vi "2D scan Tclk.vi"(0 "HW Config":T12={"SEM X coil"="SEM-X", "SEM Y coil"="SEM-Y", "Detectors"="Detectors", "Det min (V)"=-10.0, "Det max (V)"=10.0, "Eanable COM"=TRUE, "COM port"="COM1", "Detector FIB-NI auto switch"="FIB/port0/line0", "Machine Type"=0, "Machine ID"=""} {"Machine Type" items=["Feiss", "NVision"]}, 1 "Options":T9={"GetInfo"=TRUE, "Set Det A para"=TRUE, "Set WD"=FALSE, "Set Mag"=TRUE, "Set stig"=FALSE, "Set aln"=FALSE, "Display"=TRUE, "Save"=TRUE, "8-bit"=TRUE, "Detector A"=TRUE, "Detector B"=TRUE, "Detector C"=FALSE, "Detector D"=FALSE, "Inverse A"=FALSE, "Inverse B"=FALSE, "Inverse C"=FALSE, "Inverse D"=FALSE, "Inverse PNG"=FALSE, "Freeze"=TRUE, "PNG only"=FALSE, "Upload"=FALSE, "Delete after upload"=FALSE}, 2 "Frame":u8=1 min=1 step=1, 5 "Det Info":T11={"Brightness A"=40.0, "Contrast A"=26.0, "Detector B name"="ESB @ 1.0 kV", "Brightness B"=40.0, "Contrast B"=40.0, "Detector C name"="PMT @ 6.0", "Detector D name"="Detector D"}, 7 "Scan Para":T10={"X resolution"=4096, "Y resolution"=2048, "X center (um)"=0.0, "Y center (um)"=0.0, "X size (V)"=20.0, "X size auto"=TRUE, "X stig"=0.0, "Y stig"=0.0, "X aln"=0.0, "Y aln"=0.0, "Scan rate (Hz)"=10000000, "Oversampling"=10, "Oversampling auto"=TRUE, "Frame line rampdown ratio"=0.1, "Pixel size (nm)"=5.0, "WD"=4.0} {"WD" format="%#_7g"; "Frame line rampdown ratio" min=-1 max=1 step=0.05 format="%.2g"; "Scan rate (Hz)" max=4000000 format="%.2e"}, 9 "Focus Index Options":T2={"Keep aspect ratio"=FALSE, "X Grids"=1, "Y Grids"=1, "Primary X index"=1, "Primary Y index"=1}, 11 "File Info":T8={"File path"=path "E:/Images", "Notes"="", "Save recipe"=FALSE, "Load recipe"=FALSE, "Sample ID"=""}, 13 "Tile index":u8[](array[numeric])=[0, 0], 14 "Milling para":T1={"X resolution"=4096, "Y resolution"=125001, "X offset (um)"=0.0, "Y offset (um)"=0.0, "X center (um)"=0.0, "Y center (um)"=0.0, "X size (um)"=250.0, "Y size (um)"=250.0, "UL-Ang"=90.0, "UR-Ang"=90.0, "Line milling time (s)"=5.0, "Z-step (nm)"=2.0, "Lines auto pause"=1, "Auto pause"=FALSE, "Mill from Bottom"=FALSE, "FIB FOV (um)"=500.0, "Auto Profile"=FALSE, "Mill start from Last"=FALSE, "FIB PID on"=FALSE, "FIB PID reset"=TRUE, "FIB PID measured"=0, "FIB PID target"=0.0, "FIB PID target slope"=0.0, "FIB PID P"=0.001, "FIB PID I"=0.01, "FIB PID D"=0.0, "Emission (uA)"=1.36, "Suppressor (V)"=50.0, "Auto reheat"=FALSE} caption="Milling Parameters" {"Suppressor (V)" step=0.1 format="%.1g"; "Emission (uA)" step=0.1 format="%.2g"; "FIB PID measured" items=["Spec.", "B.D. 1", "B.D. 2", "Mill", "Spec. +"]; "FIB PID target slope" min=-1 max=1 step=0.1; "UR-Ang" format="%.2f"; "UL-Ang" format="%.2f"; "Y offset (um)" step=0.02 format="%.3g"; "X offset (um)" step=1 format="%.3g"; "FIB FOV (um)" format="%.3g"; "Line milling time (s)" format="%.1f"; "Y center (um)" format="%#.3g"; "X center (um)" format="%#.3g"}) -> (3 "Image Focus Index Array":T3, 4 "Info & Status":T7={"AO SampClk.MaxRate"=100000000.0, "AI SampClk.MaxRate"=100000000.0, "AO rate"=10000000.0, "Scan speed"=1, "Detector number"=2, "X min (V)"=-10.0, "X max (V)"=10.0, "X min index"=0, "X max index"=4095, "AO multiline"=128, "Decimating factor"=8, "AvailSampPerChan"=6177088, "AO scan line"=2048, "Total pixels recorded"=8388608, "Total lines scanned"=2048, "Scan time (m)"=0.0, "Scan time (s)"=0.9240575999999999, "Remaining time (m)"=0, "Remaining time (s)"=0, "Specimen I (nA)"=0.0, "Frame"=1, "X tile"=0, "Y tile"=0} {"Frame" min=1 step=1; "Y tile" min=1; "X tile" min=1; "Specimen I (nA)" format="%#.2g"; "AvailSampPerChan" scale=0.0..32000000.0; "Scan time (s)" format="%.3f"; "Total pixels recorded" scale=0.0..250000.0; "Scan speed" scale=1.0..15.0; "AO rate" format="%#_3e"}, 6 "SEM parameters":T5={"Detector A"="Det A", "Detector B"="ESB @ 1.0 kV", "Brightness A"=40.0, "Contrast A"=26.0, "Brightness B"=40.0, "Contrast B"=40.0, "Magnification"=5582.6, "Pixel size"=5.0, "Working distance"=4.0, "EHT"=0.0, "Aperture"=0, "High current mode"=0, "Probe current"=0.0, "Scan rotation"=0.0, "Chamber vac"=0.0, "Gun vac"=0.0, "Beam shift X"=0.0, "Beam shift Y"=0.0, "Stig X"=0.0, "Stig Y"=0.0, "Alignment X"=0.0, "Alignment Y"=0.0, "Stage X"=0.0, "Stage Y"=0.0, "Stage Z"=0.0, "Stage T"=0.0, "Stage R"=0.0, "Stage M"=0.0}, 8 "8-bit over scale":bool[](array[boolean]), 10 "FIB parameters":T6, 15 "Image Focus Index":T4)   [LabVIEW 2018]
uses:
  <vilib>/Utility/error.llb/DialogType.ctl
  <vilib>/DAQmx/write.llb/DAQmx Write (Digital Bool 1Line 1Point).vi
  <vilib>/Analysis/2dsp.llb/Decimate (single shot, DBL).vi
  <vilib>/DAQmx/create/channels.llb/DAQmx Create Channel (DO-Digital Output).vi
  <vilib>/DAQmx/miscellaneous.llb/DAQmx Fill In Error Info.vi
  <instrlib>/niScope/Acquire/niScope Get Scaling Coefficients.vi
  <instrlib>/niFgen/niFgen.llb/niFgen Write Waveform.vi
  <instrlib>/niScope/Acquire/Fetch/niScope Multi Fetch Binary 16.vi
  <vilib>/measure/madcrms.llb/Basic Averaged DC-RMS for 1 Chan.vi
  <vilib>/regexp/Match Regular Expression.xnode
  <vilib>/Analysis/NI_AALPro.lvlib
  <vilib>/measure/NI_MAPro.lvlib
panel:
  in  "Api":refnum<k7>(container)
  in  "Force tclk init":bool
  out "DetB-Scaling":sgl
  out "DetA-Scaling":sgl
  out "DetB-Rate":sgl
  out "DetA-Rate":sgl
  out "8-bit coefficents":sgl[][](array[numeric])
  out "DetC-Io":sgl
  out "DetC-k":sgl
  out "DetD-Io":sgl
  out "DetD-k":sgl
  out "DetB-k":sgl
  out "DetB-Io":sgl
  out "DetA-k":sgl
  out "DetA-Io":sgl
  out "8-bit":bool=TRUE
  out "Screen pixel factor":dbl=0.25
  out "Mag":dbl=5582.6
  out "Runsheet header array":string[](array[string])=["Date", "Time", "Notes", "Detector A", "Detector B", "Detector C", "Detector D", "Detectors", "X resolution", "Y resolution", "Rate (Hz)", "Brightness A (%)", "Contrast A (%)", "Brightness B (%)", "Contrast B (%)", "Magnification", "Pixel size (nm)", "Working Distance (mm)", "EHT (kV)", "Aperture #", "High Current Mode", "Probe Current (A)", "Beam Shift X", "Beam Shift Y", "Stigmation X", "Stigmation Y", "Alignment X", "Alignment Y", "FIB spacing (nm)", "A Img Focus Index", "B Img Focus Index", "C Img Focus Index", "D Img Focus Index", "Temp (F)", "FIB Faraday Cup (nA)", "Specimen I (nA)", "Milling Beam Dump (nA)", "Milling Y voltage (V)", "SEM Specimen I (nA)", "Image Delta X (pix)", "Image Delta Y (pix)", "Image Delta Z"]
  out "Set aln":bool
  out "X aln":sgl
  out "Y aln":sgl
  out "FI scaling":u8=1
  in  "SEM Spec. I (nA)":sgl format="%#.2g"
  out "SW date":string
  out "Image bits":u8=16
  out "error out":errorcluster
  out "Delete after upload":bool
  in  "FI Detector":u16(ring) caption="Detector" items=["A", "B", "C", "D"]
  out "keep aspect ratio":bool=TRUE
  out "Primary Y index":u8 caption="Primary Y"
  out "Primary X index":u8 caption="Primary X"
  out "Y Grids":u8=1
  out "X Grids":u8=1
  out "Timestamp":timestamp=timestamp(3479292891.7167473 s since 1904-01-01)
  out "Upload flags path":path
  out "Upload":bool=TRUE
  out "Sample ID":string
  out "Machine ID":string
  out "Eanable COM":bool
  out "PNG only":bool=TRUE
  out "Eval D":i16[][](graph)
  out "Eval C":i16[][](graph)
  out "Eval B":i16[][](graph)
  out "Eval A":i16[][](graph)
  out "Freeze":bool=TRUE
  out "Detector FIB-NI auto switch":tag="FIB/port0/line0"
  out "GetInfo":bool=TRUE
  out "Set stig":bool
  out "Y stig":sgl
  out "X stig":sgl
  in  "Total time":dbl=0.9240575999999999
  in  "stop":bool=TRUE
  out "Det max (V)":dbl=10.0
  out "Det min (V)":dbl=-10.0
  in  "AvailSampPerChan":u32(slide)=6177088 scale=0.0..1000000.0
  in  "AO scan line":u32=2048
  in  "AO multiline":u32=128
  in  "Decimating factor":u16=8
  in  "Remaining time (m)":u16
  in  "Remaining time (s)":u8
  in  "Scan time (s)":dbl=0.9240575999999999 format="%.3f"
  in  "Scan time (m)":dbl
  in  "Total lines scanned":i32=2048
  in  "Total pixels recorded":i32(slide)=8388608 scale=-1.0..1048576.0
  in  "X max (V)":dbl=10.0
  in  "X min (V)":dbl=-10.0
  in  "X min index":i32
  in  "X max index":i32=4095
  in  "Scan speed":u8(slide)=1 scale=1.0..15.0
  in  "AO rate":dbl=10000000.0 caption="Scanning rate" format="%#_3e"
  in  "Detector number":u8=2
  in  "AI SampClk.MaxRate":dbl=100000000.0
  in  "AO SampClk.MaxRate":dbl=100000000.0
  out "Det A Img":i16[][](graph)
  out "Det B Img":i16[][](graph)
  out "Det C Img":i16[][](graph)
  out "Det D Img":i16[][](graph)
  out "Notes":string
  out "File path":path=path "E:/Images"
  out "Inverse PNG":bool
  out "Inverse D":bool
  out "Inverse C":bool
  out "Inverse B":bool
  out "Inverse A":bool
  out "Detector D":bool
  out "Detector C":bool
  out "Detector B":bool=TRUE
  out "Detector A":bool=TRUE
  out "Save":bool=TRUE
  out "Display":bool=TRUE
  out "Set Mag":bool=TRUE
  out "Set WD":bool
  out "Set Det A para":bool=TRUE
  out "WD":sgl=4.0
  out "Pixel size (nm)":sgl=5.0
  out "Frame line rampdown ratio":sgl=0.1
  out "Oversampling":u32=10
  out "Scan rate (Hz)":u32=10000000
  out "Y resolution":u32=2048
  out "X resolution":u32=4096
  out "Detector D name":string="Detector D"
  out "Detector C name":string="PMT @ 6.0"
  out "Contrast B":dbl=40.0
  out "Brightness B":dbl=40.0
  out "Detector B name":string="ESB @ 1.0 kV"
  out "Contrast A":dbl=26.0
  out "Brightness A":dbl=40.0
  out "COM port":refnum<visa-resource-name>="COM1"
  out "File name":path=path "E:/Images/Y2014/M04/D02/_14-04-02_091451_0-0.dat"
  # "Hardware Configuration"
  # "Detectors Information"
  # "Scanning Parameters"
  # "Direction"
  # "Start\nfrom"
  # "<"
  # "Hz"
  # "Scanning time"
  # "m"
  # "s"
  # "Remaining time"
  # "m"
  # "s"
  # "Det"
  # "Detector A"
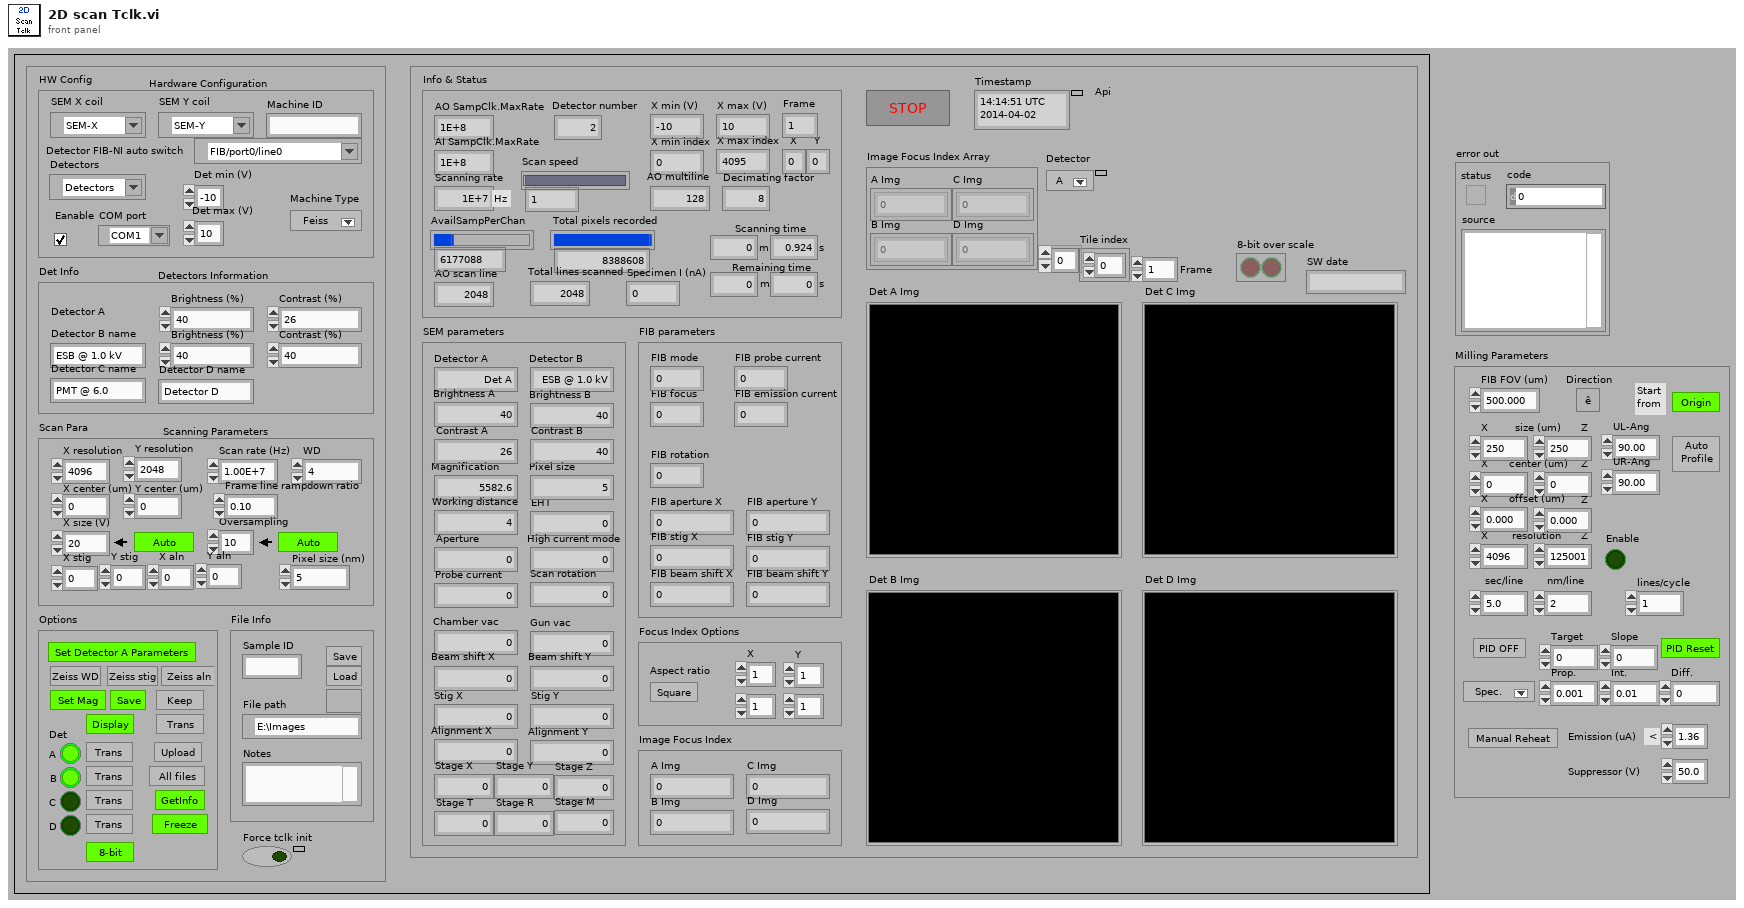
[diagram p1: front panel]
types:
  T1 = cluster{"X resolution":u32, "Y resolution":u32, "X offset (um)":sgl, "Y offset (um)":sgl, "X center (um)":sgl, "Y center (um)":sgl, "X size (um)":sgl, "Y size (um)":sgl, "UL-Ang":sgl, "UR-Ang":sgl, "Line milling time (s)":sgl, "Z-step (nm)":dbl, "Lines auto pause":u16, "Auto pause":bool, "Mill from Bottom":bool, "FIB FOV (um)":sgl, "Auto Profile":bool, "Mill start from Last":bool, "FIB PID on":bool, "FIB PID reset":bool, "FIB PID measured":u8, "FIB PID target":sgl, "FIB PID target slope":sgl, "FIB PID P":sgl, "FIB PID I":sgl, "FIB PID D":sgl, "Emission (uA)":dbl, "Suppressor (V)":sgl, "Auto reheat":bool}
  T2 = cluster{"Keep aspect ratio":bool, "X Grids":u8, "Y Grids":u8, "Primary X index":u8, "Primary Y index":u8}
  T3 = cluster{"A Img Focus Index array":sgl[][], "B Img Focus Index array":sgl[][], "C Img Focus Index array":sgl[][], "D Img Focus Index array":sgl[][]}
  T4 = cluster{"A Img Focus Index":sgl, "B Img Focus Index":sgl, "C Img Focus Index":sgl, "D Img Focus Index":sgl}
  T5 = cluster{"Detector A":string, "Detector B":string, "Brightness A":sgl, "Contrast A":sgl, "Brightness B":sgl, "Contrast B":sgl, "Magnification":sgl, "Pixel size":sgl, "Working distance":sgl, "EHT":sgl, "Aperture":u8, "High current mode":u8, "Probe current":sgl, "Scan rotation":sgl, "Chamber vac":sgl, "Gun vac":sgl, "Beam shift X":sgl, "Beam shift Y":sgl, "Stig X":sgl, "Stig Y":sgl, "Alignment X":sgl, "Alignment Y":sgl, "Stage X":sgl, "Stage Y":sgl, "Stage Z":sgl, "Stage T":sgl, "Stage R":sgl, "Stage M":sgl}
  T6 = cluster{"FIB mode":u8, "FIB focus":sgl, "FIB probe current":sgl, "FIB emission current":sgl, "FIB rotation":sgl, "FIB aperture X":sgl, "FIB aperture Y":sgl, "FIB stig X":sgl, "FIB stig Y":sgl, "FIB beam shift X":sgl, "FIB beam shift Y":sgl}
  T7 = cluster{"AO SampClk.MaxRate":dbl, "AI SampClk.MaxRate":dbl, "AO rate":dbl, "Scan speed":u8, "Detector number":u8, "X min (V)":dbl, "X max (V)":dbl, "X min index":i32, "X max index":i32, "AO multiline":u32, "Decimating factor":u16, "AvailSampPerChan":u32, "AO scan line":u32, "Total pixels recorded":i32, "Total lines scanned":i32, "Scan time (m)":dbl, "Scan time (s)":dbl, "Remaining time (m)":u16, "Remaining time (s)":u8, "Specimen I (nA)":sgl, "Frame":u8, "X tile":u8, "Y tile":u8}
  T8 = cluster{"File path":path, "Notes":string, "Save recipe":bool, "Load recipe":bool, "Sample ID":string}
  T9 = cluster{"GetInfo":bool, "Set Det A para":bool, "Set WD":bool, "Set Mag":bool, "Set stig":bool, "Set aln":bool, "Display":bool, "Save":bool, "8-bit":bool, "Detector A":bool, "Detector B":bool, "Detector C":bool, "Detector D":bool, "Inverse A":bool, "Inverse B":bool, "Inverse C":bool, "Inverse D":bool, "Inverse PNG":bool, "Freeze":bool, "PNG only":bool, "Upload":bool, "Delete after upload":bool}
  T10 = cluster{"X resolution":u32, "Y resolution":u32, "X center (um)":sgl, "Y center (um)":sgl, "X size (V)":dbl, "X size auto":bool, "X stig":sgl, "Y stig":sgl, "X aln":sgl, "Y aln":sgl, "Scan rate (Hz)":u32, "Oversampling":u32, "Oversampling auto":bool, "Frame line rampdown ratio":sgl, "Pixel size (nm)":sgl, "WD":sgl}
  T11 = cluster{"Brightness A":dbl, "Contrast A":dbl, "Detector B name":string, "Brightness B":dbl, "Contrast B":dbl, "Detector C name":string, "Detector D name":string}
  T12 = cluster{"SEM X coil":refnum<k15>, "SEM Y coil":refnum<k15>, "Detectors":refnum<k15>, "Det min (V)":dbl, "Det max (V)":dbl, "Eanable COM":bool, "COM port":refnum<visa-resource-name>, "Detector FIB-NI auto switch":tag, "Machine Type":u8, "Machine ID":string}
  T13 = cluster{"AO SampClk.MaxRate":dbl, "AI SampClk.MaxRate":dbl, "AO rate":dbl, "Scan speed":u8, "Detector number":u8, "X min (V)":dbl, "X max (V)":dbl, "X min index":i32, "X max index":i32, "AO multiline":u32, "Decimating factor":u16, "AvailSampPerChan":u32, "AO scan line":u32, "Total pixels recorded":i32, "Total lines scanned":i32, "Scan time (m)":dbl, "Scan time (s)":dbl, "Remaining time (m)":u16, "Remaining time (s)":u8, "SEM Spec. I (nA)":sgl, "Frame":u8, u8, u8}
  T14 = enum16{"SEM", "FIB", "Milling", "SEM + FIB", "Mill + SEM", "SEM Drift Correction", "FIB Drift Correction", "No Beam", "External", "External + SEM"}
  T15 = enum16{"Initialize Reference", "Get Reference", "Close Reference"}
  T16 = enum16{"open", "replace", "create", "open or create", "replace or create", "replace or create with confirmation"}
  T17 = typedef "DialogType.ctl" = u16
  T18 = cluster{"FIB mode":u8, "FIB focus":sgl, "FIB probe current":u8, "FIB emission current":sgl, "FIB rotation":sgl, "FIB aperture X":sgl, "FIB aperture Y":sgl, "FIB stig X":sgl, "FIB stig Y":sgl, "FIB beam shift X":sgl, "FIB beam shift Y":sgl}
  T19 = cluster{"Latest 8-bit coefficients[0]":sgl, "Latest 8-bit coefficients[1]":sgl, "Latest 8-bit coefficients[2]":sgl, "Latest 8-bit coefficients[3]":sgl, "Latest 8-bit coefficients[4]":sgl, "Latest 8-bit coefficients[5]":sgl, "Latest 8-bit coefficients[6]":sgl, "Latest 8-bit coefficients[7]":sgl}
  T20 = cluster{"sessions out":refnum<k20>[], "SEM-X handle out":refnum<k15>, "SEM-Y handle out":refnum<k15>, "SEM-Y waveform handle out":i32, "Detectors handle out":refnum<k15>, "channels":string, "error out":errorcluster, "Others":cluster{"AO SampClk.MaxRate":dbl, "AI SampClk.MaxRate":dbl, "AO rate":dbl, "Scan speed":u8, "Detector number":u8, "X min (V)":dbl, "X max (V)":dbl, "X min index":i32, "X max index":i32, "Y min (V)":dbl, "Y max (V)":dbl, "AO multiline":u32, "Decimating factor":u16, "Total time":dbl, "Scan time (m)":dbl, "Scan time (s)":dbl, "X resolution":u32, "Y resolution":u32, "X resolution with rampdown":i32, "Oversampling":u32, "Y scan pts per line":i32, "Y scan pts per AO multiline":i32, "Small scan":bool, "Y single line pattern":dbl[], "Detectors min record length":u32, "Waveform blocks":u32, "Repeat count":u32, "Waveform size":u32, "AI multiline":u16}}
  T21 = cluster{"offset":dbl, "gain":dbl, "reserved 1":dbl, "reserved 2":dbl}[]
  T22 = cluster{"offset":sgl, "gain":sgl, "reserved 1":sgl, "reserved 2":sgl}[]
  T23 = cluster{"Detector A":bool, "Detector B":bool, "Detector C":bool, "Detector D":bool}
  T24 = cluster{"Detector C name":string, "Detector D name":string}
  T25 = cluster{"X resolution":u32, "Y resolution":u32, "Oversampling":u32, "Scan speed":u8, "AO rate":dbl, "Frame line rampdown ratio":sgl, "X min (V)":dbl, "X max (V)":dbl, "Det min (V)":dbl, "Det max (V)":dbl}
  T26 = cluster{"A Img Focus Index array":dbl[][], "B Img Focus Index array":dbl[][], "C Img Focus Index array":dbl[][], "D Img Focus Index array":dbl[][]}
  T27 = cluster{"A Img Focus Index":dbl, "B Img Focus Index":dbl, "C Img Focus Index":dbl, "D Img Focus Index":dbl}
  T28 = cluster{"Single":sgl, "Single":sgl, "Single":sgl, "Single":sgl, "Single":sgl, "Single":sgl, "SEM Spec. I (nA)":sgl, "Single":sgl, "D Img Focus Index":dbl, "UInt32":u32}
  T29 = cluster{dbl, "8-bit":bool, "8-bit coefficents":sgl[][], cluster{"Detector A":bool, "Detector B":bool, "Detector C":bool, "Detector D":bool}, cluster{"X resolution":u32, "Y resolution":u32, "Oversampling":u32, "Scan speed":u8, "AO rate":dbl, "Frame line rampdown ratio":sgl, "X min (V)":dbl, "X max (V)":dbl, "Det min (V)":dbl, "Det max (V)":dbl}, "Decimating factor":u16, "Notes":string, cluster{"Detector C name":string, "Detector D name":string}, "SEM parameters":cluster{"Detector A":string, "Detector B":string, "Brightness A":sgl, "Contrast A":sgl, "Brightness B":sgl, "Contrast B":sgl, "Magnification":sgl, "Pixel size":sgl, "Working distance":sgl, "EHT":sgl, "Aperture":u8, "High current mode":u8, "Probe current":sgl, "Scan rotation":sgl, "Chamber vac":sgl, "Gun vac":sgl, "Beam shift X":sgl, "Beam shift Y":sgl, "Stig X":sgl, "Stig Y":sgl, "Alignment X":sgl, "Alignment Y":sgl, "Stage X":sgl, "Stage Y":sgl, "Stage Z":sgl, "Stage T":sgl, "Stage R":sgl, "Stage M":sgl}, "FIB parameters":cluster{"FIB mode":u8, "FIB focus":sgl, "FIB probe current":sgl, "FIB emission current":sgl, "FIB rotation":sgl, "FIB aperture X":sgl, "FIB aperture Y":sgl, "FIB stig X":sgl, "FIB stig Y":sgl, "FIB beam shift X":sgl, "FIB beam shift Y":sgl}, "Milling para":cluster{"X resolution":u32, "Y resolution":u32, "X offset (um)":sgl, "Y offset (um)":sgl, "X center (um)":sgl, "Y center (um)":sgl, "X size (um)":sgl, "Y size (um)":sgl, "UL-Ang":sgl, "UR-Ang":sgl, "Line milling time (s)":sgl, "Z-step (nm)":dbl, "Lines auto pause":u16, "Auto pause":bool, "Mill from Bottom":bool, "FIB FOV (um)":sgl, "Auto Profile":bool, "Mill start from Last":bool, "FIB PID on":bool, "FIB PID reset":bool, "FIB PID measured":u8, "FIB PID target":sgl, "FIB PID target slope":sgl, "FIB PID P":sgl, "FIB PID I":sgl, "FIB PID D":sgl, "Emission (uA)":dbl, "Suppressor (V)":sgl, "Auto reheat":bool}, "Machine ID":string, cluster{"Single":sgl, "Single":sgl, "Single":sgl, "Single":sgl, "Single":sgl, "Single":sgl, "SEM Spec. I (nA)":sgl, "Single":sgl, "D Img Focus Index":dbl, "UInt32":u32}}
  T30 = typedef "imagedata.ctl" = cluster{"image type":i32, "image depth":i32, "image":u8[], "mask":u8[], "colors":u32[], "Rectangle":cluster{"left":i16, "top":i16, "right":i16, "bottom":i16}}
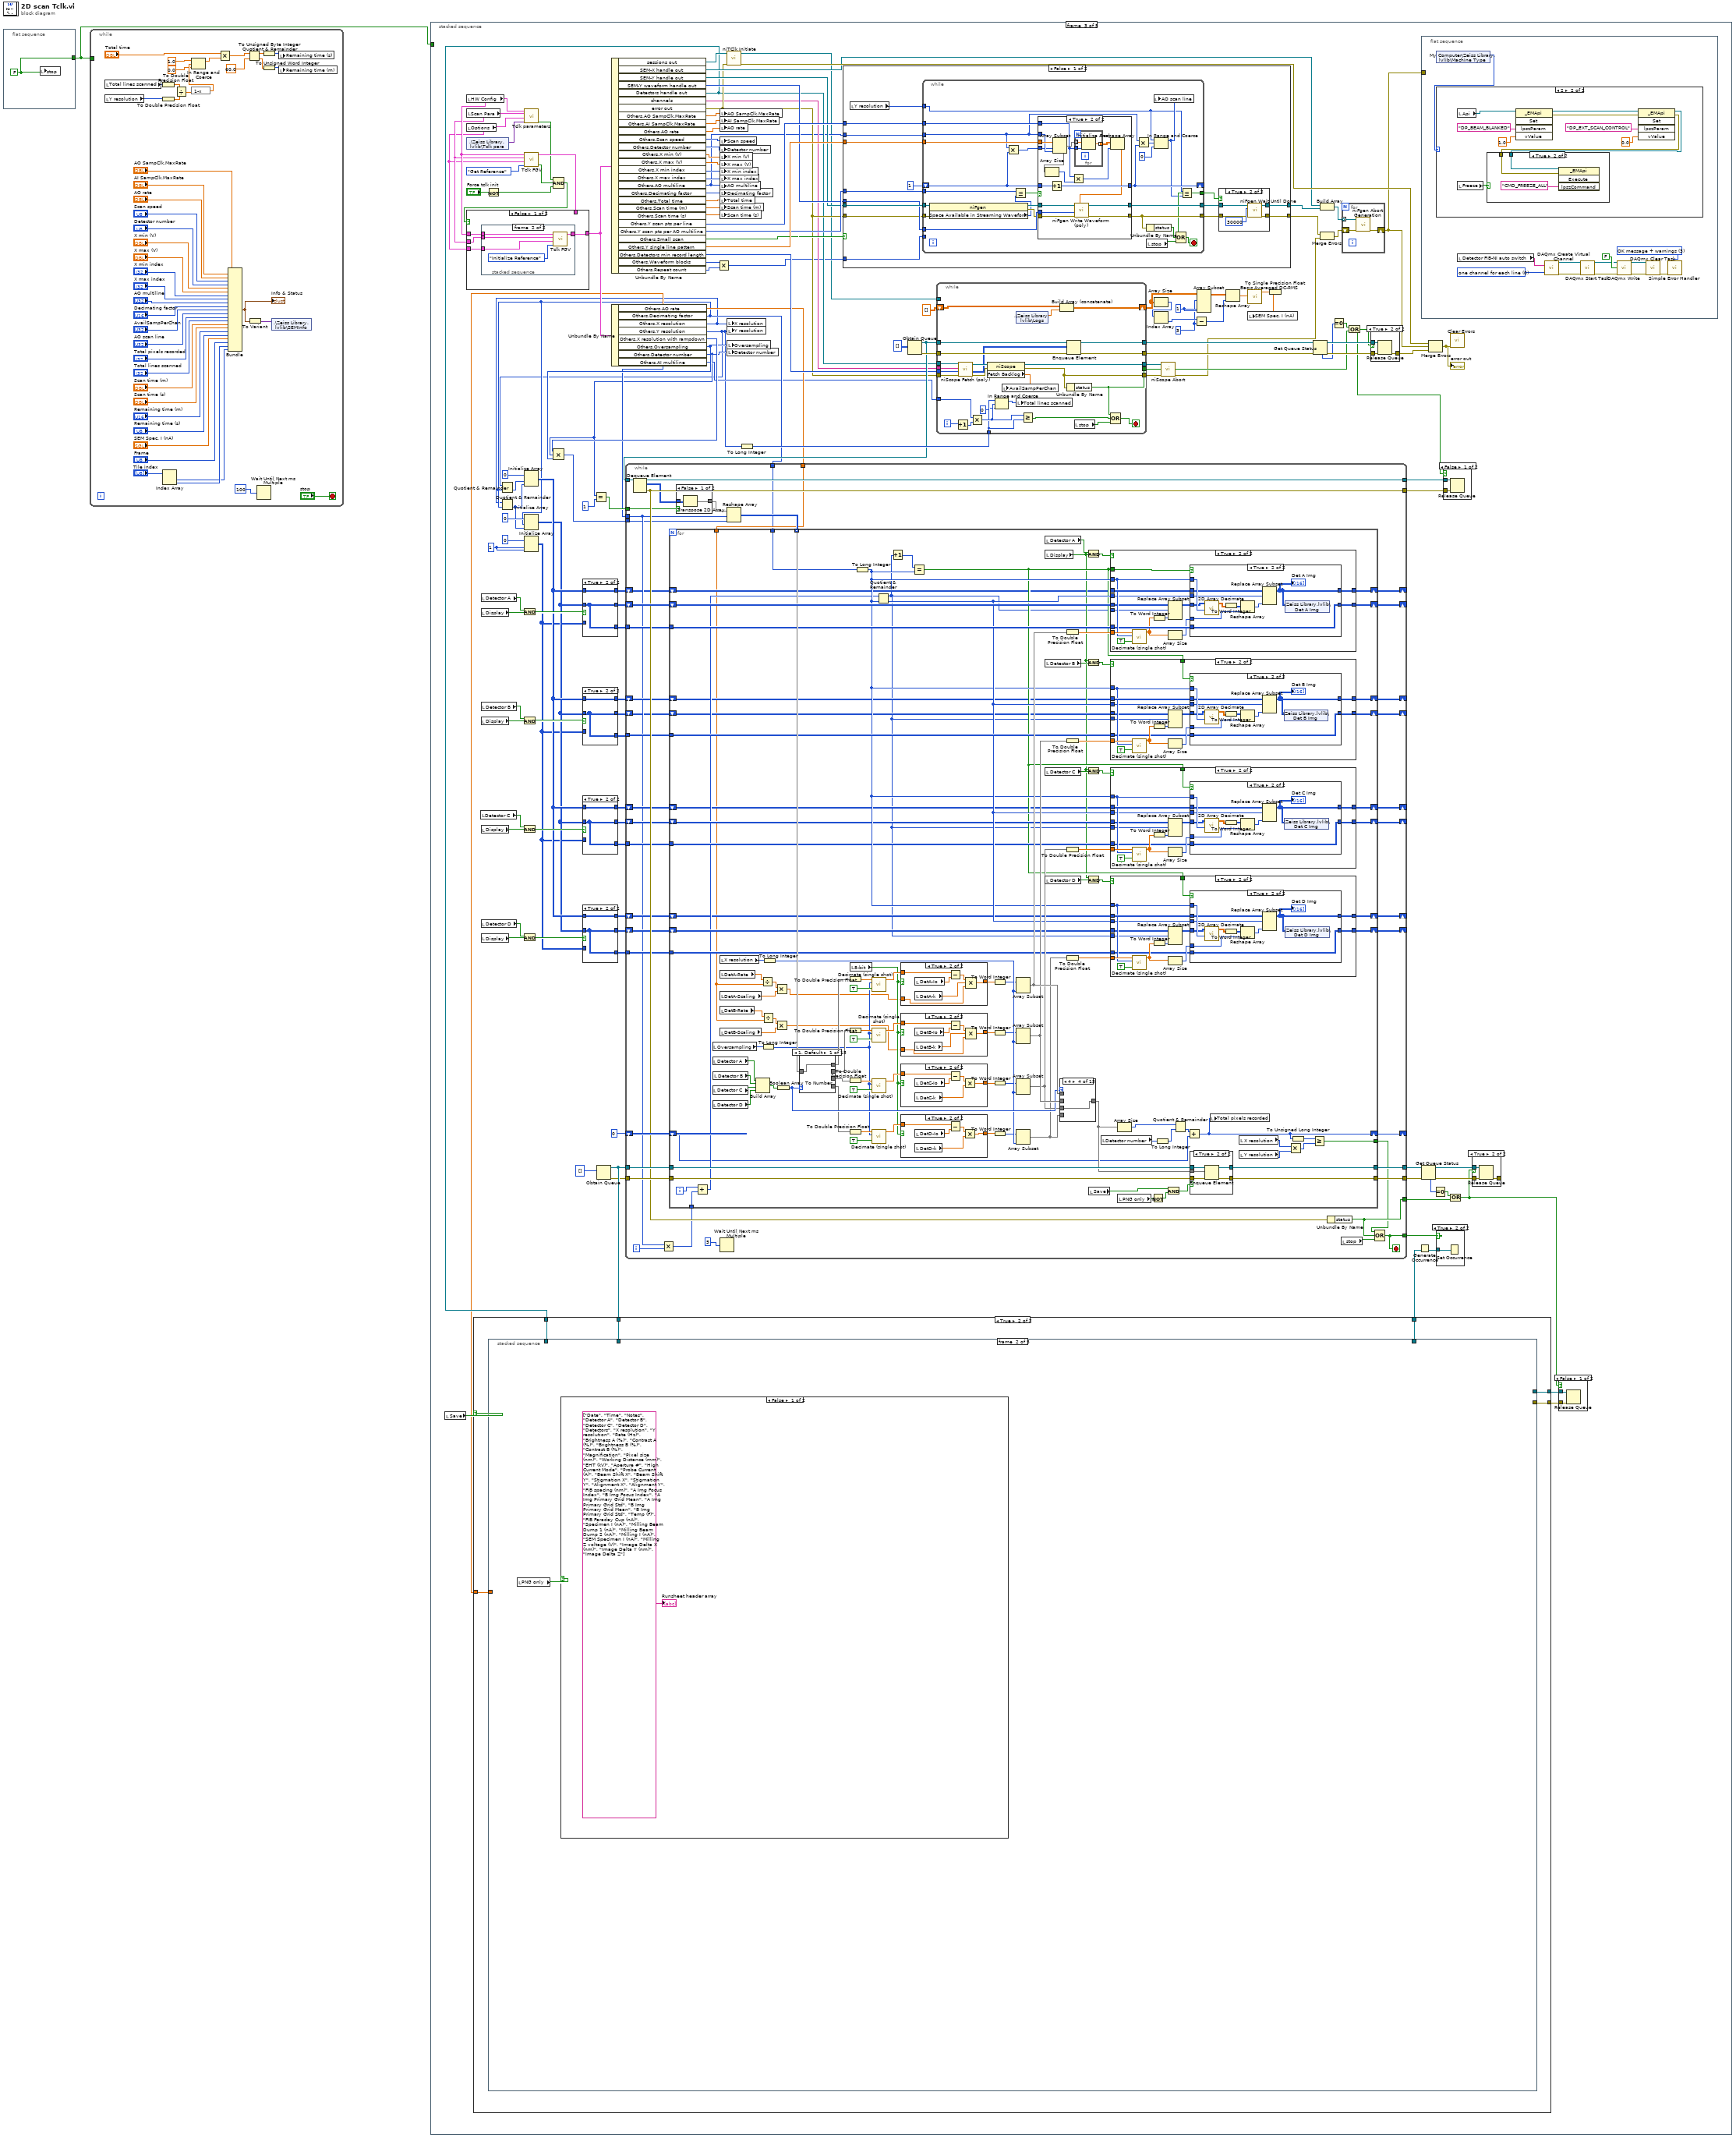
[diagram p0: block diagram]
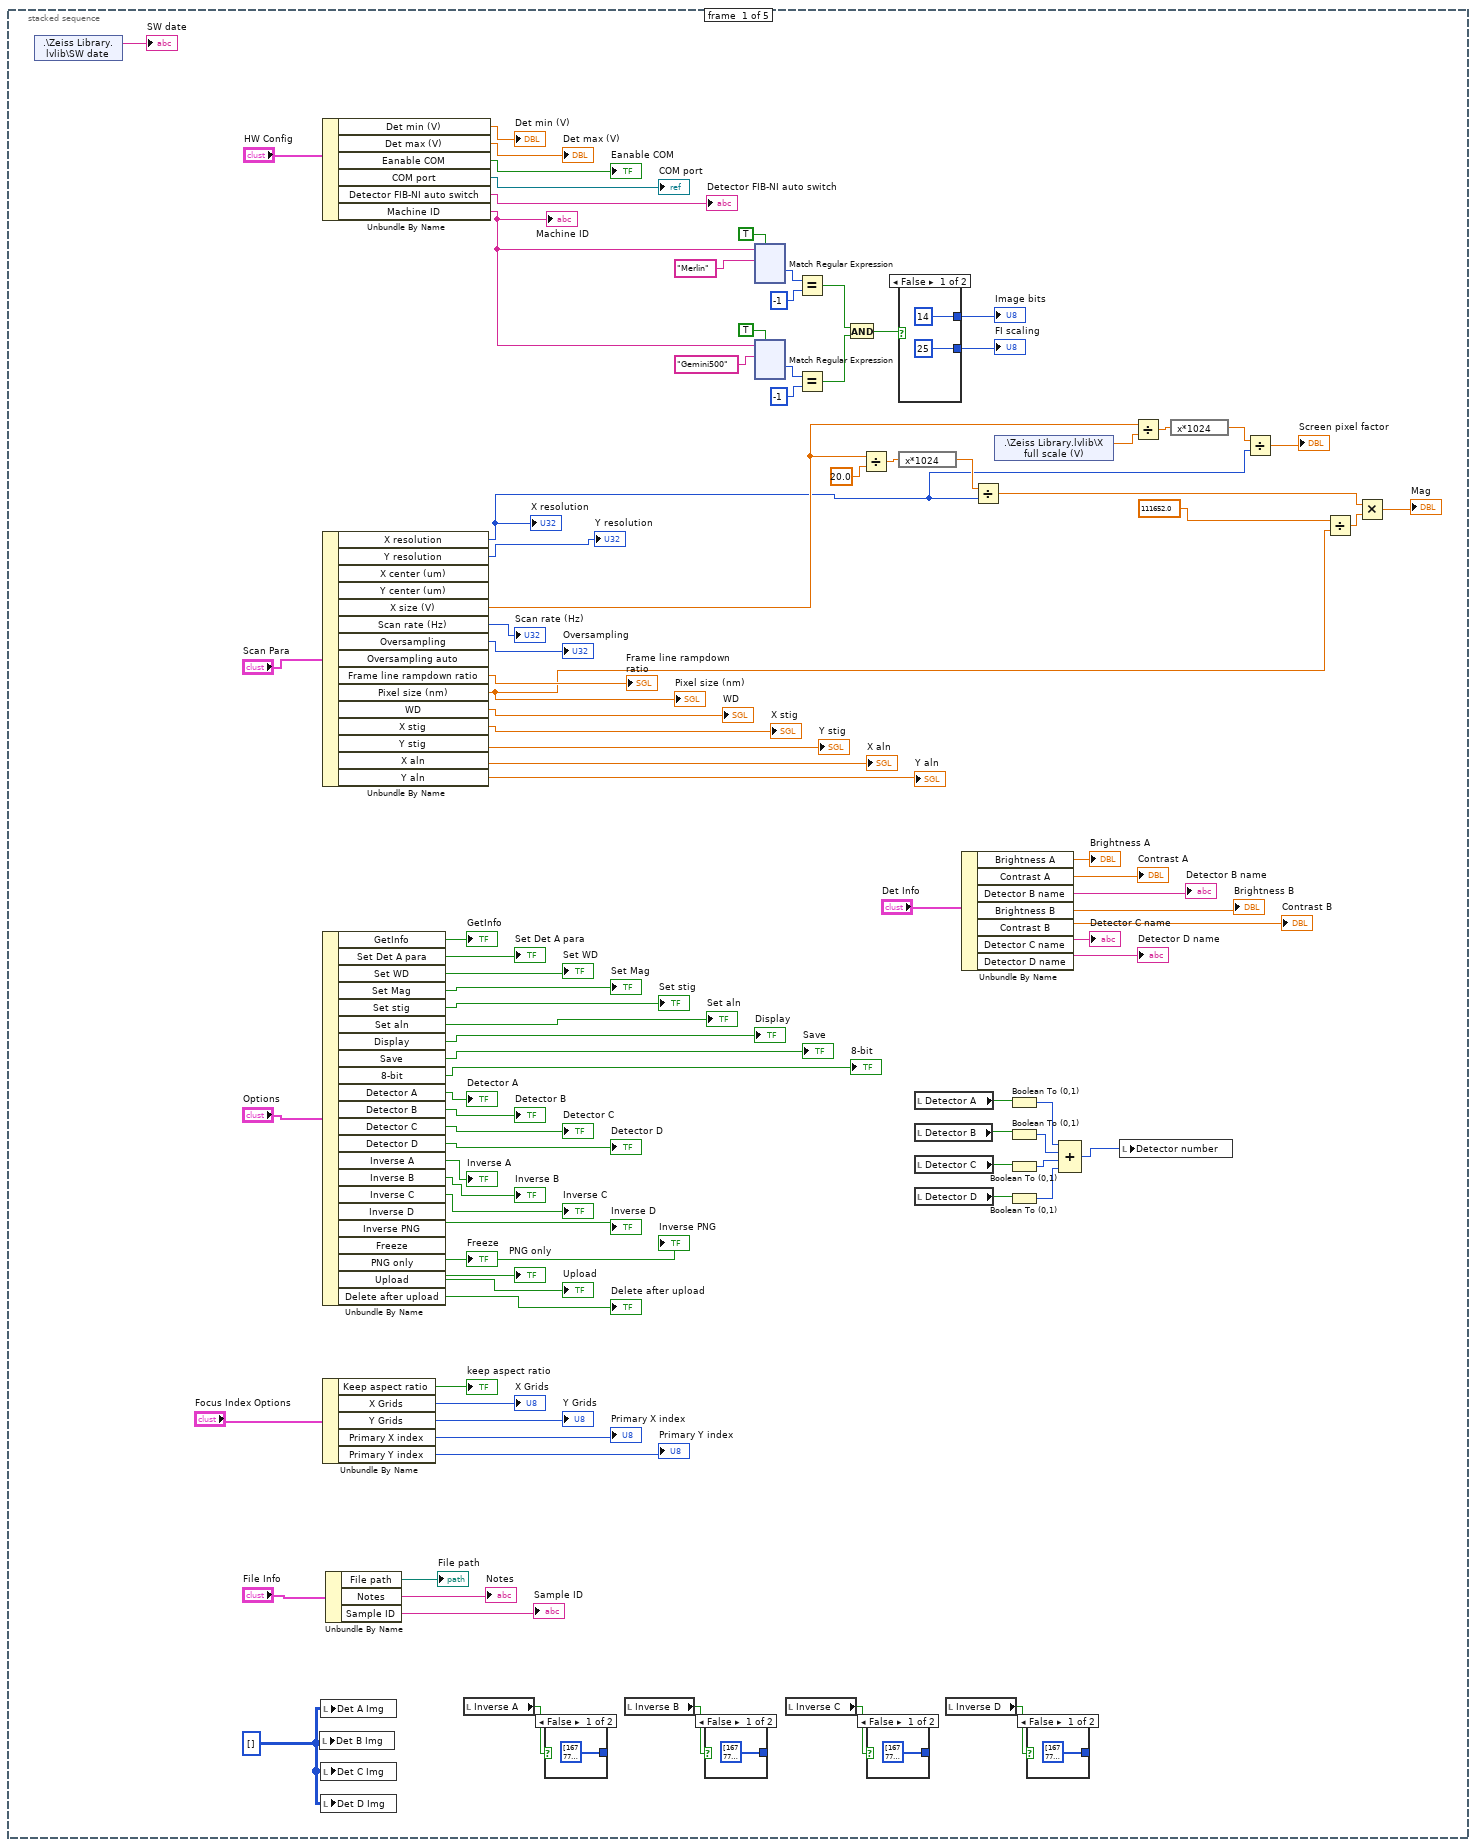
[diagram p2: hidden frame]
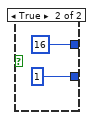
[diagram p3: hidden frame]
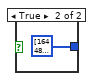
[diagram p4: hidden frame]
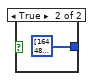
[diagram p5: hidden frame]
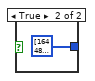
[diagram p6: hidden frame]
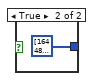
[diagram p7: hidden frame]
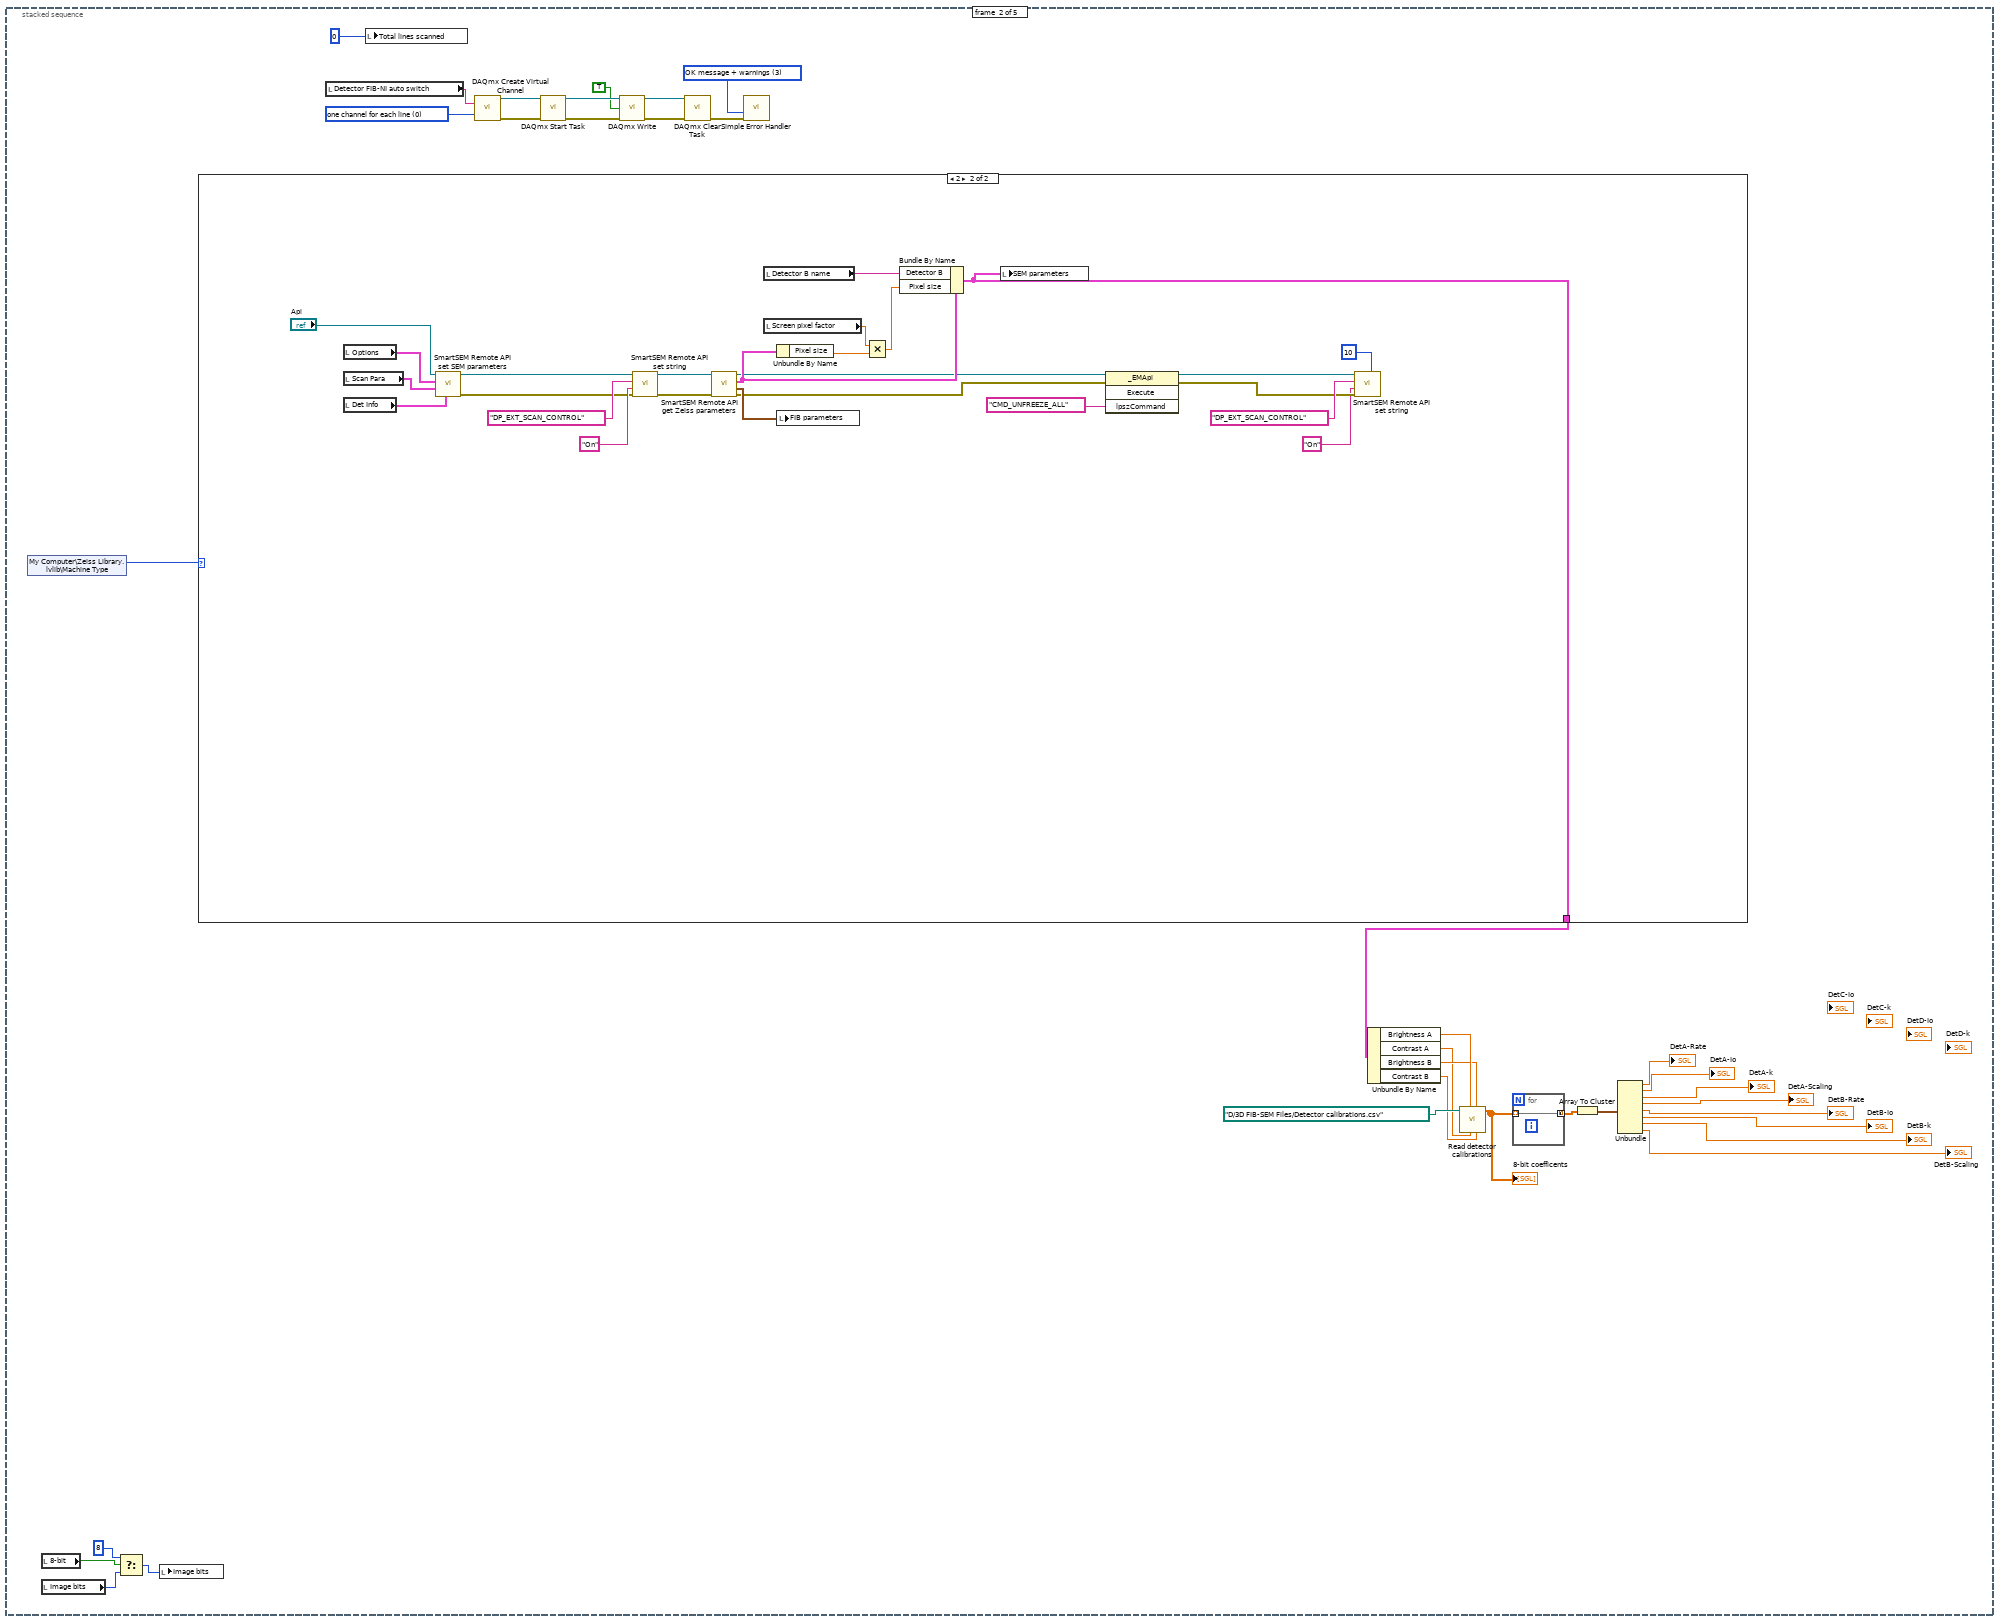
[diagram p8: hidden frame]
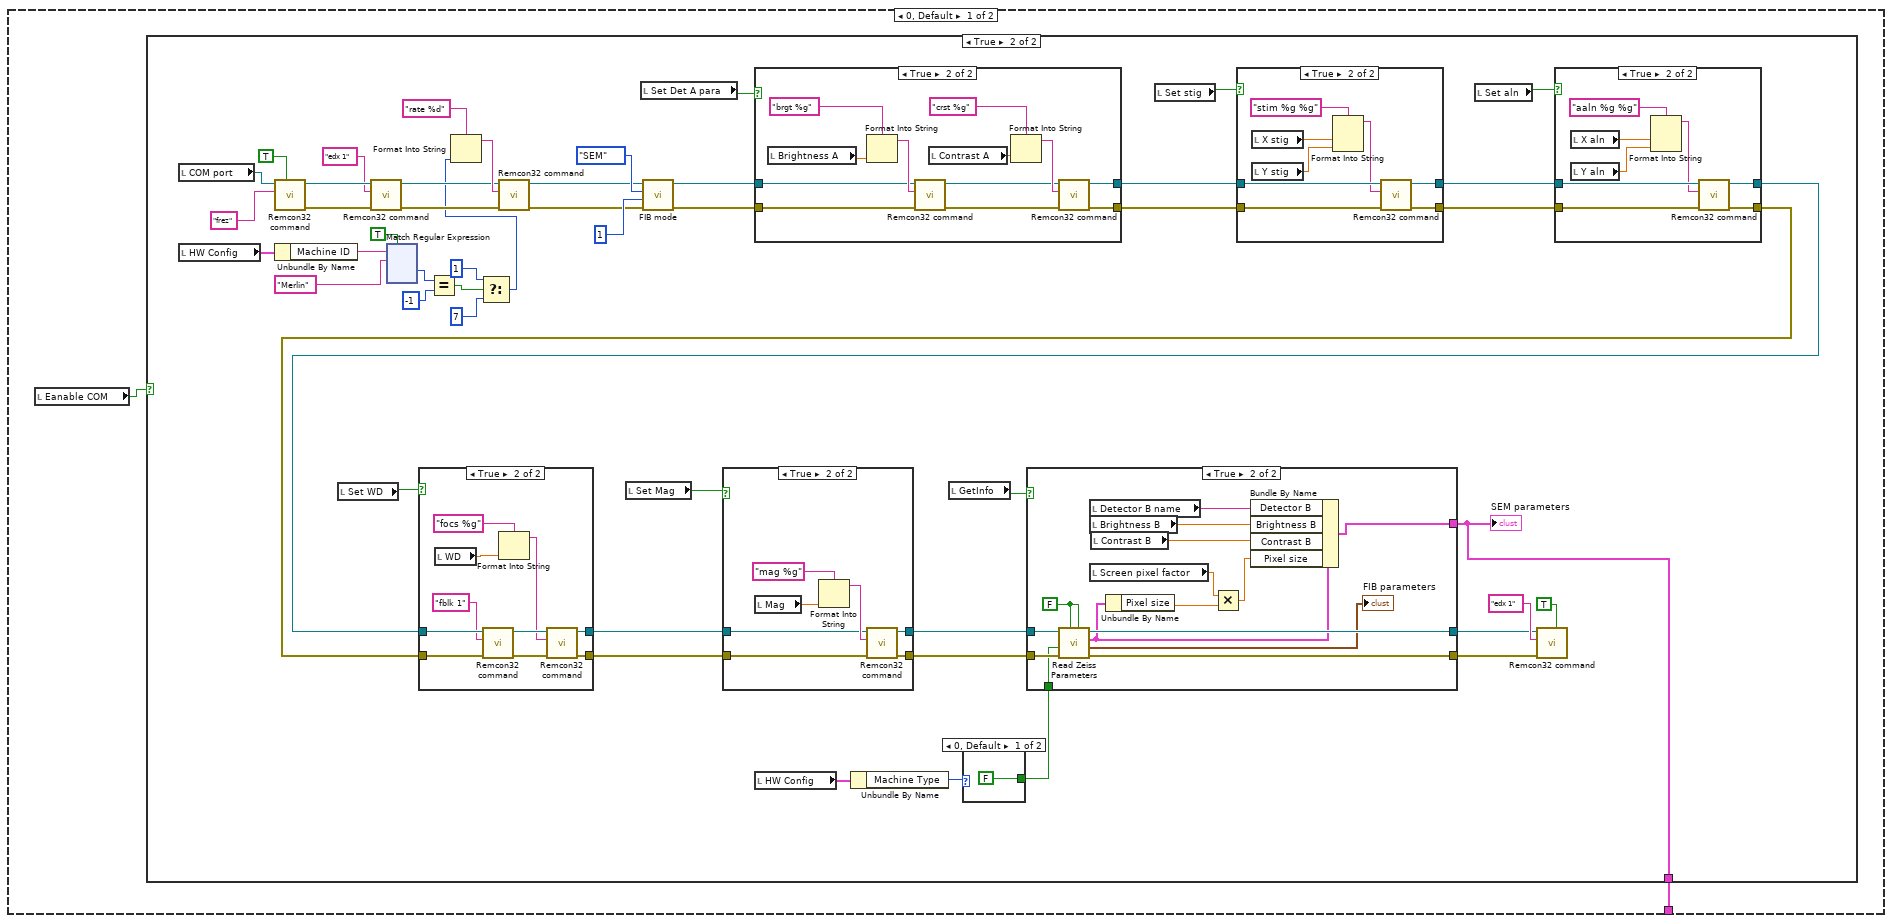
[diagram p9: hidden frame]
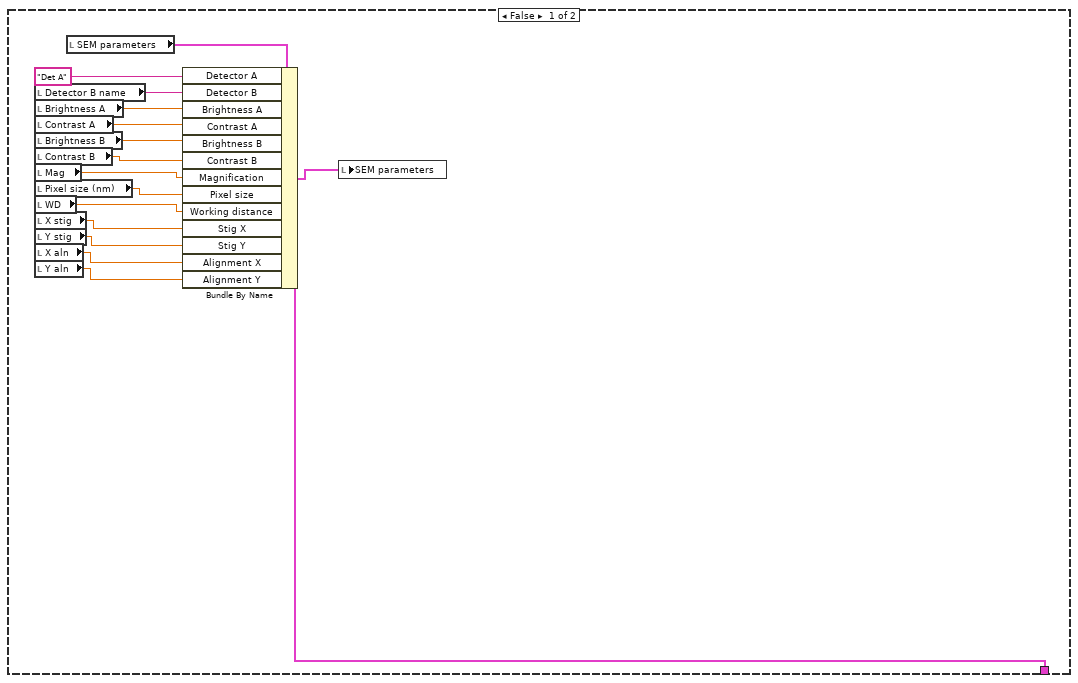
[diagram p10: hidden frame]
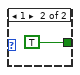
[diagram p12: hidden frame]
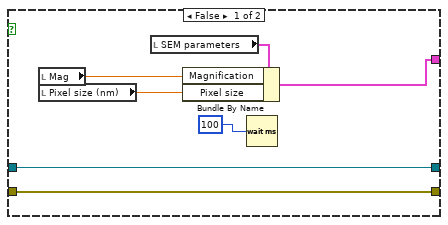
[diagram p13: hidden frame]
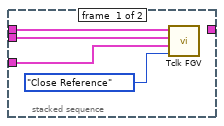
[diagram p18: hidden frame]
diagram:
  n1 = flat-sequence {
    tunnel: [w2] -> w1
    frame #0 {
      w2 = FALSE ("stop")
      n2 = local write "stop"(w2) -> ()
    }
  }
  n3 = while {
    tunnel: w1 -> [_]
    stop <- "stop" stop-if-true
    n4 = local read "Total lines scanned"() -> (w27:i32)
    n5 = local read "Y resolution"() -> (w16:u32)
    n6 = To Double Precision Float(number=w27) -> (double precision float=w20:dbl)
    n7 = To Double Precision Float(number=w16) -> (double precision float=w21:dbl)
    n8 = Index Array(array="Tile index") -> (element #1=w6:u8, element #2=w7:u8)  [unwired: 2 in]
    n9 = Divide(x=w20, y=w21) -> (x/y=w26:dbl)
    n10 = expression code="1-x"(w26) -> (w13:dbl)
    n11 = In Range and Coerce(upper limit=1.0, x=w13, lower limit=0.0) -> (coerced(x)=w10:dbl)  [unwired: 1 out]
    n12 = Multiply(x="Total time", y=w10) -> (x*y=w22:dbl)
    n13 = Bundle("AO SampClk.MaxRate"="AO SampClk.MaxRate", "AI SampClk.MaxRate"="AI SampClk.MaxRate", "AO rate"="AO rate", "Scan speed"="Scan speed", "Detector number"="Detector number", "X min (V)"="X min (V)", "X max (V)"="X max (V)", "X min index"="X min index", "X max index"="X max index", "AO multiline"="AO multiline", "Decimating factor"="Decimating factor", "AvailSampPerChan"="AvailSampPerChan", "AO scan line"="AO scan line", "Total pixels recorded"="Total pixels recorded", "Total lines scanned"="Total lines scanned", "Scan time (m)"="Scan time (m)", "Scan time (s)"="Scan time (s)", "Remaining time (m)"="Remaining time (m)", "Remaining time (s)"="Remaining time (s)", "SEM Spec. I (nA)"="SEM Spec. I (nA)", "Frame"="Frame", w7, w6) -> (w14:T13)  [unwired: 1 out]
    "Info & Status" <- w14
    n14 = Quotient & Remainder(x=w22, y=60.0) -> (x-y*floor(x/y)=w25:dbl, floor(x/y)=w24:dbl)
    n15 = To Variant(anything=w14) -> (Variant=w15:variant)
    n16 = Wait Until Next ms Multiple(millisecond multiple=u32 100) -> ()  [unwired: 1 out]
    n17 = To Unsigned Byte Integer(number=w25) -> (unsigned 8bit integer=w18:u8)
    n18 = To Unsigned Word Integer(number=w24) -> (unsigned 16bit integer=w19:u16)
    n19 = shared-variable ".\\Zeiss Library.lvlib\\SEMInfo"(w15) -> ()  [unwired: 2 out]
    n20 = local write "Remaining time (s)"(w18) -> ()
    n21 = local write "Remaining time (m)"(w19) -> ()
  }
  n22 = stacked-sequence {
    tunnel: w1 -> [_ _ _ _ _]
    frame #0 {
      w133 = i16[][] [] ("SEM")
      n23 = shared-variable ".\\Zeiss Library.lvlib\\SW date"() -> (→"SW date":string)  [unwired: 1 in, 1 out]
      n24 = local write "Det B Img"(w133) -> ()
      n25 = local write "Det A Img"(w133) -> ()
      n26 = local write "Det C Img"(w133) -> ()
      n27 = local write "Det D Img"(w133) -> ()
      n28 = Unbundle By Name("HW Config") -> ("Det min (V)"=→"Det min (V)":dbl, "Det max (V)"=→"Det max (V)":dbl, "Eanable COM"=→"Eanable COM":bool, "COM port"=→"COM port":refnum<visa-resource-name>, "Detector FIB-NI auto switch"=→"Detector FIB-NI auto switch":tag, "Machine ID"=w60:string)
      "Machine ID" <- w60
      n29 = Unbundle By Name("Scan Para") -> ("X resolution"=w48:u32, "Y resolution"=→"Y resolution":u32, "X size (V)"=w51:dbl, "Scan rate (Hz)"=→"Scan rate (Hz)":u32, "Oversampling"=→"Oversampling":u32, "Frame line rampdown ratio"=→"Frame line rampdown ratio":sgl, "Pixel size (nm)"=w71:sgl, "WD"=→"WD":sgl, "X stig"=→"X stig":sgl, "Y stig"=→"Y stig":sgl, "X aln"=→"X aln":sgl, "Y aln"=→"Y aln":sgl)  [unwired: 3 out]
      "X resolution" <- w48
      "Pixel size (nm)" <- w71
      n30 = Unbundle By Name("Options") -> ("GetInfo"=→"GetInfo":bool, "Set Det A para"=→"Set Det A para":bool, "Set WD"=→"Set WD":bool, "Set Mag"=→"Set Mag":bool, "Set stig"=→"Set stig":bool, "Set aln"=→"Set aln":bool, "Display"=→"Display":bool, "Save"=→"Save":bool, "8-bit"=→"8-bit":bool, "Detector A"=→"Detector A":bool, "Detector B"=→"Detector B":bool, "Detector C"=→"Detector C":bool, "Detector D"=→"Detector D":bool, "Inverse A"=→"Inverse A":bool, "Inverse B"=→"Inverse B":bool, "Inverse C"=→"Inverse C":bool, "Inverse D"=→"Inverse D":bool, "Inverse PNG"=→"Inverse PNG":bool, "Freeze"=→"Freeze":bool, "PNG only"=→"PNG only":bool, "Upload"=→"Upload":bool, "Delete after upload"=→"Delete after upload":bool)
      n31 = Unbundle By Name("Focus Index Options") -> ("Keep aspect ratio"=→"keep aspect ratio":bool, "X Grids"=→"X Grids":u8, "Y Grids"=→"Y Grids":u8, "Primary X index"=→"Primary X index":u8, "Primary Y index"=→"Primary Y index":u8)
      n32 = Unbundle By Name("File Info") -> ("File path"=→"File path":path, "Notes"=→"Notes":string, "Sample ID"=→"Sample ID":string)
      n33 = local read "Inverse A"() -> (w143:bool)
      n34 = case shown="False" w143 {
        tunnel: [u32[] [16777222, 65793, 131586, 197379, 263172, 328965, 394758, 460551, 526344, 592137, 657930, 723723, 789516, 855309, 921102, 986895, 1052688, 1118481, 1184274, 1250067, 1315860, 1381653, 1447446, 1513239, 1579032, 1644825, 1710618, 1776411, 1842204, 1907997, 1973790, 2039583, 2105376, 2171169, 2236962, 2302755, 2368548, 2434341, 2500134, 2565927, 2631720, 2697513, 2763306, 2829099, 2894892, 2960685, 3026478, 3092271, 3158064, 3223857, 3289650, 3355443, 3421236, 3487029, 3552822, 3618615, 3684408, 3750201, 3815994, 3881787, 3947580, 4013373, 4079166, 4144959, 4210752, 4276545, 4342338, 4408131, 4473924, 4539717, 4605510, 4671303, 4737096, 4802889, 4868682, 4934475, 5000268, 5066061, 5131854, 5197647, 5263440, 5329233, 5395026, 5460819, 5526612, 5592405, 5658198, 5723991, 5789784, 5855577, 5921370, 5987163, 6052956, 6118749, 6184542, 6250335, 6316128, 6381921, 6447714, 6513507, 6579300, 6645093, 6710886, 6776679, 6842472, 6908265, 6974058, 7039851, 7105644, 7171437, 7237230, 7303023, 7368816, 7434609, 7500402, 7566195, 7631988, 7697781, 7763574, 7829367, 7895160, 7960953, 8026746, 8092539, 8158332, 8224125, 8289918, 8355711, 8421504, 8487297, 8553090, 8618883, 8684676, 8750469, 8816262, 8882055, 8947848, 9013641, 9079434, 9145227, 9211020, 9276813, 9342606, 9408399, 9474192, 9539985, 9605778, 9671571, 9737364, 9803157, 9868950, 9934743, 10000536, 10066329, 10132122, 10197915, 10263708, 10329501, 10395294, 10461087, 10526880, 10592673, 10658466, 10724259, 10790052, 10855845, 10921638, 10987431, 11053224, 11119017, 11184810, 11250603, 11316396, 11382189, 11447982, 11513775, 11579568, 11645361, 11711154, 11776947, 11842740, 11908533, 11974326, 12040119, 12105912, 12171705, 12237498, 12303291, 12369084, 12434877, 12500670, 12566463, 12632256, 12698049, 12763842, 12829635, 12895428, 12961221, 13027014, 13092807, 13158600, 13224393, 13290186, 13355979, 13421772, 13487565, 13553358, 13619151, 13684944, 13750737, 13816530, 13882323, 13948116, 14013909, 14079702, 14145495, 14211288, 14277081, 14342874, 14408667, 14474460, 14540253, 14606046, 14671839, 14737632, 14803425, 14869218, 14935011, 15000804, 15066597, 15132390, 15198183, 15263976, 15329769, 15395562, 15461355, 15527148, 15592941, 15658734, 15724527, 15790320, 15856113, 15921906, 15987699, 16053492, 16119285, 16185078, 16250871, 16316664, 16382457, 16448250, 16514043, 16579836, 16645629, 16711422, 16448250] ("256 gray scale") u32[] [16448250, 16711422, 16645629, 16579836, 16514043, 16448250, 16382457, 16316664, 16250871, 16185078, 16119285, 16053492, 15987699, 15921906, 15856113, 15790320, 15724527, 15658734, 15592941, 15527148, 15461355, 15395562, 15329769, 15263976, 15198183, 15132390, 15066597, 15000804, 14935011, 14869218, 14803425, 14737632, 14671839, 14606046, 14540253, 14474460, 14408667, 14342874, 14277081, 14211288, 14145495, 14079702, 14013909, 13948116, 13882323, 13816530, 13750737, 13684944, 13619151, 13553358, 13487565, 13421772, 13355979, 13290186, 13224393, 13158600, 13092807, 13027014, 12961221, 12895428, 12829635, 12763842, 12698049, 12632256, 12566463, 12500670, 12434877, 12369084, 12303291, 12237498, 12171705, 12105912, 12040119, 11974326, 11908533, 11842740, 11776947, 11711154, 11645361, 11579568, 11513775, 11447982, 11382189, 11316396, 11250603, 11184810, 11119017, 11053224, 10987431, 10921638, 10855845, 10790052, 10724259, 10658466, 10592673, 10526880, 10461087, 10395294, 10329501, 10263708, 10197915, 10132122, 10066329, 10000536, 9934743, 9868950, 9803157, 9737364, 9671571, 9605778, 9539985, 9474192, 9408399, 9342606, 9276813, 9211020, 9145227, 9079434, 9013641, 8947848, 8882055, 8816262, 8750469, 8684676, 8618883, 8553090, 8487297, 8421504, 8355711, 8289918, 8224125, 8158332, 8092539, 8026746, 7960953, 7895160, 7829367, 7763574, 7697781, 7631988, 7566195, 7500402, 7434609, 7368816, 7303023, 7237230, 7171437, 7105644, 7039851, 6974058, 6908265, 6842472, 6776679, 6710886, 6645093, 6579300, 6513507, 6447714, 6381921, 6316128, 6250335, 6184542, 6118749, 6052956, 5987163, 5921370, 5855577, 5789784, 5723991, 5658198, 5592405, 5526612, 5460819, 5395026, 5329233, 5263440, 5197647, 5131854, 5066061, 5000268, 4934475, 4868682, 4802889, 4737096, 4671303, 4605510, 4539717, 4473924, 4408131, 4342338, 4276545, 4210752, 4144959, 4079166, 4013373, 3947580, 3881787, 3815994, 3750201, 3684408, 3618615, 3552822, 3487029, 3421236, 3355443, 3289650, 3223857, 3158064, 3092271, 3026478, 2960685, 2894892, 2829099, 2763306, 2697513, 2631720, 2565927, 2500134, 2434341, 2368548, 2302755, 2236962, 2171169, 2105376, 2039583, 1973790, 1907997, 1842204, 1776411, 1710618, 1644825, 1579032, 1513239, 1447446, 1381653, 1315860, 1250067, 1184274, 1118481, 1052688, 986895, 921102, 855309, 789516, 723723, 657930, 592137, 526344, 460551, 394758, 328965, 263172, 197379, 131586, 65793, 16777222] ("256 gray scale inverse")] -> _
        frame False {
        }
        frame True {
        }
      }
      n35 = local read "Inverse B"() -> (w144:bool)
      n36 = case shown="False" w144 {
        tunnel: [u32[] [16777222, 65793, 131586, 197379, 263172, 328965, 394758, 460551, 526344, 592137, 657930, 723723, 789516, 855309, 921102, 986895, 1052688, 1118481, 1184274, 1250067, 1315860, 1381653, 1447446, 1513239, 1579032, 1644825, 1710618, 1776411, 1842204, 1907997, 1973790, 2039583, 2105376, 2171169, 2236962, 2302755, 2368548, 2434341, 2500134, 2565927, 2631720, 2697513, 2763306, 2829099, 2894892, 2960685, 3026478, 3092271, 3158064, 3223857, 3289650, 3355443, 3421236, 3487029, 3552822, 3618615, 3684408, 3750201, 3815994, 3881787, 3947580, 4013373, 4079166, 4144959, 4210752, 4276545, 4342338, 4408131, 4473924, 4539717, 4605510, 4671303, 4737096, 4802889, 4868682, 4934475, 5000268, 5066061, 5131854, 5197647, 5263440, 5329233, 5395026, 5460819, 5526612, 5592405, 5658198, 5723991, 5789784, 5855577, 5921370, 5987163, 6052956, 6118749, 6184542, 6250335, 6316128, 6381921, 6447714, 6513507, 6579300, 6645093, 6710886, 6776679, 6842472, 6908265, 6974058, 7039851, 7105644, 7171437, 7237230, 7303023, 7368816, 7434609, 7500402, 7566195, 7631988, 7697781, 7763574, 7829367, 7895160, 7960953, 8026746, 8092539, 8158332, 8224125, 8289918, 8355711, 8421504, 8487297, 8553090, 8618883, 8684676, 8750469, 8816262, 8882055, 8947848, 9013641, 9079434, 9145227, 9211020, 9276813, 9342606, 9408399, 9474192, 9539985, 9605778, 9671571, 9737364, 9803157, 9868950, 9934743, 10000536, 10066329, 10132122, 10197915, 10263708, 10329501, 10395294, 10461087, 10526880, 10592673, 10658466, 10724259, 10790052, 10855845, 10921638, 10987431, 11053224, 11119017, 11184810, 11250603, 11316396, 11382189, 11447982, 11513775, 11579568, 11645361, 11711154, 11776947, 11842740, 11908533, 11974326, 12040119, 12105912, 12171705, 12237498, 12303291, 12369084, 12434877, 12500670, 12566463, 12632256, 12698049, 12763842, 12829635, 12895428, 12961221, 13027014, 13092807, 13158600, 13224393, 13290186, 13355979, 13421772, 13487565, 13553358, 13619151, 13684944, 13750737, 13816530, 13882323, 13948116, 14013909, 14079702, 14145495, 14211288, 14277081, 14342874, 14408667, 14474460, 14540253, 14606046, 14671839, 14737632, 14803425, 14869218, 14935011, 15000804, 15066597, 15132390, 15198183, 15263976, 15329769, 15395562, 15461355, 15527148, 15592941, 15658734, 15724527, 15790320, 15856113, 15921906, 15987699, 16053492, 16119285, 16185078, 16250871, 16316664, 16382457, 16448250, 16514043, 16579836, 16645629, 16711422, 16448250] ("256 gray scale") u32[] [16448250, 16711422, 16645629, 16579836, 16514043, 16448250, 16382457, 16316664, 16250871, 16185078, 16119285, 16053492, 15987699, 15921906, 15856113, 15790320, 15724527, 15658734, 15592941, 15527148, 15461355, 15395562, 15329769, 15263976, 15198183, 15132390, 15066597, 15000804, 14935011, 14869218, 14803425, 14737632, 14671839, 14606046, 14540253, 14474460, 14408667, 14342874, 14277081, 14211288, 14145495, 14079702, 14013909, 13948116, 13882323, 13816530, 13750737, 13684944, 13619151, 13553358, 13487565, 13421772, 13355979, 13290186, 13224393, 13158600, 13092807, 13027014, 12961221, 12895428, 12829635, 12763842, 12698049, 12632256, 12566463, 12500670, 12434877, 12369084, 12303291, 12237498, 12171705, 12105912, 12040119, 11974326, 11908533, 11842740, 11776947, 11711154, 11645361, 11579568, 11513775, 11447982, 11382189, 11316396, 11250603, 11184810, 11119017, 11053224, 10987431, 10921638, 10855845, 10790052, 10724259, 10658466, 10592673, 10526880, 10461087, 10395294, 10329501, 10263708, 10197915, 10132122, 10066329, 10000536, 9934743, 9868950, 9803157, 9737364, 9671571, 9605778, 9539985, 9474192, 9408399, 9342606, 9276813, 9211020, 9145227, 9079434, 9013641, 8947848, 8882055, 8816262, 8750469, 8684676, 8618883, 8553090, 8487297, 8421504, 8355711, 8289918, 8224125, 8158332, 8092539, 8026746, 7960953, 7895160, 7829367, 7763574, 7697781, 7631988, 7566195, 7500402, 7434609, 7368816, 7303023, 7237230, 7171437, 7105644, 7039851, 6974058, 6908265, 6842472, 6776679, 6710886, 6645093, 6579300, 6513507, 6447714, 6381921, 6316128, 6250335, 6184542, 6118749, 6052956, 5987163, 5921370, 5855577, 5789784, 5723991, 5658198, 5592405, 5526612, 5460819, 5395026, 5329233, 5263440, 5197647, 5131854, 5066061, 5000268, 4934475, 4868682, 4802889, 4737096, 4671303, 4605510, 4539717, 4473924, 4408131, 4342338, 4276545, 4210752, 4144959, 4079166, 4013373, 3947580, 3881787, 3815994, 3750201, 3684408, 3618615, 3552822, 3487029, 3421236, 3355443, 3289650, 3223857, 3158064, 3092271, 3026478, 2960685, 2894892, 2829099, 2763306, 2697513, 2631720, 2565927, 2500134, 2434341, 2368548, 2302755, 2236962, 2171169, 2105376, 2039583, 1973790, 1907997, 1842204, 1776411, 1710618, 1644825, 1579032, 1513239, 1447446, 1381653, 1315860, 1250067, 1184274, 1118481, 1052688, 986895, 921102, 855309, 789516, 723723, 657930, 592137, 526344, 460551, 394758, 328965, 263172, 197379, 131586, 65793, 16777222] ("256 gray scale inverse")] -> _
        frame False {
        }
        frame True {
        }
      }
      n37 = xnode "Match Regular Expression"("input string"=w60, "regular expression"="Merlin", "ignore case? (F)"=TRUE) -> ("offset past match"=w80:i32)  [unwired: 3 in, 4 out]
      n38 = xnode "Match Regular Expression"("input string"=w60, "regular expression"="Gemini500", "ignore case? (F)"=TRUE) -> ("offset past match"=w66:i32)  [unwired: 3 in, 4 out]
      n39 = local read "Inverse C"() -> (w145:bool)
      n40 = Equal?(x=w80, y=-1) -> (x = y?=w61:bool)
      n41 = Equal?(x=w66, y=-1) -> (x = y?=w63:bool)
      n42 = And(x=w61, y=w63) -> (x .and. y?=w62:bool)
      n43 = Divide(x=w51, y=20.0) -> (x/y=w74:dbl)
      n44 = case shown="False" w145 {
        tunnel: [u32[] [16777222, 65793, 131586, 197379, 263172, 328965, 394758, 460551, 526344, 592137, 657930, 723723, 789516, 855309, 921102, 986895, 1052688, 1118481, 1184274, 1250067, 1315860, 1381653, 1447446, 1513239, 1579032, 1644825, 1710618, 1776411, 1842204, 1907997, 1973790, 2039583, 2105376, 2171169, 2236962, 2302755, 2368548, 2434341, 2500134, 2565927, 2631720, 2697513, 2763306, 2829099, 2894892, 2960685, 3026478, 3092271, 3158064, 3223857, 3289650, 3355443, 3421236, 3487029, 3552822, 3618615, 3684408, 3750201, 3815994, 3881787, 3947580, 4013373, 4079166, 4144959, 4210752, 4276545, 4342338, 4408131, 4473924, 4539717, 4605510, 4671303, 4737096, 4802889, 4868682, 4934475, 5000268, 5066061, 5131854, 5197647, 5263440, 5329233, 5395026, 5460819, 5526612, 5592405, 5658198, 5723991, 5789784, 5855577, 5921370, 5987163, 6052956, 6118749, 6184542, 6250335, 6316128, 6381921, 6447714, 6513507, 6579300, 6645093, 6710886, 6776679, 6842472, 6908265, 6974058, 7039851, 7105644, 7171437, 7237230, 7303023, 7368816, 7434609, 7500402, 7566195, 7631988, 7697781, 7763574, 7829367, 7895160, 7960953, 8026746, 8092539, 8158332, 8224125, 8289918, 8355711, 8421504, 8487297, 8553090, 8618883, 8684676, 8750469, 8816262, 8882055, 8947848, 9013641, 9079434, 9145227, 9211020, 9276813, 9342606, 9408399, 9474192, 9539985, 9605778, 9671571, 9737364, 9803157, 9868950, 9934743, 10000536, 10066329, 10132122, 10197915, 10263708, 10329501, 10395294, 10461087, 10526880, 10592673, 10658466, 10724259, 10790052, 10855845, 10921638, 10987431, 11053224, 11119017, 11184810, 11250603, 11316396, 11382189, 11447982, 11513775, 11579568, 11645361, 11711154, 11776947, 11842740, 11908533, 11974326, 12040119, 12105912, 12171705, 12237498, 12303291, 12369084, 12434877, 12500670, 12566463, 12632256, 12698049, 12763842, 12829635, 12895428, 12961221, 13027014, 13092807, 13158600, 13224393, 13290186, 13355979, 13421772, 13487565, 13553358, 13619151, 13684944, 13750737, 13816530, 13882323, 13948116, 14013909, 14079702, 14145495, 14211288, 14277081, 14342874, 14408667, 14474460, 14540253, 14606046, 14671839, 14737632, 14803425, 14869218, 14935011, 15000804, 15066597, 15132390, 15198183, 15263976, 15329769, 15395562, 15461355, 15527148, 15592941, 15658734, 15724527, 15790320, 15856113, 15921906, 15987699, 16053492, 16119285, 16185078, 16250871, 16316664, 16382457, 16448250, 16514043, 16579836, 16645629, 16711422, 16448250] ("256 gray scale") u32[] [16448250, 16711422, 16645629, 16579836, 16514043, 16448250, 16382457, 16316664, 16250871, 16185078, 16119285, 16053492, 15987699, 15921906, 15856113, 15790320, 15724527, 15658734, 15592941, 15527148, 15461355, 15395562, 15329769, 15263976, 15198183, 15132390, 15066597, 15000804, 14935011, 14869218, 14803425, 14737632, 14671839, 14606046, 14540253, 14474460, 14408667, 14342874, 14277081, 14211288, 14145495, 14079702, 14013909, 13948116, 13882323, 13816530, 13750737, 13684944, 13619151, 13553358, 13487565, 13421772, 13355979, 13290186, 13224393, 13158600, 13092807, 13027014, 12961221, 12895428, 12829635, 12763842, 12698049, 12632256, 12566463, 12500670, 12434877, 12369084, 12303291, 12237498, 12171705, 12105912, 12040119, 11974326, 11908533, 11842740, 11776947, 11711154, 11645361, 11579568, 11513775, 11447982, 11382189, 11316396, 11250603, 11184810, 11119017, 11053224, 10987431, 10921638, 10855845, 10790052, 10724259, 10658466, 10592673, 10526880, 10461087, 10395294, 10329501, 10263708, 10197915, 10132122, 10066329, 10000536, 9934743, 9868950, 9803157, 9737364, 9671571, 9605778, 9539985, 9474192, 9408399, 9342606, 9276813, 9211020, 9145227, 9079434, 9013641, 8947848, 8882055, 8816262, 8750469, 8684676, 8618883, 8553090, 8487297, 8421504, 8355711, 8289918, 8224125, 8158332, 8092539, 8026746, 7960953, 7895160, 7829367, 7763574, 7697781, 7631988, 7566195, 7500402, 7434609, 7368816, 7303023, 7237230, 7171437, 7105644, 7039851, 6974058, 6908265, 6842472, 6776679, 6710886, 6645093, 6579300, 6513507, 6447714, 6381921, 6316128, 6250335, 6184542, 6118749, 6052956, 5987163, 5921370, 5855577, 5789784, 5723991, 5658198, 5592405, 5526612, 5460819, 5395026, 5329233, 5263440, 5197647, 5131854, 5066061, 5000268, 4934475, 4868682, 4802889, 4737096, 4671303, 4605510, 4539717, 4473924, 4408131, 4342338, 4276545, 4210752, 4144959, 4079166, 4013373, 3947580, 3881787, 3815994, 3750201, 3684408, 3618615, 3552822, 3487029, 3421236, 3355443, 3289650, 3223857, 3158064, 3092271, 3026478, 2960685, 2894892, 2829099, 2763306, 2697513, 2631720, 2565927, 2500134, 2434341, 2368548, 2302755, 2236962, 2171169, 2105376, 2039583, 1973790, 1907997, 1842204, 1776411, 1710618, 1644825, 1579032, 1513239, 1447446, 1381653, 1315860, 1250067, 1184274, 1118481, 1052688, 986895, 921102, 855309, 789516, 723723, 657930, 592137, 526344, 460551, 394758, 328965, 263172, 197379, 131586, 65793, 16777222] ("256 gray scale inverse")] -> _
        frame False {
        }
        frame True {
        }
      }
      n45 = case shown="False" w62 {
        tunnel: [u8 14 ("t") u8 16 ("t")] -> w78
        tunnel: [u8 25 ("t") u8 1 ("t")] -> w77
        frame False {
        }
        frame True {
        }
      }
      "Image bits" <- w78
      "FI scaling" <- w77
      n46 = expression code="x*1024"(w74) -> (w69:dbl)
      n47 = local read "Detector A"() -> (w137:bool)
      n48 = local read "Detector B"() -> (w136:bool)
      n49 = local read "Detector C"() -> (w138:bool)
      n50 = local read "Detector D"() -> (w139:bool)
      n51 = local read "Inverse D"() -> (w146:bool)
      n52 = Unbundle By Name("Det Info") -> ("Brightness A"=→"Brightness A":dbl, "Contrast A"=→"Contrast A":dbl, "Detector B name"=→"Detector B name":string, "Brightness B"=→"Brightness B":dbl, "Contrast B"=→"Contrast B":dbl, "Detector C name"=→"Detector C name":string, "Detector D name"=→"Detector D name":string)
      n53 = Divide(x=w69, y=w48) -> (x/y=w68:dbl)
      n54 = shared-variable ".\\Zeiss Library.lvlib\\X full scale (V)"() -> (w50:sgl)  [unwired: 1 in, 1 out]
      n55 = Boolean To (0,1)(Boolean=w137) -> (0, 1=w134:i16)
      n56 = Boolean To (0,1)(Boolean=w136) -> (0, 1=w135:i16)
      n57 = Boolean To (0,1)(Boolean=w138) -> (0, 1=w140:i16)
      n58 = Boolean To (0,1)(Boolean=w139) -> (0, 1=w141:i16)
      n59 = case shown="False" w146 {
        tunnel: [u32[] [16777222, 65793, 131586, 197379, 263172, 328965, 394758, 460551, 526344, 592137, 657930, 723723, 789516, 855309, 921102, 986895, 1052688, 1118481, 1184274, 1250067, 1315860, 1381653, 1447446, 1513239, 1579032, 1644825, 1710618, 1776411, 1842204, 1907997, 1973790, 2039583, 2105376, 2171169, 2236962, 2302755, 2368548, 2434341, 2500134, 2565927, 2631720, 2697513, 2763306, 2829099, 2894892, 2960685, 3026478, 3092271, 3158064, 3223857, 3289650, 3355443, 3421236, 3487029, 3552822, 3618615, 3684408, 3750201, 3815994, 3881787, 3947580, 4013373, 4079166, 4144959, 4210752, 4276545, 4342338, 4408131, 4473924, 4539717, 4605510, 4671303, 4737096, 4802889, 4868682, 4934475, 5000268, 5066061, 5131854, 5197647, 5263440, 5329233, 5395026, 5460819, 5526612, 5592405, 5658198, 5723991, 5789784, 5855577, 5921370, 5987163, 6052956, 6118749, 6184542, 6250335, 6316128, 6381921, 6447714, 6513507, 6579300, 6645093, 6710886, 6776679, 6842472, 6908265, 6974058, 7039851, 7105644, 7171437, 7237230, 7303023, 7368816, 7434609, 7500402, 7566195, 7631988, 7697781, 7763574, 7829367, 7895160, 7960953, 8026746, 8092539, 8158332, 8224125, 8289918, 8355711, 8421504, 8487297, 8553090, 8618883, 8684676, 8750469, 8816262, 8882055, 8947848, 9013641, 9079434, 9145227, 9211020, 9276813, 9342606, 9408399, 9474192, 9539985, 9605778, 9671571, 9737364, 9803157, 9868950, 9934743, 10000536, 10066329, 10132122, 10197915, 10263708, 10329501, 10395294, 10461087, 10526880, 10592673, 10658466, 10724259, 10790052, 10855845, 10921638, 10987431, 11053224, 11119017, 11184810, 11250603, 11316396, 11382189, 11447982, 11513775, 11579568, 11645361, 11711154, 11776947, 11842740, 11908533, 11974326, 12040119, 12105912, 12171705, 12237498, 12303291, 12369084, 12434877, 12500670, 12566463, 12632256, 12698049, 12763842, 12829635, 12895428, 12961221, 13027014, 13092807, 13158600, 13224393, 13290186, 13355979, 13421772, 13487565, 13553358, 13619151, 13684944, 13750737, 13816530, 13882323, 13948116, 14013909, 14079702, 14145495, 14211288, 14277081, 14342874, 14408667, 14474460, 14540253, 14606046, 14671839, 14737632, 14803425, 14869218, 14935011, 15000804, 15066597, 15132390, 15198183, 15263976, 15329769, 15395562, 15461355, 15527148, 15592941, 15658734, 15724527, 15790320, 15856113, 15921906, 15987699, 16053492, 16119285, 16185078, 16250871, 16316664, 16382457, 16448250, 16514043, 16579836, 16645629, 16711422, 16448250] ("256 gray scale") u32[] [16448250, 16711422, 16645629, 16579836, 16514043, 16448250, 16382457, 16316664, 16250871, 16185078, 16119285, 16053492, 15987699, 15921906, 15856113, 15790320, 15724527, 15658734, 15592941, 15527148, 15461355, 15395562, 15329769, 15263976, 15198183, 15132390, 15066597, 15000804, 14935011, 14869218, 14803425, 14737632, 14671839, 14606046, 14540253, 14474460, 14408667, 14342874, 14277081, 14211288, 14145495, 14079702, 14013909, 13948116, 13882323, 13816530, 13750737, 13684944, 13619151, 13553358, 13487565, 13421772, 13355979, 13290186, 13224393, 13158600, 13092807, 13027014, 12961221, 12895428, 12829635, 12763842, 12698049, 12632256, 12566463, 12500670, 12434877, 12369084, 12303291, 12237498, 12171705, 12105912, 12040119, 11974326, 11908533, 11842740, 11776947, 11711154, 11645361, 11579568, 11513775, 11447982, 11382189, 11316396, 11250603, 11184810, 11119017, 11053224, 10987431, 10921638, 10855845, 10790052, 10724259, 10658466, 10592673, 10526880, 10461087, 10395294, 10329501, 10263708, 10197915, 10132122, 10066329, 10000536, 9934743, 9868950, 9803157, 9737364, 9671571, 9605778, 9539985, 9474192, 9408399, 9342606, 9276813, 9211020, 9145227, 9079434, 9013641, 8947848, 8882055, 8816262, 8750469, 8684676, 8618883, 8553090, 8487297, 8421504, 8355711, 8289918, 8224125, 8158332, 8092539, 8026746, 7960953, 7895160, 7829367, 7763574, 7697781, 7631988, 7566195, 7500402, 7434609, 7368816, 7303023, 7237230, 7171437, 7105644, 7039851, 6974058, 6908265, 6842472, 6776679, 6710886, 6645093, 6579300, 6513507, 6447714, 6381921, 6316128, 6250335, 6184542, 6118749, 6052956, 5987163, 5921370, 5855577, 5789784, 5723991, 5658198, 5592405, 5526612, 5460819, 5395026, 5329233, 5263440, 5197647, 5131854, 5066061, 5000268, 4934475, 4868682, 4802889, 4737096, 4671303, 4605510, 4539717, 4473924, 4408131, 4342338, 4276545, 4210752, 4144959, 4079166, 4013373, 3947580, 3881787, 3815994, 3750201, 3684408, 3618615, 3552822, 3487029, 3421236, 3355443, 3289650, 3223857, 3158064, 3092271, 3026478, 2960685, 2894892, 2829099, 2763306, 2697513, 2631720, 2565927, 2500134, 2434341, 2368548, 2302755, 2236962, 2171169, 2105376, 2039583, 1973790, 1907997, 1842204, 1776411, 1710618, 1644825, 1579032, 1513239, 1447446, 1381653, 1315860, 1250067, 1184274, 1118481, 1052688, 986895, 921102, 855309, 789516, 723723, 657930, 592137, 526344, 460551, 394758, 328965, 263172, 197379, 131586, 65793, 16777222] ("256 gray scale inverse")] -> _
        frame False {
        }
        frame True {
        }
      }
      n60 = Compound Arithmetic op=ADD(w134, w135, w140, w141) -> (w142:i16)
      n61 = local write "Detector number"(w142) -> ()
      n62 = Divide(x=w51, y=w50) -> (x/y=w52:dbl)
      n63 = expression code="x*1024"(w52) -> (w49:dbl)
      n64 = Divide(x=w49, y=w48) -> (x/y=→"Screen pixel factor":dbl)
      n65 = Divide(x=111652.0, y=w71) -> (x/y=w72:dbl)
      n66 = Multiply(x=w68, y=w72) -> (x*y=→"Mag":dbl)
    }
    frame #1 {
      w407 = T17 3 items=["no dialog", "OK message", "continue or stop message", "OK message + warnings", "continue/stop + warnings"] ("type of dialog (OK msg:1)")
      w411 = 0 items=["one channel for each line", "one channel for all lines"] ("line grouping")
      n67 = shared-variable "My Computer\\Zeiss Library.lvlib\\Machine Type"() -> (w381:u8)  [unwired: 1 in, 1 out]
      n68 = local read "8-bit"() -> (w384:bool)
      n69 = local read "Image bits"() -> (w385:u8)
      n70 = Select(t=u8 8, s=w384, f=w385) -> (s? t:f=w382:u8)
      n71 = local write "Image bits"(w382) -> ()
      n72 = case shown="2" w381 {
        tunnel: [w415 w683] -> w399
        frame 0, Default {
          n73 = local read "Eanable COM"() -> (w416:bool)
          n74 = case shown="True" w416 {
            tunnel: [w417 w448] -> w415
            frame False {
              n75 = local read "Detector B name"() -> (w430:string)
              n76 = local read "Brightness A"() -> (w428:dbl)
              n77 = local read "Contrast A"() -> (w427:dbl)
              n78 = local read "Brightness B"() -> (w426:dbl)
              n79 = local read "Contrast B"() -> (w425:dbl)
              n80 = local read "Mag"() -> (w422:dbl)
              n81 = local read "Pixel size (nm)"() -> (w424:sgl)
              n82 = local read "WD"() -> (w423:sgl)
              n83 = local read "X stig"() -> (w421:sgl)
              n84 = local read "Y stig"() -> (w420:sgl)
              n85 = local read "X aln"() -> (w419:sgl)
              n86 = local read "Y aln"() -> (w418:sgl)
              n87 = local read "SEM parameters"() -> (w431:T5)
              n88 = Bundle By Name(cluster=w431, "Detector A"="Det A", "Detector B"=w430, "Brightness A"=w428, "Contrast A"=w427, "Brightness B"=w426, "Contrast B"=w425, "Magnification"=w422, "Pixel size"=w424, "Working distance"=w423, "Stig X"=w421, "Stig Y"=w420, "Alignment X"=w419, "Alignment Y"=w418) -> (w417:T5)
              n89 = local write "SEM parameters"(w417) -> ()
            }
            frame True {
              n90 = local read "COM port"() -> (w475:refnum<visa-resource-name>)
              n91 = local read "HW Config"() -> (w441:T12)
              n92 = call "Remcon32 command.vi"("Initialization"=TRUE, "SEM command"="frez" ("write buffer"), "COM port in"=w475) -> ("error out"=w455:errorcluster, "COM port out"=w456:refnum<visa-resource-name>)  [unwired: 2 in, 5 out]
              n93 = Unbundle By Name(w441) -> ("Machine ID"=w437:string)
              n94 = local read "Set WD"() -> (w465:bool)
              n95 = call "Remcon32 command.vi"("error in"=w455, "SEM command"="edx 1" ("write buffer"), "COM port in"=w456) -> ("error out"=w443:errorcluster, "COM port out"=w445:refnum<visa-resource-name>)  [unwired: 2 in, 5 out]
              n96 = xnode "Match Regular Expression"("input string"=w437, "regular expression"="Merlin", "ignore case? (F)"=TRUE) -> ("offset past match"=w439:i32)  [unwired: 3 in, 4 out]
              n97 = Equal?(x=w439, y=-1) -> (x = y?=w435:bool)
              n98 = Select(t=u8 1, s=w435, f=u8 7 ("t")) -> (s? t:f=w432:u8)
              n99 = Format Into String(format string="rate %d", w432) -> (resulting string=w447:string)  [unwired: 2 in, 1 out]
              n100 = call "Remcon32 command.vi"("error in"=w443, "SEM command"=w447, "COM port in"=w445) -> ("error out"=w442:errorcluster, "COM port out"=w444:refnum<visa-resource-name>)  [unwired: 2 in, 5 out]
              n101 = local read "Set Mag"() -> (w464:bool)
              n102 = local read "Set Det A para"() -> (w466:bool)
              n103 = call "FIB mode.vi"("error in"=w442, "Iterations"=u32 1, "FIB mode"=T14."SEM", "COM port in"=w444) -> ("error out"=w467:errorcluster, "COM port out"=w468:refnum<visa-resource-name>)  [unwired: 2 in, 4 out]
              n104 = case shown="True" w466 {
                tunnel: w468 -> [w638 w642]
                tunnel: w467 -> [w637 w641]
                tunnel: [w638 w650] -> w462
                tunnel: [w637 w649] -> w461
                frame False {
                }
                frame True {
                  n105 = local read "Brightness A"() -> (w639:dbl)
                  n106 = Format Into String(format string="brgt %g", w639) -> (resulting string=w645:string)  [unwired: 2 in, 1 out]
                  n107 = call "Remcon32 command.vi"("error in"=w641, "SEM command"=w645, "COM port in"=w642) -> ("error out"=w643:errorcluster, "COM port out"=w644:refnum<visa-resource-name>)  [unwired: 2 in, 5 out]
                  n108 = local read "Contrast A"() -> (w640:dbl)
                  n109 = Format Into String(format string="crst %g", w640) -> (resulting string=w647:string)  [unwired: 2 in, 1 out]
                  n110 = call "Remcon32 command.vi"("error in"=w643, "SEM command"=w647, "COM port in"=w644) -> ("error out"=w649:errorcluster, "COM port out"=w650:refnum<visa-resource-name>)  [unwired: 2 in, 5 out]
                }
              }
              n111 = local read "HW Config"() -> (w459:T12)
              n112 = Unbundle By Name(w459) -> ("Machine Type"=w458:u8)
              n113 = local read "GetInfo"() -> (w460:bool)
              n114 = case shown="0, Default" w458 {
                tunnel: [FALSE ("Initialization") TRUE ("Initialization")] -> w457
                frame 0, Default {
                }
                frame 1 {
                }
              }
              n115 = local read "Set stig"() -> (w463:bool)
              n116 = case shown="True" w463 {
                tunnel: [w628 w636] -> w451
                tunnel: [w627 w635] -> w452
                tunnel: w462 -> [w628 w634]
                tunnel: w461 -> [w627 w633]
                frame False {
                }
                frame True {
                  n117 = local read "X stig"() -> (w630:sgl)
                  n118 = local read "Y stig"() -> (w632:sgl)
                  n119 = Format Into String(format string="stim %g %g", w630, w632) -> (resulting string=w629:string)  [unwired: 2 in, 1 out]
                  n120 = call "Remcon32 command.vi"("error in"=w633, "SEM command"=w629, "COM port in"=w634) -> ("error out"=w635:errorcluster, "COM port out"=w636:refnum<visa-resource-name>)  [unwired: 2 in, 5 out]
                }
              }
              n121 = local read "Set aln"() -> (w453:bool)
              n122 = case shown="True" w453 {
                tunnel: [w594 w602] -> w450
                tunnel: [w593 w601] -> w449
                tunnel: w451 -> [w594 w600]
                tunnel: w452 -> [w593 w599]
                frame False {
                }
                frame True {
                  n123 = local read "X aln"() -> (w596:sgl)
                  n124 = local read "Y aln"() -> (w598:sgl)
                  n125 = Format Into String(format string="aaln %g %g", w596, w598) -> (resulting string=w595:string)  [unwired: 2 in, 1 out]
                  n126 = call "Remcon32 command.vi"("error in"=w599, "SEM command"=w595, "COM port in"=w600) -> ("error out"=w601:errorcluster, "COM port out"=w602:refnum<visa-resource-name>)  [unwired: 2 in, 5 out]
                }
              }
              n127 = case shown="True" w465 {
                tunnel: w450 -> [w661 w671]
                tunnel: w449 -> [w660 w670]
                tunnel: [w661 w668] -> w472
                tunnel: [w660 w666] -> w470
                frame False {
                }
                frame True {
                  n128 = local read "WD"() -> (w664:sgl)
                  n129 = call "Remcon32 command.vi"("error in"=w670, "SEM command"="fblk 1", "COM port in"=w671) -> ("error out"=w667:errorcluster, "COM port out"=w669:refnum<visa-resource-name>)  [unwired: 2 in, 5 out]
                  n130 = Format Into String(format string="focs %g", w664) -> (resulting string=w662:string)  [unwired: 2 in, 1 out]
                  n131 = call "Remcon32 command.vi"("error in"=w667, "SEM command"=w662, "COM port in"=w669) -> ("error out"=w666:errorcluster, "COM port out"=w668:refnum<visa-resource-name>)  [unwired: 2 in, 5 out]
                }
              }
              n132 = case shown="True" w464 {
                tunnel: w472 -> [w652 w655]
                tunnel: [w652 w657] -> w471
                tunnel: w470 -> [w651 w654]
                tunnel: [w651 w656] -> w469
                frame False {
                }
                frame True {
                  n133 = local read "Mag"() -> (w653:dbl)
                  n134 = Format Into String(format string="mag %g", w653) -> (resulting string=w658:string)  [unwired: 2 in, 1 out]
                  n135 = call "Remcon32 command.vi"("error in"=w654, "SEM command"=w658, "COM port in"=w655) -> ("error out"=w656:errorcluster, "COM port out"=w657:refnum<visa-resource-name>)  [unwired: 2 in, 5 out]
                }
              }
              n136 = case shown="True" w460 {
                tunnel: [w611 w626] -> w477
                tunnel: [w610 w625] -> w476
                tunnel: w471 -> [w611 w624]
                tunnel: w469 -> [w610 w623]
                tunnel: w457 -> [_ w615]
                tunnel: [w605 w612] -> w448
                frame False {
                  n137 = local read "Mag"() -> (w606:dbl)
                  n138 = local read "Pixel size (nm)"() -> (w607:sgl)
                  n139 = local read "SEM parameters"() -> (w609:T5)
                  n140 = Bundle By Name(cluster=w609, "Magnification"=w606, "Pixel size"=w607) -> (w605:T5)
                  n141 = Wait (ms)(milliseconds to wait=u32 100) -> ()  [unwired: 1 out]
                }
                frame True {
                  w616 = FALSE ("Initialization")
                  n142 = call "Read Zeiss Parameters.vi"("Close session"=w616, "Initialization"=w616, "error in (no error)"=w623, "FIB"=w615, "COM port in"=w624) -> ("error out"=w625:errorcluster, "FIB parameters"=→"FIB parameters":T18, "SEM parameters"=w618:T5, "COM port out"=w626:refnum<visa-resource-name>)  [unwired: 3 out]
                  n143 = local read "Detector B name"() -> (w620:string)
                  n144 = local read "Brightness B"() -> (w621:dbl)
                  n145 = local read "Screen pixel factor"() -> (w614:dbl)
                  n146 = local read "Contrast B"() -> (w622:dbl)
                  n147 = Unbundle By Name(w618) -> ("Pixel size"=w617:sgl)
                  n148 = Multiply(x=w614, y=w617) -> (x*y=w613:dbl)
                  n149 = Bundle By Name(cluster=w618, "Detector B"=w620, "Brightness B"=w621, "Contrast B"=w622, "Pixel size"=w613) -> (w612:T5)
                }
              }
              "SEM parameters" <- w448
              n150 = call "Remcon32 command.vi"("Close session"=TRUE, "error in"=w476, "SEM command"="edx 1" ("write buffer"), "COM port in"=w477) -> ()  [unwired: 1 in, 7 out]
            }
          }
        }
        frame 2 {
          n151 = local read "Options"() -> (w694:T9)
          n152 = local read "Scan Para"() -> (w695:T10)
          n153 = local read "Det Info"() -> (w693:T11)
          n154 = call "SmartSEM Remote API set SEM parameters.vi"("Det Info"=w693, "Scan Para"=w695, "SEM Options"=w694, "Api in"="Api") -> ("error out"=w674:errorcluster, "Api out"=w675:refnum<k7>)  [unwired: 6 in]
          n155 = call "SmartSEM Remote API set string.vi"("error in"=w674, "vValue"="On", "lpszParam"="DP_EXT_SCAN_CONTROL" ("lpszCommand"), "Api"=w675) -> ("error out"=w672:errorcluster, "Api out"=w673:refnum<k7>)  [unwired: 6 in]
          n156 = call "SmartSEM Remote API get Zeiss parameters.vi"("error in"=w672, "Api in"=w673) -> ("error out"=w685:errorcluster, "FIB parameters"=w692:T6, "SEM parameters"=w687:T5, "Api out"=w684:refnum<k7>)  [unwired: 6 in]
          n157 = local read "Detector B name"() -> (w691:string)
          n158 = local read "Screen pixel factor"() -> (w689:dbl)
          n159 = Unbundle By Name(w687) -> ("Pixel size"=w690:sgl)
          n160 = local write "FIB parameters"(w692) -> ()
          n161 = Multiply(x=w689, y=w690) -> (x*y=w688:dbl)
          n162 = Bundle By Name(cluster=w687, "Detector B"=w691, "Pixel size"=w688) -> (w683:T5)
          n163 = local write "SEM parameters"(w683) -> ()
          n164 = invoke class="_EMApi" method="Execute"(reference=w684, error in=w685, "lpszCommand"="CMD_UNFREEZE_ALL") -> (reference out=w682:refnum<k7>, error out=w680:errorcluster)  [unwired: 1 in, 2 out]
          n165 = call "SmartSEM Remote API set string.vi"("Wait (ms)"=u32 10 ("wait (ms)"), "error in"=w680, "vValue"="On", "lpszParam"="DP_EXT_SCAN_CONTROL" ("lpszCommand"), "Api"=w682) -> ()  [unwired: 5 in, 2 out]
        }
      }
      n166 = local read "Detector FIB-NI auto switch"() -> (w403:tag)
      n167 = local write "Total lines scanned"(0 ("Read line")) -> ()
      n168 = call-poly <vilib>:"DAQmx Create Virtual Channel.vi"("lines"=w403, "line grouping"=w411) -> ("task out"=w413:refnum<k21>, "error out"=w412:errorcluster)  [unwired: 3 in, 9 out]
      n169 = call <vilib>:"DAQmx Start Task.vi"("task/channels in"=w413, "error in"=w412) -> ("task out"=w410:refnum<k21>, "error out"=w409:errorcluster)  [unwired: 12 out]
      n170 = call-poly <vilib>:"DAQmx Write.vi"("task/channels in"=w410, "data"=TRUE, "error in"=w409) -> ("task out"=w405:refnum<k21>, "error out"=w404:errorcluster)  [unwired: 1 in, 10 out]
      n171 = call <vilib>:"DAQmx Clear Task.vi"("task in"=w405, "error in"=w404) -> ("error out"=w406:errorcluster)  [unwired: 13 out]
      n172 = call <vilib>:"Simple Error Handler.vi"("type of dialog (OK msg:1)"=w407, "error in (no error)"=w406) -> ()  [unwired: 8 out]
      n173 = Unbundle By Name(w399) -> ("Brightness A"=w398:sgl, "Contrast A"=w396:sgl, "Brightness B"=w397:sgl, "Contrast B"=w395:sgl)
      n174 = call "Read detector calibrations.vi"("Contrast B"=w395, "Brightness B"=w397, "Contrast A"=w396, "Brightness A"=w398, "Path"=path "D:/3D FIB-SEM Files/Detector calibrations.csv" ("file path (dialog if empty)")) -> ("Latest 8-bit coefficients"=w386:sgl[][])  [unwired: 6 in]
      "8-bit coefficents" <- w386
      n175 = for {
        tunnel: w386 -> [w697] mode=indexing
        tunnel: [w697] -> w402 mode=concatenating
      }
      n176 = Array To Cluster(array=w402) -> (cluster=w401:T19)
      n177 = Unbundle(w401) -> ("Latest 8-bit coefficients[0]"=→"DetA-Rate":sgl, "Latest 8-bit coefficients[1]"=→"DetA-Io":sgl, "Latest 8-bit coefficients[2]"=→"DetA-k":sgl, "Latest 8-bit coefficients[3]"=→"DetA-Scaling":sgl, "Latest 8-bit coefficients[4]"=→"DetB-Rate":sgl, "Latest 8-bit coefficients[5]"=→"DetB-Io":sgl, "Latest 8-bit coefficients[6]"=→"DetB-k":sgl, "Latest 8-bit coefficients[7]"=→"DetB-Scaling":sgl)
    }
    frame #2 {
      w698 = 3 ("index")
      w701 = 1 ("index")
      w802 = 1 ("dimension size")
      n178 = local read "Save"() -> (w806:bool)
      n179 = local read "HW Config"() -> (w718:T12)
      n180 = local read "Scan Para"() -> (w717:T10)
      n181 = local read "Options"() -> (w716:T9)
      n182 = shared-variable ".\\Zeiss Library.lvlib\\Tclk para"() -> (w720:variant)  [unwired: 1 in, 1 out]
      n183 = local read "Detector C"() -> (w787:bool)
      n184 = local read "Detector A"() -> (w804:bool)
      n185 = local read "Display"() -> (w805:bool)
      n186 = local read "Detector B"() -> (w794:bool)
      n187 = local read "Display"() -> (w793:bool)
      n188 = local read "Display"() -> (w788:bool)
      n189 = local read "Detector D"() -> (w785:bool)
      n190 = local read "Display"() -> (w784:bool)
      n191 = Not(x="Force tclk init") -> (.not. x?=w710:bool)
      n192 = And(x=w804, y=w805) -> (x .and. y?=w798:bool)
      n193 = And(x=w794, y=w793) -> (x .and. y?=w792:bool)
      n194 = And(x=w787, y=w788) -> (x .and. y?=w786:bool)
      n195 = And(x=w785, y=w784) -> (x .and. y?=w783:bool)
      n196 = call "Tclk parameters.vi"("variant"=w720, "Options"=w716, "Scan Para"=w717, "HW Config"=w718) -> ("Same tclk para?"=w711:bool)  [unwired: 6 in, 1 out]
      n197 = call "Tclk FGV.vi"("Action"=T15."Get Reference", "Options"=w716, "Scan Para"=w717, "HW Config"=w718) -> ("Tclk handle valid"=w712:bool, "Initialized handles"=w715:T20)  [unwired: 6 in]
      n198 = Initialize Array(i16 0 ("element"), w802, w802) -> (w777:i16[][])
      n199 = Compound Arithmetic op=AND(w711, w712, w710) -> (w714:bool)
      n200 = case shown="False" w714 {
        tunnel: w718 -> [w840 _]
        tunnel: w717 -> [w839 _]
        tunnel: w716 -> [w838 _]
        tunnel: [w837 w850] -> w730
        tunnel: w715 -> [_ w850]
        frame False {
          n201 = stacked-sequence {
            tunnel: w840 -> [w844 w849]
            tunnel: w839 -> [w843 w848]
            tunnel: w838 -> [w842 w847]
            tunnel: [_ w845] -> w837
            frame #0 {
              n202 = call "Tclk FGV.vi"("Action"=T15."Close Reference", "Options"=w842, "Scan Para"=w843, "HW Config"=w844) -> ()  [unwired: 6 in, 2 out]
            }
            frame #1 {
              n203 = call "Tclk FGV.vi"("Action"=T15."Initialize Reference", "Options"=w847, "Scan Para"=w848, "HW Config"=w849) -> ("Initialized handles"=w845:T20)  [unwired: 6 in, 1 out]
            }
          }
        }
        frame True {
        }
      }
      n204 = Obtain Queue(element data type=i16[] [] ("2D array")) -> (queue out=w827:refnum<queue>, error out=w826:errorcluster)  [unwired: 3 in, 2 out]
      n205 = Unbundle By Name(w730) -> ("sessions out"=w760:refnum<k20>[], "SEM-X handle out"=w759:refnum<k15>, "SEM-Y handle out"=w753:refnum<k15>, "SEM-Y waveform handle out"=w755:i32, "Detectors handle out"=w749:refnum<k15>, "channels"=w750:string, "error out"=w751:errorcluster, "Others.AO SampClk.MaxRate"=w747:dbl, "Others.AI SampClk.MaxRate"=w746:dbl, "Others.AO rate"=w745:dbl, "Others.Scan speed"=w744:u8, "Others.Detector number"=w743:u8, "Others.X min (V)"=w742:dbl, "Others.X max (V)"=w741:dbl, "Others.X min index"=w740:i32, "Others.X max index"=w739:i32, "Others.AO multiline"=w738:u32, "Others.Decimating factor"=w731:u16, "Others.Total time"=w732:dbl, "Others.Scan time (m)"=w737:dbl, "Others.Scan time (s)"=w736:dbl, "Others.Y scan pts per line"=w758:i32, "Others.Y scan pts per AO multiline"=w756:i32, "Others.Small scan"=w754:bool, "Others.Y single line pattern"=w757:dbl[], "Others.Detectors min record length"=w752:u32, "Others.Waveform blocks"=w735:u32, "Others.Repeat count"=w734:u32)
      n206 = Unbundle By Name(w730) -> ("Others.AO rate"=w729:dbl, "Others.Decimating factor"=w728:u16, "Others.X resolution"=w721:u32, "Others.Y resolution"=w722:u32, "Others.X resolution with rampdown"=w727:i32, "Others.Oversampling"=w726:u32, "Others.Detector number"=w724:u8, "Others.AI multiline"=w725:u16)
      n207 = Quotient & Remainder(x=w722, y=w728) -> (floor(x/y)=w821:u32)  [unwired: 1 out]
      n208 = Quotient & Remainder(x=w721, y=w728) -> (floor(x/y)=w820:u32)  [unwired: 1 out]
      n209 = Initialize Array(i16 0 ("element"), w821, w820) -> (w782:i16[][])
      n210 = Initialize Array(i16 0 ("element"), w728, w820) -> (w781:i16[][])
      n211 = Compound Arithmetic op=MULTIPLY(w727, w724, w726) -> (w723:u32)
      n212 = case shown="True" w798 {
        tunnel: w782 -> [_ w982]
        tunnel: [w980 w982] -> w801
        tunnel: w781 -> [_ w981]
        tunnel: [w980 w981] -> w800
        tunnel: [w980 w981] -> w799
        tunnel: w777 -> [w980 _]
        frame False {
        }
        frame True {
        }
      }
      n213 = case shown="True" w792 {
        tunnel: w782 -> [_ w979]
        tunnel: [w977 w979] -> w795
        tunnel: w781 -> [_ w978]
        tunnel: [w977 w978] -> w796
        tunnel: [w977 w978] -> w797
        tunnel: w777 -> [w977 _]
        frame False {
        }
        frame True {
        }
      }
      n214 = case shown="True" w786 {
        tunnel: w782 -> [_ w976]
        tunnel: [w974 w976] -> w791
        tunnel: w781 -> [_ w975]
        tunnel: [w974 w975] -> w790
        tunnel: [w974 w975] -> w789
        tunnel: w777 -> [w974 _]
        frame False {
        }
        frame True {
        }
      }
      n215 = case shown="True" w783 {
        tunnel: w782 -> [_ w973]
        tunnel: [w971 w973] -> w779
        tunnel: w781 -> [_ w972]
        tunnel: [w971 w972] -> w780
        tunnel: [w971 w972] -> w778
        tunnel: w777 -> [w971 _]
        frame False {
        }
        frame True {
        }
      }
      n216 = Equal?(x=w724, y=u8 1 ("x")) -> (x = y?=w764:bool)
      n217 = Multiply(x=w735, y=w734) -> (x*y=w733:u32)
      n218 = local write "AO SampClk.MaxRate"(w747) -> ()
      n219 = local write "AI SampClk.MaxRate"(w746) -> ()
      n220 = local write "AO rate"(w745) -> ()
      n221 = local write "Scan speed"(w744) -> ()
      n222 = local write "Detector number"(w743) -> ()
      n223 = local write "X min (V)"(w742) -> ()
      n224 = local write "X max (V)"(w741) -> ()
      n225 = local write "X min index"(w740) -> ()
      n226 = local write "X max index"(w739) -> ()
      n227 = local write "AO multiline"(w738) -> ()
      n228 = local write "Decimating factor"(w731) -> ()
      n229 = local write "Total time"(w732) -> ()
      n230 = local write "Scan time (m)"(w737) -> ()
      n231 = local write "Scan time (s)"(w736) -> ()
      n232 = call <instrlib>:"niTClk Initiate.vi"("error in (no error)"=w751, "sessions"=w760) -> ("error out"=w765:errorcluster, "sessions out"=w709:refnum<k20>[])  [unwired: 8 in]
      n233 = local write "X resolution"(w721) -> ()
      n234 = local write "Y resolution"(w722) -> ()
      n235 = local write "Oversampling"(w726) -> ()
      n236 = local write "Detector number"(w724) -> ()
      n237 = To Long Integer(number=w722) -> (32bit integer=w828:i32)
      n238 = case shown="False" w754 {
        tunnel: w753 -> [w865 w921]
        tunnel: w755 -> [w863 _]
        tunnel: w758 -> [w853 _]
        tunnel: w751 -> [w862 w920]
        tunnel: w738 -> [w852 _]
        tunnel: [w860 w921] -> w769
        tunnel: [w858 w920] -> w767
        tunnel: w757 -> [w857 _]
        tunnel: w756 -> [w856 _]
        tunnel: w733 -> [w851 _]
        frame False {
          n239 = local read "Y resolution"() -> (w855:u32)
          n240 = while {
            tunnel: w852 -> [w874]
            tunnel: w865 -> [w895]
            tunnel: w857 -> [w876]
            tunnel: w853 -> [w877]
            shift-right: [w885] -> _
            shift-left: 1 -> [w873]
            tunnel: w863 -> [w893]
            tunnel: [w892] -> w861
            tunnel: w862 -> [w890]
            tunnel: [w889] -> w859
            tunnel: [w884] -> w854
            tunnel: w851 -> [_]
            tunnel: w856 -> [w882]
            tunnel: w855 -> [w879]
            stop <- w896 stop-if-true
            n241 = property class="niFgen"(reference=w895, error in=w890) -> (reference out=w894:refnum<k15>, error out=w891:errorcluster, "Arbitrary Waveform:Data Transfer:Streaming:Space Available in Streaming Waveform"=w886:i32)
            n242 = Multiply(x=w874, y=w873) -> (x*y=w875:u32)
            n243 = Less Or Equal?(x=w882, y=w886) -> (x <= y?=w878:bool)
            n244 = case shown="True" w878 {
              tunnel: [w899 w915] -> w892
              tunnel: w894 -> [w899 w914]
              tunnel: [w898 w913] -> w885
              tunnel: w873 -> [w898 w908]
              tunnel: w893 -> [_ w912]
              tunnel: w891 -> [w897 w911]
              tunnel: [w897 w910] -> w889
              tunnel: w874 -> [_ w907]
              tunnel: w877 -> [_ w901]
              tunnel: w876 -> [_ w909]
              tunnel: w875 -> [_ w906]
              frame False {
              }
              frame True {
                n245 = Increment(x=w908) -> (x+1=w913:i32)
                n246 = Array Subset(array=w909, index=w906, length=w907) -> (w903:dbl[])
                n247 = Array Size(array=w903) -> (size(s)=w902:i32)
                n248 = Multiply(x=w901, y=w902) -> (x*y=w900:i32)
                n249 = for {
                  tunnel: w903 -> [w916] mode=indexing
                  tunnel: [w918] -> w904 mode=indexing
                  tunnel: w901 -> [w917]
                  n250 = Initialize Array(w916, w917) -> (w918:dbl[])
                }
                n251 = Reshape Array(w904, w900) -> (w905:dbl[])
                n252 = call-poly <instrlib>:"niFgen Write Waveform (poly).vi"("Waveform Data"=w905, "error in (no error)"=w911, "Waveform Handle"=w912, "Instrument Handle"=w914) -> ("error out"=w910:errorcluster, "Instrument Handle Out"=w915:refnum<k15>)  [unwired: 5 in, 1 out]
              }
            }
            n253 = Multiply(x=w874, y=w885) -> (x*y=w881:u32)
            n254 = Unbundle By Name(w889) -> ("status"=w887:bool)
            n255 = local read "stop"() -> (w888:bool)
            n256 = In Range and Coerce(upper limit=w879, x=w881, lower limit=u32 0) -> (coerced(x)=w880:u32)  [unwired: 1 out]
            n257 = local write "AO scan line"(w880) -> ()
            n258 = Less Or Equal?(x=w879, y=w880) -> (x <= y?=w884:bool)
            n259 = Compound Arithmetic op=OR(w884, w887, w888) -> (w896:bool)
          }
          n260 = case shown="True" w854 {
            tunnel: w861 -> [w867 w872]
            tunnel: [w867 w871] -> w860
            tunnel: [w866 w869] -> w858
            tunnel: w859 -> [w866 w868]
            frame False {
            }
            frame True {
              n261 = call <instrlib>:"niFgen Wait Until Done.vi"("error in (no error)"=w868, "MaxTime (msec)"=30000, "Instrument Handle"=w872) -> ("error out"=w869:errorcluster, "Instrument Handle Out"=w871:refnum<k15>)  [unwired: 7 in]
            }
          }
        }
        frame True {
          n262 = local read "Y resolution"() -> (w919:u32)
          n263 = local write "AO scan line"(w919) -> ()
        }
      }
      n264 = Obtain Queue(element data type=i16[][] [] ("wfm")) -> (queue out=w819:refnum<queue>, error out=w836:errorcluster)  [unwired: 3 in, 2 out]
      n265 = while {
        tunnel: w827 -> [w1032]
        tunnel: w826 -> [w1031]
        tunnel: [w1030] -> w811
        tunnel: [w1029] -> w810
        shift-right: [w1005] -> _
        shift-left: w800 -> [w1028]
        shift-right: [w1027] -> _
        shift-left: w801 -> [w1006]
        shift-right: [w1021] -> _
        shift-left: w796 -> [w1003]
        shift-right: [w1004] -> _
        shift-left: w795 -> [w1015]
        shift-right: [w1025] -> _
        shift-left: 0 -> [w1007]
        tunnel: [w1026] -> w817
        tunnel: [w1024] -> w812
        tunnel: w799 -> [w1022]
        tunnel: w797 -> [w1020]
        shift-right: [w1002] -> _
        shift-left: w791 -> [w1014]
        shift-right: [w1001] -> _
        shift-left: w790 -> [w1019]
        tunnel: w789 -> [w1018]
        shift-right: [w1000] -> _
        shift-left: w779 -> [w1013]
        shift-right: [w999] -> _
        shift-left: w780 -> [w1017]
        tunnel: w778 -> [w1016]
        tunnel: w819 -> [w1012]
        tunnel: [w1011] -> w818
        tunnel: w725 -> [w1008]
        tunnel: [w994] -> w776
        tunnel: w723 -> [w995]
        tunnel: w764 -> [w992]
        tunnel: w729 -> [w990]
        tunnel: w728 -> [w989]
        i -> [w1023]
        stop <- w994 stop-if-true
        n266 = Dequeue Element(queue=w1012) -> (queue out=w1011:refnum<queue>, element=w997:i16[][], error out=w1026:errorcluster)  [unwired: 1 in, 2 out]
        n267 = Multiply(x=w1008, y=w1023) -> (x*y=w1009:i32)
        n268 = case shown="False" w992 {
          tunnel: w997 -> [w1034 w1035]
          tunnel: [w1033 w1035] -> w996
          frame False {
            n269 = Transpose 2D Array(2D array=w1034) -> (transposed array=w1033:i16[][])
          }
          frame True {
          }
        }
        n270 = Wait Until Next ms Multiple(millisecond multiple=u32 5) -> ()  [unwired: 1 out]
        n271 = Reshape Array(w996, w1008, w995) -> (w1010:i16[][])
        n272 = for {
          tunnel: w1032 -> [w1146]
          tunnel: w1031 -> [w1145]
          tunnel: [w1144] -> w1030
          tunnel: [w1143] -> w1029
          tunnel: [w1132] -> w993
          tunnel: w1010 -> [w1130] mode=indexing
          tunnel: w1009 -> [w1112]
          tunnel: w1022 -> [w1111]
          tunnel: w1020 -> [w1109]
          tunnel: w1018 -> [w1091]
          tunnel: w1016 -> [w1088]
          shift-right: [w1064] -> w1025
          shift-left: w1007 -> [w1085]
          shift-right: [w1137] -> w1027
          shift-left: w1006 -> [w1065]
          shift-right: [w1084] -> w1005
          shift-left: w1028 -> [w1138]
          shift-right: [w1083] -> w1004
          shift-left: w1015 -> [w1066]
          shift-right: [w1110] -> w1021
          shift-left: w1003 -> [w1082]
          shift-right: [w1081] -> w1002
          shift-left: w1014 -> [w1067]
          shift-right: [w1080] -> w1001
          shift-left: w1019 -> [w1092]
          shift-right: [w1079] -> w1000
          shift-left: w1013 -> [w1068]
          shift-right: [w1078] -> w999
          shift-left: w1017 -> [w1089]
          tunnel: w990 -> [w1039]
          tunnel: w989 -> [w1036]
          i -> [w1086]
          n273 = Add(x=w1086, y=w1112) -> (x+y=w1087:i32)
          n274 = local read "Oversampling"() -> (w1140:u32)
          n275 = local read "Detector A"() -> (w1123:bool)
          n276 = local read "Detector C"() -> (w1108:bool)
          n277 = local read "Detector D"() -> (w1107:bool)
          n278 = local read "Detector B"() -> (w1124:bool)
          n279 = local read "X resolution"() -> (w1139:u32)
          n280 = local read "DetA-Rate"() -> (w1040:sgl)
          n281 = local read "DetA-Scaling"() -> (w1043:sgl)
          n282 = local read "DetB-Rate"() -> (w1041:sgl)
          n283 = local read "DetB-Scaling"() -> (w1044:sgl)
          n284 = Build Array(w1123, w1124, w1108, w1107) -> (w1125:bool[])
          n285 = Divide(x=w1040, y=w1039) -> (x/y=w1042:dbl)
          n286 = Divide(x=w1041, y=w1039) -> (x/y=w1045:dbl)
          n287 = To Long Integer(number=w1140) -> (32bit integer=w1102:i32)
          n288 = To Long Integer(number=w1139) -> (32bit integer=w1099:i32)
          n289 = Multiply(x=w1042, y=w1043) -> (x*y=w1038:dbl)
          n290 = Multiply(x=w1045, y=w1044) -> (x*y=w1037:dbl)
          n291 = Boolean Array To Number(Boolean array=w1125) -> (number=w1122:u32)
          n292 = case shown="1, Default" w1122 {
            tunnel: [w1274 _ w1278 _ w1282 _ w1289 _ w1293 _ w1300 _ w1307 _ w1316] -> w1131
            tunnel: w1130 -> [w1274 w1275 w1276 w1279 w1280 w1283 w1286 w1290 w1291 w1294 w1297 w1301 w1304 w1308 w1312]
            tunnel: [_ w1275 w1277 _ _ w1285 w1288 _ _ w1296 w1299 _ _ w1311 w1315] -> w1126
            tunnel: [_ _ _ w1279 w1281 w1284 w1287 _ _ _ _ w1303 w1306 w1309 w1314] -> w1101
            tunnel: [_ _ _ _ _ _ _ w1290 w1292 w1295 w1298 w1302 w1305 w1310 w1313] -> w1100
            frame 1, Default {
            }
            frame 2 {
            }
            frame 3 {
              n293 = Decimate 1D Array(w1276) -> (w1278:i16[], w1277:i16[])
            }
            frame 4 {
            }
            frame 5 {
              n294 = Decimate 1D Array(w1280) -> (w1282:i16[], w1281:i16[])
            }
            frame 6 {
              n295 = Decimate 1D Array(w1283) -> (w1285:i16[], w1284:i16[])
            }
            frame 7 {
              n296 = Decimate 1D Array(w1286) -> (w1289:i16[], w1288:i16[], w1287:i16[])
            }
            frame 8 {
            }
            frame 9 {
              n297 = Decimate 1D Array(w1291) -> (w1293:i16[], w1292:i16[])
            }
            frame 10 {
              n298 = Decimate 1D Array(w1294) -> (w1296:i16[], w1295:i16[])
            }
            frame 11 {
              n299 = Decimate 1D Array(w1297) -> (w1300:i16[], w1299:i16[], w1298:i16[])
            }
            frame 12 {
              n300 = Decimate 1D Array(w1301) -> (w1303:i16[], w1302:i16[])
            }
            frame 13 {
              n301 = Decimate 1D Array(w1304) -> (w1307:i16[], w1306:i16[], w1305:i16[])
            }
            frame 14 {
              n302 = Decimate 1D Array(w1308) -> (w1311:i16[], w1309:i16[], w1310:i16[])
            }
            frame 15 {
              n303 = Decimate 1D Array(w1312) -> (w1316:i16[], w1315:i16[], w1314:i16[], w1313:i16[])
            }
          }
          n304 = To Double Precision Float(number=w1131) -> (double precision float=w1121:dbl[])
          n305 = To Double Precision Float(number=w1126) -> (double precision float=w1120:dbl[])
          n306 = To Double Precision Float(number=w1101) -> (double precision float=w1105:dbl[])
          n307 = To Double Precision Float(number=w1100) -> (double precision float=w1106:dbl[])
          n308 = local read "8-bit"() -> (w1054:bool)
          n309 = To Long Integer(number=w1036) -> (32bit integer=w1093:i32)
          n310 = call-poly <vilib>:"Decimate (single shot).vi"("averaging"=TRUE, "decimating factor"=w1102, "X"=w1121) -> ("Decimated Array"=w1136:dbl[])  [unwired: 8 out]
          n311 = call-poly <vilib>:"Decimate (single shot).vi"("averaging"=TRUE, "decimating factor"=w1102, "X"=w1120) -> ("Decimated Array"=w1057:dbl[])  [unwired: 8 out]
          n312 = call-poly <vilib>:"Decimate (single shot).vi"("averaging"=TRUE, "decimating factor"=w1102, "X"=w1105) -> ("Decimated Array"=w1056:dbl[])  [unwired: 8 out]
          n313 = call-poly <vilib>:"Decimate (single shot).vi"("averaging"=TRUE, "decimating factor"=w1102, "X"=w1106) -> ("Decimated Array"=w1055:dbl[])  [unwired: 8 out]
          n314 = Quotient & Remainder(x=w1087, y=w1093) -> (x-y*floor(x/y)=w1062:i32, floor(x/y)=w1094:i32)
          n315 = Increment(x=w1062) -> (x+1=w1063:i32)
          n316 = case shown="True" w1054 {
            tunnel: [w1166 w1169] -> w1053
            tunnel: w1136 -> [w1166 w1171]
            tunnel: w1038 -> [_ w1168]
            frame False {
            }
            frame True {
              n317 = local read "DetA-Io"() -> (w1172:sgl)
              n318 = local read "DetA-k"() -> (w1167:sgl)
              n319 = Subtract(x=w1171, y=w1172) -> (x-y=w1170:dbl[])
              n320 = Compound Arithmetic op=MULTIPLY(w1170, w1167, w1168) -> (w1169:dbl[])
            }
          }
          n321 = case shown="True" w1054 {
            tunnel: [w1159 w1162] -> w1051
            tunnel: w1057 -> [w1159 w1164]
            tunnel: w1037 -> [_ w1161]
            frame False {
            }
            frame True {
              n322 = local read "DetB-Io"() -> (w1165:sgl)
              n323 = local read "DetB-k"() -> (w1160:sgl)
              n324 = Subtract(x=w1164, y=w1165) -> (x-y=w1163:dbl[])
              n325 = Compound Arithmetic op=MULTIPLY(w1163, w1160, w1161) -> (w1162:dbl[])
            }
          }
          n326 = case shown="True" w1054 {
            tunnel: [w1153 w1154] -> w1049
            tunnel: w1056 -> [w1153 w1157]
            frame False {
            }
            frame True {
              n327 = local read "DetC-Io"() -> (w1158:sgl)
              n328 = local read "DetC-k"() -> (w1155:sgl)
              n329 = Subtract(x=w1157, y=w1158) -> (x-y=w1156:dbl[])
              n330 = Multiply(x=w1156, y=w1155) -> (x*y=w1154:dbl[])
            }
          }
          n331 = case shown="True" w1054 {
            tunnel: [w1147 w1148] -> w1047
            tunnel: w1055 -> [w1147 w1151]
            frame False {
            }
            frame True {
              n332 = local read "DetD-Io"() -> (w1152:sgl)
              n333 = local read "DetD-k"() -> (w1149:sgl)
              n334 = Subtract(x=w1151, y=w1152) -> (x-y=w1150:dbl[])
              n335 = Multiply(x=w1150, y=w1149) -> (x*y=w1148:dbl[])
            }
          }
          n336 = Equal?(x=w1063, y=w1093) -> (x = y?=w1090:bool)
          n337 = To Word Integer(number=w1053) -> (16bit integer=w1052:i16[])
          n338 = To Word Integer(number=w1051) -> (16bit integer=w1050:i16[])
          n339 = To Word Integer(number=w1049) -> (16bit integer=w1048:i16[])
          n340 = To Word Integer(number=w1047) -> (16bit integer=w1046:i16[])
          n341 = Array Subset(array=w1052, length=w1099) -> (w1129:i16[])  [unwired: 1 in]
          n342 = Array Subset(array=w1050, length=w1099) -> (w1128:i16[])  [unwired: 1 in]
          n343 = Array Subset(array=w1048, length=w1099) -> (w1097:i16[])  [unwired: 1 in]
          n344 = Array Subset(array=w1046, length=w1099) -> (w1096:i16[])  [unwired: 1 in]
          n345 = local read "Detector A"() -> (w1077:bool)
          n346 = local read "Display"() -> (w1069:bool)
          n347 = local read "Detector B"() -> (w1075:bool)
          n348 = local read "Detector C"() -> (w1072:bool)
          n349 = local read "Detector D"() -> (w1070:bool)
          n350 = case shown="4" w1122 {
            tunnel: w1129 -> [w1231 _ w1235 _ w1238 _ w1246 _ w1250 _ w1257 _ w1264 _ w1273]
            tunnel: w1128 -> [_ w1232 w1234 _ _ w1242 w1245 _ _ w1253 w1256 _ _ w1268 w1272]
            tunnel: [w1231 w1232 w1233 w1236 w1239 w1240 w1243 w1247 w1248 w1251 w1254 w1258 w1261 w1265 w1269] -> w1127
            tunnel: w1097 -> [_ _ _ w1236 w1237 w1241 w1244 _ _ _ _ w1259 w1263 w1267 w1271]
            tunnel: w1096 -> [_ _ _ _ _ _ _ w1247 w1249 w1252 w1255 w1260 w1262 w1266 w1270]
            frame 1, Default {
            }
            frame 2 {
            }
            frame 3 {
              n351 = Interleave 1D Arrays(w1235, w1234) -> (w1233:i16[])
            }
            frame 4 {
            }
            frame 5 {
              n352 = Interleave 1D Arrays(w1238, w1237) -> (w1239:i16[])
            }
            frame 6 {
              n353 = Interleave 1D Arrays(w1242, w1241) -> (w1240:i16[])
            }
            frame 7 {
              n354 = Interleave 1D Arrays(w1246, w1245, w1244) -> (w1243:i16[])
            }
            frame 8 {
            }
            frame 9 {
              n355 = Interleave 1D Arrays(w1250, w1249) -> (w1248:i16[])
            }
            frame 10 {
              n356 = Interleave 1D Arrays(w1253, w1252) -> (w1251:i16[])
            }
            frame 11 {
              n357 = Interleave 1D Arrays(w1257, w1256, w1255) -> (w1254:i16[])
            }
            frame 12 {
              n358 = Interleave 1D Arrays(w1259, w1260) -> (w1258:i16[])
            }
            frame 13 {
              n359 = Interleave 1D Arrays(w1264, w1263, w1262) -> (w1261:i16[])
            }
            frame 14 {
              n360 = Interleave 1D Arrays(w1268, w1267, w1266) -> (w1265:i16[])
            }
            frame 15 {
              n361 = Interleave 1D Arrays(w1273, w1272, w1271, w1270) -> (w1269:i16[])
            }
          }
          n362 = To Double Precision Float(number=w1129) -> (double precision float=w1113:dbl[])
          n363 = To Double Precision Float(number=w1128) -> (double precision float=w1114:dbl[])
          n364 = To Double Precision Float(number=w1097) -> (double precision float=w1098:dbl[])
          n365 = To Double Precision Float(number=w1096) -> (double precision float=w1095:dbl[])
          n366 = And(x=w1077, y=w1069) -> (x .and. y?=w1076:bool)
          n367 = And(x=w1069, y=w1075) -> (x .and. y?=w1074:bool)
          n368 = And(x=w1069, y=w1072) -> (x .and. y?=w1073:bool)
          n369 = And(x=w1069, y=w1070) -> (x .and. y?=w1071:bool)
          n370 = local read "Save"() -> (w1059:bool)
          n371 = local read "Detector number"() -> (w1117:u8)
          n372 = case shown="True" w1076 {
            tunnel: w1113 -> [_ w1359]
            tunnel: w1138 -> [w1346 w1354]
            tunnel: [w1347 w1362] -> w1137
            tunnel: w1065 -> [w1347 w1361]
            tunnel: w1093 -> [_ w1357]
            tunnel: [w1346 w1360] -> w1084
            tunnel: w1062 -> [_ w1353]
            tunnel: w1111 -> [_ w1352]
            tunnel: w1090 -> [_ w1348]
            tunnel: w1094 -> [_ w1349]
            frame False {
            }
            frame True {
              n373 = call-poly <vilib>:"Decimate (single shot).vi"("averaging"=TRUE, "decimating factor"=w1357, "X"=w1359) -> ("Decimated Array"=w1351:dbl[])  [unwired: 8 out]
              n374 = To Word Integer(number=w1351) -> (16bit integer=w1355:i16[])
              n375 = Replace Array Subset(array=w1354, new element=w1355, index (row)=w1353) -> (w1356:i16[][])  [unwired: 1 in]
              n376 = Array Size(array=w1351) -> (size(s)=w1350:i32)
              n377 = case shown="True" w1348 {
                tunnel: [w1364 w1365] -> w1362
                tunnel: w1361 -> [w1364 w1367]
                tunnel: w1357 -> [_ w1374]
                tunnel: [w1363 w1372] -> w1360
                tunnel: w1356 -> [w1363 w1373]
                tunnel: w1352 -> [_ w1372]
                tunnel: w1350 -> [_ w1368]
                tunnel: w1349 -> [_ w1366]
                frame False {
                }
                frame True {
                  n378 = call "2D Array Decimate.vi"("y decimating factor"=w1374, "Input 2D Array"=w1373) -> ("output array"=w1369:dbl[][])  [unwired: 2 in, 7 out]
                  n379 = To Word Integer(number=w1369) -> (16bit integer=w1370:i16[][])
                  n380 = Reshape Array(w1370, w1368) -> (w1371:i16[])
                  n381 = Replace Array Subset(array=w1367, new element=w1371, index (row)=w1366) -> (w1365:i16[][])  [unwired: 1 in]
                  "Det A Img" <- w1365
                  n382 = shared-variable ".\\Zeiss Library.lvlib\\Det A Img"(w1365) -> ()  [unwired: 2 out]
                }
              }
            }
          }
          n383 = case shown="True" w1074 {
            tunnel: w1093 -> [_ w1329]
            tunnel: w1114 -> [_ w1330]
            tunnel: w1082 -> [w1317 w1321]
            tunnel: [w1318 w1333] -> w1083
            tunnel: w1066 -> [w1318 w1332]
            tunnel: w1090 -> [_ w1328]
            tunnel: w1094 -> [_ w1327]
            tunnel: w1062 -> [_ w1325]
            tunnel: [w1317 w1320] -> w1110
            tunnel: w1109 -> [_ w1319]
            frame False {
            }
            frame True {
              n384 = call-poly <vilib>:"Decimate (single shot).vi"("averaging"=TRUE, "decimating factor"=w1329, "X"=w1330) -> ("Decimated Array"=w1324:dbl[])  [unwired: 8 out]
              n385 = To Word Integer(number=w1324) -> (16bit integer=w1326:i16[])
              n386 = Replace Array Subset(array=w1321, new element=w1326, index (row)=w1325) -> (w1323:i16[][])  [unwired: 1 in]
              n387 = Array Size(array=w1324) -> (size(s)=w1322:i32)
              n388 = case shown="True" w1328 {
                tunnel: w1329 -> [_ w1345]
                tunnel: [w1335 w1336] -> w1333
                tunnel: w1332 -> [w1335 w1343]
                tunnel: w1327 -> [_ w1342]
                tunnel: w1323 -> [w1334 w1338]
                tunnel: w1322 -> [_ w1339]
                tunnel: [w1334 w1337] -> w1320
                tunnel: w1319 -> [_ w1337]
                frame False {
                }
                frame True {
                  n389 = call "2D Array Decimate.vi"("y decimating factor"=w1345, "Input 2D Array"=w1338) -> ("output array"=w1344:dbl[][])  [unwired: 2 in, 7 out]
                  n390 = To Word Integer(number=w1344) -> (16bit integer=w1340:i16[][])
                  n391 = Reshape Array(w1340, w1339) -> (w1341:i16[])
                  n392 = Replace Array Subset(array=w1343, new element=w1341, index (row)=w1342) -> (w1336:i16[][])  [unwired: 1 in]
                  "Det B Img" <- w1336
                  n393 = shared-variable ".\\Zeiss Library.lvlib\\Det B Img"(w1336) -> ()  [unwired: 2 out]
                }
              }
            }
          }
          n394 = case shown="True" w1073 {
            tunnel: w1093 -> [_ w1214]
            tunnel: w1098 -> [_ w1215]
            tunnel: w1092 -> [w1202 w1206]
            tunnel: [w1203 w1218] -> w1081
            tunnel: w1067 -> [w1203 w1217]
            tunnel: w1090 -> [_ w1213]
            tunnel: w1094 -> [_ w1212]
            tunnel: w1062 -> [_ w1210]
            tunnel: [w1202 w1205] -> w1080
            tunnel: w1091 -> [_ w1204]
            frame False {
            }
            frame True {
              n395 = call-poly <vilib>:"Decimate (single shot).vi"("averaging"=TRUE, "decimating factor"=w1214, "X"=w1215) -> ("Decimated Array"=w1209:dbl[])  [unwired: 8 out]
              n396 = To Word Integer(number=w1209) -> (16bit integer=w1211:i16[])
              n397 = Replace Array Subset(array=w1206, new element=w1211, index (row)=w1210) -> (w1208:i16[][])  [unwired: 1 in]
              n398 = Array Size(array=w1209) -> (size(s)=w1207:i32)
              n399 = case shown="True" w1213 {
                tunnel: w1214 -> [_ w1230]
                tunnel: [w1220 w1221] -> w1218
                tunnel: w1217 -> [w1220 w1228]
                tunnel: w1212 -> [_ w1227]
                tunnel: w1208 -> [w1219 w1223]
                tunnel: w1207 -> [_ w1224]
                tunnel: [w1219 w1222] -> w1205
                tunnel: w1204 -> [_ w1222]
                frame False {
                }
                frame True {
                  n400 = call "2D Array Decimate.vi"("y decimating factor"=w1230, "Input 2D Array"=w1223) -> ("output array"=w1229:dbl[][])  [unwired: 2 in, 7 out]
                  n401 = To Word Integer(number=w1229) -> (16bit integer=w1225:i16[][])
                  n402 = Reshape Array(w1225, w1224) -> (w1226:i16[])
                  n403 = Replace Array Subset(array=w1228, new element=w1226, index (row)=w1227) -> (w1221:i16[][])  [unwired: 1 in]
                  "Det C Img" <- w1221
                  n404 = shared-variable ".\\Zeiss Library.lvlib\\Det C Img"(w1221) -> ()  [unwired: 2 out]
                }
              }
            }
          }
          n405 = case shown="True" w1071 {
            tunnel: w1093 -> [_ w1185]
            tunnel: w1095 -> [_ w1186]
            tunnel: w1089 -> [w1173 w1177]
            tunnel: [w1174 w1189] -> w1079
            tunnel: w1068 -> [w1174 w1188]
            tunnel: w1090 -> [_ w1184]
            tunnel: w1094 -> [_ w1183]
            tunnel: w1062 -> [_ w1181]
            tunnel: [w1173 w1176] -> w1078
            tunnel: w1088 -> [_ w1175]
            frame False {
            }
            frame True {
              n406 = call-poly <vilib>:"Decimate (single shot).vi"("averaging"=TRUE, "decimating factor"=w1185, "X"=w1186) -> ("Decimated Array"=w1180:dbl[])  [unwired: 8 out]
              n407 = To Word Integer(number=w1180) -> (16bit integer=w1182:i16[])
              n408 = Replace Array Subset(array=w1177, new element=w1182, index (row)=w1181) -> (w1179:i16[][])  [unwired: 1 in]
              n409 = Array Size(array=w1180) -> (size(s)=w1178:i32)
              n410 = case shown="True" w1184 {
                tunnel: w1185 -> [_ w1201]
                tunnel: [w1191 w1192] -> w1189
                tunnel: w1188 -> [w1191 w1199]
                tunnel: w1183 -> [_ w1198]
                tunnel: w1179 -> [w1190 w1194]
                tunnel: w1178 -> [_ w1195]
                tunnel: [w1190 w1193] -> w1176
                tunnel: w1175 -> [_ w1193]
                frame False {
                }
                frame True {
                  n411 = call "2D Array Decimate.vi"("y decimating factor"=w1201, "Input 2D Array"=w1194) -> ("output array"=w1200:dbl[][])  [unwired: 2 in, 7 out]
                  n412 = To Word Integer(number=w1200) -> (16bit integer=w1196:i16[][])
                  n413 = Reshape Array(w1196, w1195) -> (w1197:i16[])
                  n414 = Replace Array Subset(array=w1199, new element=w1197, index (row)=w1198) -> (w1192:i16[][])  [unwired: 1 in]
                  "Det D Img" <- w1192
                  n415 = shared-variable ".\\Zeiss Library.lvlib\\Det D Img"(w1192) -> ()  [unwired: 2 out]
                }
              }
            }
          }
          n416 = Array Size(array=w1127) -> (size(s)=w1118:i32)
          n417 = local read "PNG only"() -> (w1061:bool)
          n418 = Not(x=w1061) -> (.not. x?=w1060:bool)
          n419 = To Long Integer(number=w1117) -> (32bit integer=w1116:i32)
          n420 = And(x=w1059, y=w1060) -> (x .and. y?=w1058:bool)
          n421 = Quotient & Remainder(x=w1118, y=w1116) -> (floor(x/y)=w1119:i32)  [unwired: 1 out]
          n422 = Add(x=w1119, y=w1085) -> (x+y=w1064:i32)
          n423 = case shown="True" w1058 {
            tunnel: w1146 -> [w1376 w1381]
            tunnel: w1145 -> [w1375 w1380]
            tunnel: [w1376 w1379] -> w1144
            tunnel: [w1375 w1378] -> w1143
            tunnel: w1127 -> [_ w1377]
            frame False {
            }
            frame True {
              n424 = Enqueue Element(queue=w1381, element=w1377, error in (no error)=w1380) -> (queue out=w1379:refnum<queue>, error out=w1378:errorcluster)  [unwired: 2 out]
            }
          }
          n425 = local write "Total pixels recorded"(w1064) -> ()
          n426 = local read "X resolution"() -> (w1135:u32)
          n427 = local read "Y resolution"() -> (w1134:u32)
          n428 = Multiply(x=w1135, y=w1134) -> (x*y=w1133:u32)
          n429 = To Unsigned Long Integer(number=w1064) -> (unsigned 32bit integer=w1115:u32)
          n430 = Greater Or Equal?(x=w1115, y=w1133) -> (x >= y?=w1132:bool)
        }
        n431 = Unbundle By Name(w1026) -> ("status"=w1024:bool)
        n432 = local read "stop"() -> (w998:bool)
        n433 = Compound Arithmetic op=OR(w993, w1024, w998) -> (w994:bool)
      }
      n434 = while {
        tunnel: w819 -> [w2262]
        tunnel: w836 -> [w2261]
        tunnel: [w2260] -> w835
        tunnel: [w2259] -> w833
        tunnel: w828 -> [w2239]
        tunnel: w725 -> [w2244]
        tunnel: w749 -> [w2257]
        tunnel: w751 -> [w2256]
        tunnel: w752 -> [w2255]
        tunnel: [w2250] -> w772
        tunnel: [w2253] -> w768
        tunnel: w750 -> [w2254]
        tunnel: [w2247] -> w773
        tunnel: w709 -> [_]
        shift-right: [w2236] -> w706
        shift-left: sgl[][] [] -> [w2235]
        i -> [w2245]
        stop <- w2258 stop-if-true
        n435 = Increment(x=w2245) -> (x+1=w2246:i32)
        n436 = call-poly <instrlib>:"niScope Fetch (poly).vi"("error in"=w2256, "numSamples"=w2255, "channels"=w2254, "instrument handle"=w2257) -> ("error out"=w2252:errorcluster, "wfm"=w2248:i16[][], "instrument handle out"=w2251:refnum<k15>)  [unwired: 4 in, 1 out]
        n437 = Multiply(x=w2244, y=w2246) -> (x*y=w2240:i32)
        n438 = property class="niScope"(reference=w2251, error in=w2252) -> (reference out=w2250:refnum<k15>, error out=w2253:errorcluster, "Fetch Backlog"=w2249:dbl)
        n439 = In Range and Coerce(upper limit=w2239, x=w2240, lower limit=0) -> (coerced(x)=w2243:i32)  [unwired: 1 out]
        n440 = local write "AvailSampPerChan"(w2249) -> ()
        n441 = shared-variable ".\\Zeiss Library.lvlib\\Logs"() -> (w2237:sgl[])  [unwired: 1 in, 1 out]
        n442 = local write "Total lines scanned"(w2243) -> ()
        n443 = Greater Or Equal?(x=w2240, y=w2239) -> (x >= y?=w2241:bool)
        n444 = Build Array (concatenate)(w2235, w2237) -> (w2236:sgl[][])
        n445 = Enqueue Element(queue=w2262, element=w2248, error in (no error)=w2261) -> (queue out=w2260:refnum<queue>, error out=w2259:errorcluster)  [unwired: 2 out]
        n446 = Unbundle By Name(w2253) -> ("status"=w2247:bool)
        n447 = local read "stop"() -> (w2242:bool)
        n448 = Compound Arithmetic op=OR(w2247, w2241, w2242) -> (w2258:bool)
      }
      n449 = Array Size(array=w706) -> (size(s)=w707:i32[])
      n450 = Index Array(array=w707) -> (element=w700:i32)  [unwired: 1 in]
      n451 = call <instrlib>:"niScope Abort.vi"("instrument handle"=w772, "error in"=w768) -> ("error out"=w748:errorcluster)  [unwired: 12 in, 1 out]
      n452 = Subtract(x=w700, y=w698) -> (x-y=w699:i32)
      n453 = Array Subset(array=w706, index (row)=w698, index (col)=w701, length (col)=w701) -> (w705:sgl[][])  [unwired: 1 in]
      n454 = Reshape Array(w705, w699) -> (w704:sgl[])
      n455 = call-poly <vilib>:"Basic Averaged DC-RMS.vi"("signal in"=w704) -> ("DC value"=w702:dbl)  [unwired: 7 in, 3 out]
      n456 = To Single Precision Float(number=w702) -> (single precision float=w703:sgl)
      n457 = local write "SEM Spec. I (nA)"(w703) -> ()
      n458 = Get Queue Status(queue=w835, error in (no error)=w833) -> (queue out=w834:refnum<queue>, error out=w832:errorcluster, # elements in queue=w831:i32)  [unwired: 6 out]
      n459 = Build Array(w759, w769) -> (w771:refnum<k15>[])
      n460 = Merge Errors(w767, w748) -> (w766:errorcluster)
      n461 = Equal To 0?(x=w831) -> (x = 0?=w830:bool)
      n462 = for {
        tunnel: w771 -> [w924] mode=indexing
        shift-right: [w922] -> w762
        shift-left: w766 -> [w923]
        n463 = call <instrlib>:"niFgen Abort Generation.vi"("error in (no error)"=w923, "Instrument Handle"=w924) -> ("error out"=w922:errorcluster)  [unwired: 8 in, 1 out]
      }
      n464 = Compound Arithmetic op=OR(w830, w773) -> (w829:bool)
      n465 = case shown="True" w829 {
        tunnel: w834 -> [_ w2234]
        tunnel: w832 -> [w2231 w2233]
        tunnel: [w2231 w2232] -> w770
        frame False {
        }
        frame True {
          n466 = Release Queue(queue=w2234, error in (no error)=w2233) -> (error out=w2232:errorcluster)  [unwired: 3 out]
        }
      }
      n467 = Generate Occurrence() -> (w775:refnum<k4>)
      n468 = case shown="True" w806 {
        tunnel: w827 -> [_ w1387]
        tunnel: [_ w1386] -> w809
        tunnel: [_ w1385] -> w808
        tunnel: w775 -> [_ w1384]
        tunnel: w749 -> [_ w1383]
        tunnel: w729 -> [_ w1382]
        frame False {
        }
        frame True {
          n469 = stacked-sequence {
            tunnel: w1387 -> [_ _ w1537 _ _]
            tunnel: [_ _ w1536 _ _] -> w1386
            tunnel: [_ _ w1535 _ _] -> w1385
            tunnel: w1384 -> [_ _ w1533 _ _]
            tunnel: w1383 -> [_ _ w1532 _ _]
            tunnel: w1382 -> [_ _ w1531 w1943 _]
            frame #0 {
              w1389 = "-" ("string")
              w1398 = "_" ("string")
              n470 = local read "Machine ID"() -> (w1403:string)
              n471 = local read "Tile index"() -> (w1391:u8[])
              n472 = local read "Frame"() -> (w1388:u8)
              n473 = Format Into String(w1388) -> (resulting string=w1390:string)  [unwired: 3 in, 1 out]
              n474 = Index Array(array=w1391) -> (element #1=w1393:u8, element #2=w1392:u8)  [unwired: 2 in]
              n475 = Compound Arithmetic op=ADD(w1392, w1393, w1388) -> (w1394:u8)
              n476 = Equal To 0?(x=w1394) -> (x = 0?=w1395:bool)
              n477 = case shown="False" w1395 {
                tunnel: [w1415 w1416] -> w1401
                frame False {
                  n478 = local read "Timestamp"() -> (w1415:timestamp)
                }
                frame True {
                  n479 = Get Date/Time In Seconds() -> (seconds since 1Jan1904=w1416:timestamp)
                }
              }
              "Timestamp" <- w1401
              n480 = local read "File path"() -> (w1406:path)
              n481 = xnode "Match Regular Expression"("input string"=w1403, "regular expression"="/") -> ("after match"=w1404:string)  [unwired: 4 in, 4 out]
              n482 = Format Date/Time String(time format string (%c)="%y-%m-%d_%H%M%S", seconds (now)=w1401) -> (date/time string=w1409:string)  [unwired: 1 out]
              n483 = Format Into String(w1393) -> (resulting string=w1397:string)  [unwired: 3 in, 1 out]
              n484 = Format Into String(w1392) -> (resulting string=w1396:string)  [unwired: 3 in, 1 out]
              n485 = Format Date/Time String(time format string (%c)="Y%Y\\M%m\\D%d", seconds (now)=w1401) -> (date/time string=w1402:string)  [unwired: 1 out]
              n486 = Build Path(base path=w1406, name or relative path=w1402) -> (appended path=w1407:path)
              n487 = Concatenate Strings(w1404, w1398, w1409, w1398, w1390, w1389, w1397, w1389, w1396, ".dat" ("string")) -> (w1400:string)
              n488 = File/Directory Info(path=w1407) -> (path out=w1414:path, error out=w1412:errorcluster)  [unwired: 1 in, 5 out]
              n489 = Build Path(base path=w1407, name or relative path=w1400) -> (appended path=→"File name":path)
              n490 = Unbundle By Name(w1412) -> ("status"=w1413:bool)
              n491 = case shown="True" w1413 {
                tunnel: w1414 -> [_ w1528]
                frame False {
                }
                frame True {
                  n492 = Create Folder(path (use dialog)=w1528) -> ()  [unwired: 1 in, 4 out]
                }
              }
            }
            frame #1 {
              n493 = local read "PNG only"() -> (w1529:bool)
              n494 = case shown="False" w1529 {
                frame False {
                  "Runsheet header array" <- string[] ["Date", "Time", "Notes", "Detector A", "Detector B", "Detector C", "Detector D", "Detectors", "X resolution", "Y resolution", "Rate (Hz)", "Brightness A (%)", "Contrast A (%)", "Brightness B (%)", "Contrast B (%)", "Magnification", "Pixel size (nm)", "Working Distance (mm)", "EHT (kV)", "Aperture #", "High Current Mode", "Probe Current (A)", "Beam Shift X", "Beam Shift Y", "Stigmation X", "Stigmation Y", "Alignment X", "Alignment Y", "FIB spacing (nm)", "A Img Focus Index", "B Img Focus Index", "A Img Primary Grid Mean", "A Img Primary Grid Std", "B Img Primary Grid Mean", "B Img Primary Grid Std", "Temp (F)", "FIB Faraday Cup (nA)", "Specimen I (nA)", "Milling Beam Dump 1 (nA)", "Milling Beam Dump 2 (nA)", "Milling I (nA)", "SEM Specimen I (nA)", "Milling Z voltage (V)", "Image Delta X (nm)", "Image Delta Y (nm)", "Image Delta Z"]
                }
                frame True {
                }
              }
            }
            frame #2 {
              n495 = local read "PNG only"() -> (w1534:bool)
              n496 = case shown="False" w1534 {
                tunnel: w1537 -> [w1704 _]
                tunnel: [w1703 _] -> w1536
                tunnel: [w1702 _] -> w1535
                tunnel: w1533 -> [_ w1942]
                tunnel: w1532 -> [w1603 _]
                tunnel: w1531 -> [w1555 _]
                frame False {
                  w1653 = u8 1 ("lower limit")
                  w1716 = "\"" ("string")
                  w1737 = T17 3 items=["no dialog", "OK message", "continue or stop message", "OK message + warnings", "continue/stop + warnings"] ("type of dialog (OK msg:1)")
                  n497 = property class="niScope"(reference=w1603) -> ("Actual Sample Rate"=w1607:dbl)  [unwired: 1 in, 2 out]
                  n498 = local read "8-bit"() -> (w1572:bool)
                  n499 = local read "8-bit coefficents"() -> (w1561:sgl[][])
                  n500 = local read "Detector A"() -> (w1728:bool)
                  n501 = local read "Detector C"() -> (w1709:bool)
                  n502 = local read "Detector D"() -> (w1708:bool)
                  n503 = local read "X resolution"() -> (w1723:u32)
                  n504 = local read "Y resolution"() -> (w1734:u32)
                  n505 = local read "Oversampling"() -> (w1735:u32)
                  n506 = local read "Scan speed"() -> (w1729:u8)
                  n507 = local read "Frame line rampdown ratio"() -> (w1736:sgl)
                  n508 = local read "X min (V)"() -> (w1664:dbl)
                  n509 = local read "X max (V)"() -> (w1710:dbl)
                  n510 = local read "Det min (V)"() -> (w1666:dbl)
                  n511 = local read "Det max (V)"() -> (w1665:dbl)
                  n512 = local read "Decimating factor"() -> (w1582:u16)
                  n513 = local read "Notes"() -> (w1612:string)
                  n514 = local read "Detector C name"() -> (w1705:string)
                  n515 = local read "Detector D name"() -> (w1706:string)
                  n516 = local read "SEM parameters"() -> (w1608:T5)
                  n517 = local read "FIB parameters"() -> (w1610:T6)
                  n518 = local read "Machine ID"() -> (w1609:string)
                  n519 = local read "Detector B"() -> (w1727:bool)
                  n520 = call-poly <instrlib>:"niScope Get Wfm Coefficients (poly).vi"("instrument handle"=w1603, "channels"="0,1") -> ("coefficient info"=w1605:T21)  [unwired: 11 in, 2 out]
                  n521 = To Single Precision Float(number=w1605) -> (single precision float=w1604:T22)
                  n522 = Bundle("Detector A"=w1728, "Detector B"=w1727, "Detector C"=w1709, "Detector D"=w1708) -> (w1614:T23)  [unwired: 1 out]
                  n523 = Reciprocal(x=w1607) -> (1/x=w1602:dbl)
                  n524 = Bundle("Detector C name"=w1705, "Detector D name"=w1706) -> (w1611:T24)  [unwired: 1 out]
                  n525 = for {
                    tunnel: w1604 -> [w1759] mode=indexing
                    tunnel: [w1758] -> w1574 mode=indexing
                    n526 = Unbundle By Name(w1759) -> ("offset"=w1763:sgl, "gain"=w1762:sgl, "reserved 1"=w1761:sgl, "reserved 2"=w1760:sgl)
                    n527 = Build Array(w1763, w1762, w1761, w1760) -> (w1758:sgl[])
                  }
                  n528 = Bundle("X resolution"=w1723, "Y resolution"=w1734, "Oversampling"=w1735, "Scan speed"=w1729, "AO rate"=w1555, "Frame line rampdown ratio"=w1736, "X min (V)"=w1664, "X max (V)"=w1710, "Det min (V)"=w1666, "Det max (V)"=w1665) -> (w1613:T25)  [unwired: 1 out]
                  n529 = local read "Detector number"() -> (w1719:u8)
                  n530 = Unbundle By Name(w1613) -> ("X resolution"=w1720:u32, "Y resolution"=w1721:u32, "AO rate"=w1722:dbl)
                  n531 = Unbundle By Name(w1608) -> ("Detector A"=w1714:string, "Detector B"=w1713:string, "Brightness A"=w1701:sgl, "Contrast A"=w1700:sgl, "Brightness B"=w1711:sgl, "Contrast B"=w1712:sgl, "Magnification"=w1699:sgl, "Pixel size"=w1698:sgl, "Working distance"=w1697:sgl, "EHT"=w1696:sgl, "Aperture"=w1695:u8, "High current mode"=w1694:u8, "Probe current"=w1693:sgl, "Beam shift X"=w1688:sgl, "Beam shift Y"=w1687:sgl, "Stig X"=w1692:sgl, "Stig Y"=w1691:sgl, "Alignment X"=w1690:sgl, "Alignment Y"=w1689:sgl)
                  n532 = Unbundle By Name("Milling para") -> ("Z-step (nm)"=w1538:dbl)
                  n533 = Select(t=w1561, s=TRUE, f=w1574) -> (s? t:f=w1573:sgl[][])
                  n534 = shared-variable ".\\Zeiss Library.lvlib\\Temp (F)"() -> (w1591:sgl)  [unwired: 1 in, 1 out]
                  n535 = shared-variable ".\\Zeiss Library.lvlib\\Faraday Cup (nA)"() -> (w1590:sgl)  [unwired: 1 in, 1 out]
                  n536 = shared-variable ".\\Zeiss Library.lvlib\\Specimen (nA)"() -> (w1589:sgl)  [unwired: 1 in, 1 out]
                  n537 = shared-variable ".\\Zeiss Library.lvlib\\Beam Dump 1 (nA)"() -> (w1588:sgl)  [unwired: 1 in, 1 out]
                  n538 = shared-variable ".\\Zeiss Library.lvlib\\Beam Dump 2 (nA)"() -> (w1552:sgl)  [unwired: 1 in, 1 out]
                  n539 = shared-variable ".\\Zeiss Library.lvlib\\Milling I (nA)"() -> (w1551:sgl)  [unwired: 1 in, 1 out]
                  n540 = local read "SEM Spec. I (nA)"() -> (w1587:sgl)
                  n541 = shared-variable "My Computer\\Zeiss Library.lvlib\\FIB Slice #"() -> (w1584:u32)  [unwired: 1 in, 1 out]
                  n542 = shared-variable ".\\Zeiss Library.lvlib\\Milling Z Voltage RT"() -> (w1586:sgl)  [unwired: 1 in, 1 out]
                  n543 = local read "X Grids"() -> (w1544:u8)
                  n544 = local read "Y Grids"() -> (w1543:u8)
                  n545 = local read "File name"() -> (w1667:path)
                  n546 = local read "keep aspect ratio"() -> (w1542:bool)
                  n547 = local read "X resolution"() -> (w1663:u32)
                  n548 = local read "Y resolution"() -> (w1662:u32)
                  n549 = Multiply(x=w1544, y=w1543) -> (x*y=w1637:u8)
                  n550 = Less Or Equal?(x=w1637, y=u8 10) -> (x <= y?=w1636:bool)
                  n551 = local read "Notes"() -> (w1718:string)
                  n552 = Open/Create/Replace File(file path (use dialog)=w1667, operation (0:open)=T16."replace or create") -> (refnum out=w1743:refnum<file>, error out=w1742:errorcluster)  [unwired: 1 in, 4 out]
                  n553 = Select(t=u32 1048576 ("Cropped to area pixels"), s=w1636, f=u32 262144 ("Cropped to area pixels")) -> (s? t:f=w1633:u32)
                  n554 = Initialize Array(0.0 ("element"), 128 ("dimension size")) -> (w1739:dbl[])
                  n555 = call "Proportional area crop.vi"("Cropped to area pixels"=w1633, "keep aspect ratio"=w1542, "Y grids"=w1543, "Y resolution"=w1662, "X grids"=w1544, "X resolution"=w1663) -> ("Y length"=w1659:u32, "Y index"=w1661:u32[], "X length"=w1658:u32, "X index"=w1660:u32[])  [unwired: 2 in]
                  n556 = Concatenate Strings(w1716, w1718, w1716) -> (w1717:string)
                  n557 = Write to Binary File(file (use dialog)=w1743, data=w1739, error in=w1742, 5:FALSE ("prepend array or string size? (T)")) -> (refnum out=w1600:refnum<file>, error out=w1599:errorcluster)  [unwired: 3 out]
                  n558 = local read "DetA-Rate"() -> (w1557:sgl)
                  n559 = local read "DetA-Scaling"() -> (w1559:sgl)
                  n560 = local read "DetA-k"() -> (w1556:sgl)
                  n561 = local read "Runsheet header array"() -> (w1578:string[])
                  n562 = local read "File path"() -> (w1581:path)
                  n563 = local read "Timestamp"() -> (w1580:timestamp)
                  n564 = Compound Arithmetic op=MULTIPLY(w1658, w1659, w1544, w1543) -> (w1680:u32)
                  n565 = Initialize Array(i16 0 ("element"), w1680) -> (w1670:i16[])
                  n566 = Initialize Array(i16 0 ("element"), 1 ("dimension size")) -> (w1668:i16[])
                  n567 = Divide(x=w1557, y=w1555) -> (x/y=w1558:dbl)
                  n568 = local read "Detector A"() -> (w1684:bool)
                  n569 = local read "Detector C"() -> (w1683:bool)
                  n570 = local read "Detector D"() -> (w1682:bool)
                  n571 = case shown="0, Default" "FI Detector" {
                    tunnel: [w1776 FALSE ("Detector A") FALSE ("Detector A") FALSE ("Detector A")] -> w1631
                    frame 0, Default {
                      n572 = local read "Detector A"() -> (w1776:bool)
                    }
                    frame 1 {
                    }
                    frame 2 {
                    }
                    frame 3 {
                    }
                  }
                  n573 = case shown="1" "FI Detector" {
                    tunnel: [FALSE ("Detector A") w1773 FALSE ("Detector A") FALSE ("Detector A")] -> w1630
                    frame 0, Default {
                    }
                    frame 1 {
                      n574 = local read "Detector B"() -> (w1773:bool)
                    }
                    frame 2 {
                    }
                    frame 3 {
                    }
                  }
                  n575 = case shown="2" "FI Detector" {
                    tunnel: [FALSE ("Detector A") FALSE ("Detector A") w1770 FALSE ("Detector A")] -> w1628
                    frame 0, Default {
                    }
                    frame 1 {
                    }
                    frame 2 {
                      n576 = local read "Detector C"() -> (w1770:bool)
                    }
                    frame 3 {
                    }
                  }
                  n577 = case shown="3" "FI Detector" {
                    tunnel: [FALSE ("Detector A") FALSE ("Detector A") FALSE ("Detector A") w1767] -> w1629
                    frame 0, Default {
                    }
                    frame 1 {
                    }
                    frame 2 {
                    }
                    frame 3 {
                      n578 = local read "Detector D"() -> (w1767:bool)
                    }
                  }
                  n579 = local read "Detector B"() -> (w1685:bool)
                  n580 = Compound Arithmetic op=MULTIPLY(w1558, w1559, w1556) -> (w1554:dbl)
                  n581 = Set File Position(offset (in bytes) (0)=i64 1024, refnum=w1600, from (0:start)=enum16{"start", "end", "current"}."start", error in=w1599) -> (refnum out=w1746:refnum<file>, error out=w1745:errorcluster)
                  n582 = expression code="1/x**2"(w1554) -> (w1553:dbl)
                  n583 = Build Array(w1684, w1685, w1683, w1682) -> (w1686:bool[])
                  n584 = local read "8-bit"() -> (w1575:bool)
                  n585 = Boolean Array To Number(Boolean array=w1686) -> (number=w1681:u32)
                  n586 = Select(t=w1670, s=w1631, f=w1668) -> (s? t:f=w1674:i16[])
                  n587 = Select(t=w1670, s=w1630, f=w1668) -> (s? t:f=w1673:i16[])
                  n588 = Select(t=w1670, s=w1628, f=w1668) -> (s? t:f=w1672:i16[])
                  n589 = Select(t=w1670, s=w1629, f=w1668) -> (s? t:f=w1671:i16[])
                  n590 = while {
                    tunnel: w1746 -> [w1886]
                    tunnel: [w1884] -> w1598
                    tunnel: w1745 -> [w1883]
                    tunnel: [w1879] -> w1597
                    tunnel: w1704 -> [w1876]
                    tunnel: [w1875] -> w1616
                    tunnel: [w1871] -> w1703
                    tunnel: [w1870] -> w1702
                    tunnel: w1681 -> [w1868]
                    shift-right: [w1864] -> w1678
                    shift-left: w1674 -> [w1866]
                    shift-right: [w1853] -> w1652
                    shift-left: w1673 -> [w1861]
                    shift-right: [w1854] -> w1651
                    shift-left: w1672 -> [w1862]
                    shift-right: [w1855] -> w1648
                    shift-left: w1671 -> [w1863]
                    tunnel: w1661 -> [w1860]
                    tunnel: w1660 -> [w1856]
                    tunnel: w1658 -> [w1851]
                    tunnel: w1659 -> [w1850]
                    tunnel: w1629 -> [w1846]
                    tunnel: w1628 -> [w1847]
                    tunnel: w1630 -> [w1848]
                    tunnel: w1631 -> [w1849]
                    tunnel: [w1851] -> w1645
                    tunnel: [w1850] -> w1644
                    tunnel: [w1849] -> w1627
                    tunnel: [w1848] -> w1626
                    tunnel: [w1847] -> w1625
                    tunnel: [w1846] -> w1624
                    tunnel: w1575 -> [w1844]
                    i -> [w1852]
                    stop <- w1880 stop-if-true
                    n591 = Dequeue Element(queue=w1876) -> (queue out=w1871:refnum<queue>, element=w1843:i16[], error out=w1870:errorcluster)  [unwired: 1 in, 2 out]
                    n592 = local read "Y resolution"() -> (w1867:u32)
                    n593 = Increment(x=w1852) -> (x+1=w1872:i32)
                    n594 = case shown="5" w1868 {
                      tunnel: w1843 -> [w1899 w1900 w1903 w1904 w1907 w1910 w1914 w1915 w1918 w1921 w1925 w1928 w1932 w1933 w1937]
                      tunnel: [w1899 _ w1902 _ w1906 _ w1913 _ w1917 _ w1924 _ w1929 _ w1941] -> w1865
                      tunnel: [_ w1900 w1901 _ _ w1909 w1912 _ _ w1920 w1922 _ _ w1935 w1938] -> w1859
                      tunnel: [_ _ _ w1904 w1905 w1908 w1911 _ _ _ _ w1926 w1930 w1934 w1939] -> w1858
                      tunnel: [_ _ _ _ _ _ _ w1915 w1916 w1919 w1923 w1927 w1931 w1936 w1940] -> w1857
                      frame 1, Default {
                      }
                      frame 2 {
                      }
                      frame 3 {
                        n595 = Decimate 1D Array(w1903) -> (w1902:i16[], w1901:i16[])
                      }
                      frame 4 {
                      }
                      frame 5 {
                        n596 = Decimate 1D Array(w1907) -> (w1906:i16[], w1905:i16[])
                      }
                      frame 6 {
                        n597 = Decimate 1D Array(w1910) -> (w1909:i16[], w1908:i16[])
                      }
                      frame 7 {
                        n598 = Decimate 1D Array(w1914) -> (w1913:i16[], w1912:i16[], w1911:i16[])
                      }
                      frame 8 {
                      }
                      frame 9 {
                        n599 = Decimate 1D Array(w1918) -> (w1917:i16[], w1916:i16[])
                      }
                      frame 10 {
                        n600 = Decimate 1D Array(w1921) -> (w1920:i16[], w1919:i16[])
                      }
                      frame 11 {
                        n601 = Decimate 1D Array(w1925) -> (w1924:i16[], w1922:i16[], w1923:i16[])
                      }
                      frame 12 {
                        n602 = Decimate 1D Array(w1928) -> (w1926:i16[], w1927:i16[])
                      }
                      frame 13 {
                        n603 = Decimate 1D Array(w1932) -> (w1929:i16[], w1930:i16[], w1931:i16[])
                      }
                      frame 14 {
                        n604 = Decimate 1D Array(w1933) -> (w1935:i16[], w1934:i16[], w1936:i16[])
                      }
                      frame 15 {
                        n605 = Decimate 1D Array(w1937) -> (w1941:i16[], w1938:i16[], w1939:i16[], w1940:i16[])
                      }
                    }
                    n606 = In Range and Coerce(upper limit=u8 255 ("offset (in bytes) (0)"), x=w1843, lower limit=u8 0 ("offset (in bytes) (0)")) -> (coerced(x)=w1842:i16[])  [unwired: 1 out]
                    n607 = Less Or Equal?(x=w1867, y=w1872) -> (x <= y?=w1873:bool)
                    n608 = To Unsigned Byte Integer(number=w1842) -> (unsigned 8bit integer=w1845:u8[])
                    n609 = local read "Save"() -> (w1878:bool)
                    n610 = case shown="True" w1844 {
                      tunnel: w1886 -> [w1891 w1897]
                      tunnel: [w1890 w1896] -> w1885
                      tunnel: w1883 -> [w1889 w1895]
                      tunnel: [w1888 w1894] -> w1882
                      tunnel: w1845 -> [_ w1893]
                      tunnel: w1843 -> [w1887 _]
                      frame False {
                        n611 = Write to Binary File(file (use dialog)=w1891, data=w1887, error in=w1889, 5:FALSE ("prepend array or string size? (T)")) -> (refnum out=w1890:refnum<file>, error out=w1888:errorcluster)  [unwired: 3 out]
                      }
                      frame True {
                        n612 = Write to Binary File(file (use dialog)=w1897, data=w1893, error in=w1895, 5:FALSE ("prepend array or string size? (T)")) -> (refnum out=w1896:refnum<file>, error out=w1894:errorcluster)  [unwired: 3 out]
                      }
                    }
                    n613 = call "Scan line to grid area.vi"("Y index"=w1860, "X index"=w1856, "Y length"=w1850, "X length"=w1851, "Y scan line"=w1852, "Enable"=w1849, "Single line scan"=w1865, "Input array"=w1866) -> ("Ouput array"=w1864:i16[])  [unwired: 3 in]
                    n614 = call "Scan line to grid area.vi"("Y index"=w1860, "X index"=w1856, "Y length"=w1850, "X length"=w1851, "Y scan line"=w1852, "Enable"=w1848, "Single line scan"=w1859, "Input array"=w1861) -> ("Ouput array"=w1853:i16[])  [unwired: 3 in]
                    n615 = call "Scan line to grid area.vi"("Y index"=w1860, "X index"=w1856, "Y length"=w1850, "X length"=w1851, "Y scan line"=w1852, "Enable"=w1847, "Single line scan"=w1858, "Input array"=w1862) -> ("Ouput array"=w1854:i16[])  [unwired: 3 in]
                    n616 = call "Scan line to grid area.vi"("Y index"=w1860, "X index"=w1856, "Y length"=w1850, "X length"=w1851, "Y scan line"=w1852, "Enable"=w1846, "Single line scan"=w1857, "Input array"=w1863) -> ("Ouput array"=w1855:i16[])  [unwired: 3 in]
                    n617 = local read "stop"() -> (w1869:bool)
                    n618 = Unbundle By Name(w1870) -> ("status"=w1874:bool)
                    n619 = Not(x=w1878) -> (.not. x?=w1877:bool)
                    n620 = Get File Position(4:w1882, 7:w1885) -> (0:w1879:errorcluster, 2:w1875:i64, 3:w1884:refnum<file>)
                    n621 = Unbundle By Name(w1879) -> ("status"=w1881:bool)
                    n622 = Compound Arithmetic op=OR(w1881, w1874, w1877, w1873, w1869) -> (w1880:bool)
                  }
                  n623 = local read "X Grids"() -> (w1647:u8)
                  n624 = local read "Y Grids"() -> (w1646:u8)
                  n625 = local read "Pixel size (nm)"() -> (w1550:sgl)
                  n626 = local read "Primary X index"() -> (w1541:u8)
                  n627 = local read "Primary Y index"() -> (w1540:u8)
                  n628 = shared-variable ".\\Zeiss Library.lvlib\\Recipe input"() -> (w1615:variant)  [unwired: 1 in, 1 out]
                  n629 = Less?(x=w1550, y=sgl 4.0) -> (x < y?=w1548:bool)
                  n630 = In Range and Coerce(upper limit=w1647, x=w1541, lower limit=w1653) -> (coerced(x)=w1650:u8)  [unwired: 1 out]
                  n631 = In Range and Coerce(upper limit=w1646, x=w1540, lower limit=w1653) -> (coerced(x)=w1649:u8)  [unwired: 1 out]
                  n632 = Select(t=TRUE ("prepend array or string size? (T)"), s=w1548, f=FALSE ("prepend array or string size? (T)")) -> (s? t:f=w1545:bool)
                  n633 = case shown="True" w1627 {
                    tunnel: w1678 -> [_ w1839]
                    tunnel: w1645 -> [_ w1838]
                    tunnel: w1644 -> [_ w1837]
                    tunnel: w1647 -> [_ w1836]
                    tunnel: w1646 -> [_ w1835]
                    tunnel: [w1824 w1832] -> w1656
                    tunnel: w1650 -> [_ w1831]
                    tunnel: w1649 -> [_ w1830]
                    tunnel: [sgl[][] [] ("Focus index array") w1829] -> w1654
                    tunnel: [w1824 w1828] -> w1566
                    tunnel: [w1824 w1827] -> w1565
                    tunnel: w1545 -> [_ w1826]
                    frame False {
                      w1824 = sgl 0.0 ("Focus index")
                    }
                    frame True {
                      n634 = call "Focus Index by Grid.vi"("Input array"=w1839, "Primary X index"=w1831, "X grids"=w1836, "Pre-bin 2"=w1826, "Y grids"=w1835, "X length"=w1838, "Y length"=w1837, "Primary Y index"=w1830) -> ("Focus index array"=w1829:sgl[][], "Primary FI"=w1832:sgl, "Primary eval area mean"=w1828:sgl, "Primary eval area std"=w1827:sgl, "Primary eval area"=w1834:dbl[][])  [unwired: 3 in]
                      n635 = To Word Integer(number=w1834) -> (16bit integer=→"Eval A":i16[][])
                    }
                  }
                  n636 = case shown="True" w1626 {
                    tunnel: w1652 -> [_ w1823]
                    tunnel: w1645 -> [_ w1822]
                    tunnel: w1644 -> [_ w1821]
                    tunnel: w1647 -> [_ w1820]
                    tunnel: w1646 -> [_ w1819]
                    tunnel: [w1808 w1817] -> w1643
                    tunnel: w1650 -> [_ w1816]
                    tunnel: w1649 -> [_ w1815]
                    tunnel: [sgl[][] [] ("Focus index array") w1814] -> w1640
                    tunnel: [w1808 w1812] -> w1564
                    tunnel: [w1808 w1811] -> w1563
                    tunnel: w1545 -> [_ w1810]
                    frame False {
                      w1808 = sgl 0.0 ("Focus index")
                    }
                    frame True {
                      n637 = call "Focus Index by Grid.vi"("Input array"=w1823, "Primary X index"=w1816, "X grids"=w1820, "Pre-bin 2"=w1810, "Y grids"=w1819, "X length"=w1822, "Y length"=w1821, "Primary Y index"=w1815) -> ("Focus index array"=w1814:sgl[][], "Primary FI"=w1817:sgl, "Primary eval area mean"=w1812:sgl, "Primary eval area std"=w1811:sgl, "Primary eval area"=w1818:dbl[][])  [unwired: 3 in]
                      n638 = To Word Integer(number=w1818) -> (16bit integer=→"Eval B":i16[][])
                    }
                  }
                  n639 = case shown="True" w1625 {
                    tunnel: w1651 -> [_ w1807]
                    tunnel: w1645 -> [_ w1806]
                    tunnel: w1644 -> [_ w1805]
                    tunnel: w1647 -> [_ w1804]
                    tunnel: w1646 -> [_ w1803]
                    tunnel: [sgl 0.0 ("Focus index") w1801] -> w1642
                    tunnel: w1650 -> [_ w1800]
                    tunnel: w1649 -> [_ w1799]
                    tunnel: [sgl[][] [] ("Focus index array") w1798] -> w1639
                    tunnel: w1545 -> [_ w1796]
                    frame False {
                    }
                    frame True {
                      n640 = call "Focus Index by Grid.vi"("Input array"=w1807, "Primary X index"=w1800, "X grids"=w1804, "Pre-bin 2"=w1796, "Y grids"=w1803, "X length"=w1806, "Y length"=w1805, "Primary Y index"=w1799) -> ("Focus index array"=w1798:sgl[][], "Primary FI"=w1801:sgl, "Primary eval area"=w1802:dbl[][])  [unwired: 3 in, 2 out]
                      n641 = To Word Integer(number=w1802) -> (16bit integer=→"Eval C":i16[][])
                    }
                  }
                  n642 = case shown="True" w1624 {
                    tunnel: w1648 -> [_ w1793]
                    tunnel: w1645 -> [_ w1792]
                    tunnel: w1644 -> [_ w1791]
                    tunnel: w1647 -> [_ w1790]
                    tunnel: w1646 -> [_ w1789]
                    tunnel: [sgl 0.0 ("Focus index") w1787] -> w1641
                    tunnel: w1650 -> [_ w1786]
                    tunnel: w1649 -> [_ w1785]
                    tunnel: [sgl[][] [] ("Focus index array") w1784] -> w1638
                    tunnel: w1545 -> [_ w1782]
                    frame False {
                    }
                    frame True {
                      n643 = call "Focus Index by Grid.vi"("Input array"=w1793, "Primary X index"=w1786, "X grids"=w1790, "Pre-bin 2"=w1782, "Y grids"=w1789, "X length"=w1792, "Y length"=w1791, "Primary Y index"=w1785) -> ("Focus index array"=w1784:sgl[][], "Primary FI"=w1787:sgl, "Primary eval area"=w1788:dbl[][])  [unwired: 3 in, 2 out]
                      n644 = To Word Integer(number=w1788) -> (16bit integer=→"Eval D":i16[][])
                    }
                  }
                  n645 = local read "8-bit"() -> (w1571:bool)
                  n646 = local read "FI scaling"() -> (w1569:u8)
                  n647 = local read "Image Focus Index Array"() -> (w1655:T3)
                  n648 = Select(t=w1553, s=w1571, f=1.0) -> (s? t:f=w1570:dbl)
                  n649 = Multiply(x=w1569, y=w1570) -> (x*y=w1568:dbl)
                  n650 = Bundle(cluster=w1655, "A Img Focus Index array"=w1654, "B Img Focus Index array"=w1640, "C Img Focus Index array"=w1639, "D Img Focus Index array"=w1638) -> (w1623:T3)
                  n651 = local read "Image Focus Index"() -> (w1677:T4)
                  n652 = Multiply(x=w1623, y=w1568) -> (x*y=w1577:T26)
                  "Image Focus Index Array" <- w1577
                  n653 = Bundle(cluster=w1677, "A Img Focus Index"=w1656, "B Img Focus Index"=w1643, "C Img Focus Index"=w1642, "D Img Focus Index"=w1641) -> (w1622:T4)
                  n654 = To Variant(anything=w1577) -> (Variant=w1576:variant)
                  n655 = Multiply(x=w1568, y=w1622) -> (x*y=w1592:T27)
                  "Image Focus Index" <- w1592
                  n656 = Unbundle By Name(w1592) -> ("A Img Focus Index"=w1676:dbl, "B Img Focus Index"=w1675:dbl)
                  n657 = case shown="0, Default" "FI Detector" {
                    tunnel: w1592 -> [w1751 w1753 w1755 w1757]
                    tunnel: [w1750 w1752 w1754 w1756] -> w1585
                    frame 0, Default {
                      n658 = Unbundle By Name(w1751) -> ("A Img Focus Index"=w1750:dbl)
                    }
                    frame 1 {
                      n659 = Unbundle By Name(w1753) -> ("B Img Focus Index"=w1752:dbl)
                    }
                    frame 2 {
                      n660 = Unbundle By Name(w1755) -> ("C Img Focus Index"=w1754:dbl)
                    }
                    frame 3 {
                      n661 = Unbundle By Name(w1757) -> ("D Img Focus Index"=w1756:dbl)
                    }
                  }
                  n662 = Build Array(w1719, w1720, w1721, w1722, w1701, w1700, w1711, w1712, w1699, w1698, w1697, w1696, w1695, w1694, w1693, w1688, w1687, w1692, w1691, w1690, w1689, w1538, w1676, w1675, w1566, w1565, w1564, w1563) -> (w1724:dbl[])
                  n663 = Bundle("Single"=w1591, "Single"=w1590, "Single"=w1589, "Single"=w1588, "Single"=w1552, "Single"=w1551, "SEM Spec. I (nA)"=w1587, "Single"=w1586, "D Img Focus Index"=w1585, "UInt32"=w1584) -> (w1583:T28)  [unwired: 1 out]
                  n664 = Bundle(w1602, "8-bit"=w1572, "8-bit coefficents"=w1573, w1614, w1613, "Decimating factor"=w1582, "Notes"=w1612, w1611, "SEM parameters"=w1608, "FIB parameters"=w1610, "Milling para"="Milling para", "Machine ID"=w1609, w1583) -> (w1601:T29)  [unwired: 1 in]
                  n665 = Array To Spreadsheet String(delimiter (Tab)=",", array=w1724, 3:"%#g" ("format string")) -> (spreadsheet string=w1715:string)
                  n666 = Scan String For Tokens(9:w1715) -> (1:w1707:string)  [unwired: 1 in, 7 out]
                  n667 = Build Array(w1717, w1714, w1713, w1705, w1706, w1707) -> (w1579:string[])
                  n668 = call "YMD log files.vi"("Input text array"=w1579, "Input header array"=w1578, "current time"=w1580, "Log file path"=w1581) -> ()  [unwired: 8 in]
                  n669 = call "Zeiss File Header Tclk.vi"("error in"=w1597, "Inputs"=w1601, "refnum"=w1598) -> ("error out"=w1593:errorcluster, "dup refnum"=w1594:refnum<file>)  [unwired: 6 in, 1 out]
                  n670 = Set File Position(offset (in bytes) (0)=i64 1000, refnum=w1594, error in=w1593) -> (refnum out=w1733:refnum<file>, error out=w1732:errorcluster)  [unwired: 1 in]
                  n671 = Write to Binary File(file (use dialog)=w1733, data=w1616, error in=w1732, 5:FALSE ("prepend array or string size? (T)")) -> (refnum out=w1618:refnum<file>, error out=w1617:errorcluster)  [unwired: 3 out]
                  n672 = Set File Position(offset (in bytes) (0)=w1616, refnum=w1618, error in=w1617) -> (refnum out=w1619:refnum<file>, error out=w1620:errorcluster)  [unwired: 1 in]
                  n673 = Write to Binary File(file (use dialog)=w1619, data=w1615, error in=w1620, 5:FALSE ("prepend array or string size? (T)")) -> (refnum out=w1596:refnum<file>, error out=w1595:errorcluster)  [unwired: 3 out]
                  n674 = Close File(refnum=w1596, error in=w1595) -> (error out=w1738:errorcluster)  [unwired: 1 out]
                  n675 = shared-variable ".\\Zeiss Library.lvlib\\Focus Index Array"(w1576) -> ()  [unwired: 1 in, 1 out]
                  n676 = call <vilib>:"General Error Handler.vi"("type of dialog (OK msg:1)"=w1737, "error in (no error)"=w1738) -> ()  [unwired: 1 in, 13 out]
                }
                frame True {
                  n677 = Wait on Occurrence(2:w1942) -> ()  [unwired: 2 in, 1 out]
                }
              }
            }
            frame #3 {
              n678 = local read "Display"() -> (w1944:bool)
              n679 = case shown="True" w1944 {
                tunnel: w1943 -> [_ w1954]
                frame False {
                }
                frame True {
                  w2010 = "%s, Max/Mean/Min = %#g / %#g / %#g, Focus INdex = %^_3e" ("format string")
                  w2041 = "%s, B&C = %#u\\% & %#u\\%, Max/Mean/Min = %#g / %#g / %#g, Focus Index = %^_3e" ("format string")
                  n680 = local read "Detector A"() -> (w2035:bool)
                  n681 = local read "Detector C"() -> (w2033:bool)
                  n682 = local read "Detector D"() -> (w2032:bool)
                  n683 = local read "Detector B"() -> (w2034:bool)
                  n684 = local read "Det B Img"() -> (w1982:i16[][])
                  n685 = local read "Detector A"() -> (w1979:bool)
                  n686 = local read "Detector C"() -> (w1978:bool)
                  n687 = local read "Detector D"() -> (w1975:bool)
                  n688 = local read "Det A Img"() -> (w1981:i16[][])
                  n689 = local read "Det C Img"() -> (w1983:i16[][])
                  n690 = local read "Det D Img"() -> (w1984:i16[][])
                  n691 = local read "Detector B"() -> (w1976:bool)
                  n692 = case shown="True" w2035 {
                    tunnel: [u8[][] [] w2188] -> w1985
                    tunnel: [_ w2191] -> w1950
                    tunnel: [_ w2190] -> w1949
                    tunnel: [_ w2189] -> w1948
                    tunnel: [_ w2193] -> w1998
                    frame False {
                    }
                    frame True {
                      n693 = local read "Det A Img"() -> (w2192:i16[][])
                      n694 = local read "Image Focus Index"() -> (w2194:T4)
                      n695 = call "16bit Image Normalization.vi"("Input image"=w2192) -> ("min"=w2189:i16, "mean"=w2190:i16, "max"=w2191:i16, "Normalized image"=w2188:u8[][])  [unwired: 6 in, 1 out]
                      n696 = Unbundle By Name(w2194) -> ("A Img Focus Index"=w2193:sgl)
                    }
                  }
                  n697 = case shown="True" w2034 {
                    tunnel: [u8[][] [] w2184] -> w2019
                    tunnel: [_ w2183] -> w1947
                    tunnel: [_ w2182] -> w1946
                    tunnel: [_ w2181] -> w1945
                    tunnel: [_ w2185] -> w1999
                    frame False {
                    }
                    frame True {
                      n698 = local read "Det B Img"() -> (w2180:i16[][])
                      n699 = local read "Image Focus Index"() -> (w2186:T4)
                      n700 = call "16bit Image Normalization.vi"("Input image"=w2180) -> ("min"=w2181:i16, "mean"=w2182:i16, "max"=w2183:i16, "Normalized image"=w2184:u8[][])  [unwired: 6 in, 1 out]
                      n701 = Unbundle By Name(w2186) -> ("B Img Focus Index"=w2185:sgl)
                    }
                  }
                  n702 = case shown="True" w2033 {
                    tunnel: [u8[][] [] w2171] -> w2018
                    tunnel: [_ w2173] -> w2014
                    tunnel: [_ w2174] -> w2015
                    tunnel: [_ w2172] -> w2013
                    tunnel: [_ w2175] -> w1997
                    frame False {
                    }
                    frame True {
                      n703 = local read "Det C Img"() -> (w2170:i16[][])
                      n704 = local read "Image Focus Index"() -> (w2176:T4)
                      n705 = call "16bit Image Normalization.vi"("Input image"=w2170) -> ("min"=w2172:i16, "mean"=w2173:i16, "max"=w2174:i16, "Normalized image"=w2171:u8[][])  [unwired: 6 in, 1 out]
                      n706 = Unbundle By Name(w2176) -> ("C Img Focus Index"=w2175:sgl)
                    }
                  }
                  n707 = case shown="True" w2032 {
                    tunnel: [u8[][] [] w2163] -> w2017
                    tunnel: [_ w2166] -> w2009
                    tunnel: [_ w2165] -> w2008
                    tunnel: [_ w2164] -> w2007
                    tunnel: [_ w2167] -> w1996
                    frame False {
                    }
                    frame True {
                      n708 = local read "Det D Img"() -> (w2162:i16[][])
                      n709 = local read "Image Focus Index"() -> (w2168:T4)
                      n710 = call "16bit Image Normalization.vi"("Input image"=w2162) -> ("min"=w2164:i16, "mean"=w2165:i16, "max"=w2166:i16, "Normalized image"=w2163:u8[][])  [unwired: 6 in, 1 out]
                      n711 = Unbundle By Name(w2168) -> ("D Img Focus Index"=w2167:sgl)
                    }
                  }
                  n712 = Build Array(w2035, w2034, w2033, w2032) -> (w2031:bool[])
                  n713 = Build Array(w1979, w1976, w1978, w1975) -> (w1977:bool[])
                  n714 = Boolean Array To Number(Boolean array=w2031) -> (number=w2044:u32)
                  n715 = Boolean Array To Number(Boolean array=w1977) -> (number=w1980:u32)
                  n716 = case shown="2" w1980 {
                    tunnel: w1981 -> [w2091 _ w2093 _ w2095 _ w2097 _ w2099 _ w2101 _ w2103 _ w2105]
                    tunnel: w1982 -> [_ w2092 _ _ _ w2096 _ _ _ w2100 _ _ _ w2104 _]
                    tunnel: [w2091 w2092 w2093 w2094 w2095 w2096 w2097 w2098 w2099 w2100 w2101 w2102 w2103 w2104 w2105] -> w1974
                    tunnel: w1983 -> [_ _ _ w2094 _ _ _ _ _ _ _ w2102 _ _ _]
                    tunnel: w1984 -> [_ _ _ _ _ _ _ w2098 _ _ _ _ _ _ _]
                    frame 1, Default {
                    }
                    frame 2 {
                    }
                    frame 3 {
                    }
                    frame 4 {
                    }
                    frame 5 {
                    }
                    frame 6 {
                    }
                    frame 7 {
                    }
                    frame 8 {
                    }
                    frame 9 {
                    }
                    frame 10 {
                    }
                    frame 11 {
                    }
                    frame 12 {
                    }
                    frame 13 {
                    }
                    frame 14 {
                    }
                    frame 15 {
                    }
                  }
                  n717 = local read "Image bits"() -> (w1972:u8)
                  n718 = local read "Inverse PNG"() -> (w1971:bool)
                  n719 = case shown="True" w1971 {
                    tunnel: [u32[] [16777222, 65793, 131586, 197379, 263172, 328965, 394758, 460551, 526344, 592137, 657930, 723723, 789516, 855309, 921102, 986895, 1052688, 1118481, 1184274, 1250067, 1315860, 1381653, 1447446, 1513239, 1579032, 1644825, 1710618, 1776411, 1842204, 1907997, 1973790, 2039583, 2105376, 2171169, 2236962, 2302755, 2368548, 2434341, 2500134, 2565927, 2631720, 2697513, 2763306, 2829099, 2894892, 2960685, 3026478, 3092271, 3158064, 3223857, 3289650, 3355443, 3421236, 3487029, 3552822, 3618615, 3684408, 3750201, 3815994, 3881787, 3947580, 4013373, 4079166, 4144959, 4210752, 4276545, 4342338, 4408131, 4473924, 4539717, 4605510, 4671303, 4737096, 4802889, 4868682, 4934475, 5000268, 5066061, 5131854, 5197647, 5263440, 5329233, 5395026, 5460819, 5526612, 5592405, 5658198, 5723991, 5789784, 5855577, 5921370, 5987163, 6052956, 6118749, 6184542, 6250335, 6316128, 6381921, 6447714, 6513507, 6579300, 6645093, 6710886, 6776679, 6842472, 6908265, 6974058, 7039851, 7105644, 7171437, 7237230, 7303023, 7368816, 7434609, 7500402, 7566195, 7631988, 7697781, 7763574, 7829367, 7895160, 7960953, 8026746, 8092539, 8158332, 8224125, 8289918, 8355711, 8421504, 8487297, 8553090, 8618883, 8684676, 8750469, 8816262, 8882055, 8947848, 9013641, 9079434, 9145227, 9211020, 9276813, 9342606, 9408399, 9474192, 9539985, 9605778, 9671571, 9737364, 9803157, 9868950, 9934743, 10000536, 10066329, 10132122, 10197915, 10263708, 10329501, 10395294, 10461087, 10526880, 10592673, 10658466, 10724259, 10790052, 10855845, 10921638, 10987431, 11053224, 11119017, 11184810, 11250603, 11316396, 11382189, 11447982, 11513775, 11579568, 11645361, 11711154, 11776947, 11842740, 11908533, 11974326, 12040119, 12105912, 12171705, 12237498, 12303291, 12369084, 12434877, 12500670, 12566463, 12632256, 12698049, 12763842, 12829635, 12895428, 12961221, 13027014, 13092807, 13158600, 13224393, 13290186, 13355979, 13421772, 13487565, 13553358, 13619151, 13684944, 13750737, 13816530, 13882323, 13948116, 14013909, 14079702, 14145495, 14211288, 14277081, 14342874, 14408667, 14474460, 14540253, 14606046, 14671839, 14737632, 14803425, 14869218, 14935011, 15000804, 15066597, 15132390, 15198183, 15263976, 15329769, 15395562, 15461355, 15527148, 15592941, 15658734, 15724527, 15790320, 15856113, 15921906, 15987699, 16053492, 16119285, 16185078, 16250871, 16316664, 16382457, 16448250, 16514043, 16579836, 16645629, 16711422, 16448250] ("256 gray scale") u32[] [16448250, 16711422, 16645629, 16579836, 16514043, 16448250, 16382457, 16316664, 16250871, 16185078, 16119285, 16053492, 15987699, 15921906, 15856113, 15790320, 15724527, 15658734, 15592941, 15527148, 15461355, 15395562, 15329769, 15263976, 15198183, 15132390, 15066597, 15000804, 14935011, 14869218, 14803425, 14737632, 14671839, 14606046, 14540253, 14474460, 14408667, 14342874, 14277081, 14211288, 14145495, 14079702, 14013909, 13948116, 13882323, 13816530, 13750737, 13684944, 13619151, 13553358, 13487565, 13421772, 13355979, 13290186, 13224393, 13158600, 13092807, 13027014, 12961221, 12895428, 12829635, 12763842, 12698049, 12632256, 12566463, 12500670, 12434877, 12369084, 12303291, 12237498, 12171705, 12105912, 12040119, 11974326, 11908533, 11842740, 11776947, 11711154, 11645361, 11579568, 11513775, 11447982, 11382189, 11316396, 11250603, 11184810, 11119017, 11053224, 10987431, 10921638, 10855845, 10790052, 10724259, 10658466, 10592673, 10526880, 10461087, 10395294, 10329501, 10263708, 10197915, 10132122, 10066329, 10000536, 9934743, 9868950, 9803157, 9737364, 9671571, 9605778, 9539985, 9474192, 9408399, 9342606, 9276813, 9211020, 9145227, 9079434, 9013641, 8947848, 8882055, 8816262, 8750469, 8684676, 8618883, 8553090, 8487297, 8421504, 8355711, 8289918, 8224125, 8158332, 8092539, 8026746, 7960953, 7895160, 7829367, 7763574, 7697781, 7631988, 7566195, 7500402, 7434609, 7368816, 7303023, 7237230, 7171437, 7105644, 7039851, 6974058, 6908265, 6842472, 6776679, 6710886, 6645093, 6579300, 6513507, 6447714, 6381921, 6316128, 6250335, 6184542, 6118749, 6052956, 5987163, 5921370, 5855577, 5789784, 5723991, 5658198, 5592405, 5526612, 5460819, 5395026, 5329233, 5263440, 5197647, 5131854, 5066061, 5000268, 4934475, 4868682, 4802889, 4737096, 4671303, 4605510, 4539717, 4473924, 4408131, 4342338, 4276545, 4210752, 4144959, 4079166, 4013373, 3947580, 3881787, 3815994, 3750201, 3684408, 3618615, 3552822, 3487029, 3421236, 3355443, 3289650, 3223857, 3158064, 3092271, 3026478, 2960685, 2894892, 2829099, 2763306, 2697513, 2631720, 2565927, 2500134, 2434341, 2368548, 2302755, 2236962, 2171169, 2105376, 2039583, 1973790, 1907997, 1842204, 1776411, 1710618, 1644825, 1579032, 1513239, 1447446, 1381653, 1315860, 1250067, 1184274, 1118481, 1052688, 986895, 921102, 855309, 789516, 723723, 657930, 592137, 526344, 460551, 394758, 328965, 263172, 197379, 131586, 65793, 16777222] ("256 gray scale inverse")] -> w1970
                    frame False {
                    }
                    frame True {
                    }
                  }
                  n720 = call "16bit Image Normalization.vi"("Transpose"=FALSE, "Imput image bits"=w1972, "Input image"=w1974) -> ("Direct scaled image"=w1960:u8[][])  [unwired: 4 in, 4 out]
                  n721 = local read "PNG only"() -> (w1968:bool)
                  n722 = local read "Inverse PNG"() -> (w2052:bool)
                  n723 = call <vilib>:"Flatten Pixmap.vi"("colors"=w1970, "8-bit pixmap"=w1960) -> ("image data"=w1969:T30)  [unwired: 4 in, 5 out]
                  n724 = Build Array (concatenate)(w1985, w2019, w2018, w2017) -> (w1995:u8[][])
                  n725 = shared-variable "My Computer\\Zeiss Library.lvlib\\DetB Max"(w1947) -> ()  [unwired: 1 in, 1 out]
                  n726 = shared-variable "My Computer\\Zeiss Library.lvlib\\DetB Mean"(w1946) -> ()  [unwired: 1 in, 1 out]
                  n727 = shared-variable "My Computer\\Zeiss Library.lvlib\\DetB Min"(w1945) -> ()  [unwired: 1 in, 1 out]
                  n728 = case shown="False" w1968 {
                    tunnel: w1969 -> [w2088 _]
                    frame False {
                      n729 = local read "Tile index"() -> (w2085:u8[])
                      n730 = Index Array(array=w2085) -> (element #1=w2086:u8, element #2=w2087:u8)  [unwired: 2 in]
                      n731 = Format Into String(w2086) -> (resulting string=w2084:string)  [unwired: 3 in, 1 out]
                      n732 = Format Into String(w2087) -> (resulting string=w2082:string)  [unwired: 3 in, 1 out]
                      n733 = Concatenate Strings("Low res_" ("string"), w2084, "-" ("string"), w2082, ".png" ("string")) -> (w2078:string)
                      n734 = Build Path(base path=path "D:/3D FIB-SEM Files" ("path to PNG file"), name or relative path=w2078) -> (appended path=w2077:path)
                      n735 = call <vilib>:"Write PNG File.vi"("image data"=w2088, "path to PNG file"=w2077) -> ()  [unwired: 1 in, 9 out]
                    }
                    frame True {
                    }
                  }
                  n736 = local read "Detector C name"() -> (w2006:string)
                  n737 = local read "Detector D name"() -> (w2011:string)
                  n738 = Transpose 2D Array(2D array=w1995) -> (transposed array=w2065:u8[][])
                  n739 = local read "FI Detector"() -> (w1953:u16)
                  n740 = local read "Eval A"() -> (w1991:i16[][])
                  n741 = local read "Eval B"() -> (w1992:i16[][])
                  n742 = local read "Eval C"() -> (w1993:i16[][])
                  n743 = local read "Eval D"() -> (w1994:i16[][])
                  n744 = shared-variable "My Computer\\Zeiss Library.lvlib\\DetA Max"(w1950) -> ()  [unwired: 1 in, 1 out]
                  n745 = case shown="False" w2052 {
                    tunnel: [u8 0 ("element") u8 255 ("element")] -> w2069
                    frame False {
                    }
                    frame True {
                    }
                  }
                  n746 = shared-variable "My Computer\\Zeiss Library.lvlib\\DetA Mean"(w1949) -> ()  [unwired: 1 in, 1 out]
                  n747 = shared-variable "My Computer\\Zeiss Library.lvlib\\DetA Min"(w1948) -> ()  [unwired: 1 in, 1 out]
                  n748 = local read "SEM parameters"() -> (w2036:T5)
                  n749 = Unbundle By Name(w2036) -> ("Detector A"=w2040:string, "Brightness A"=w2001:sgl, "Contrast A"=w2000:sgl, "Detector B"=w2037:string, "Brightness B"=w2038:sgl, "Contrast B"=w2039:sgl)
                  n750 = local read "Image bits"() -> (w1986:u8)
                  n751 = case shown="0, Default" w1953 {
                    tunnel: w1991 -> [w2125 _ _ _]
                    tunnel: w1992 -> [_ w2126 _ _]
                    tunnel: [w2125 w2126 w2127 w2128] -> w1956
                    tunnel: w1993 -> [_ _ w2127 _]
                    tunnel: w1994 -> [_ _ _ w2128]
                    frame 0, Default {
                    }
                    frame 1 {
                    }
                    frame 2 {
                    }
                    frame 3 {
                    }
                  }
                  n752 = Array Size(array=w1956) -> (size(s)=w2068:i32[])
                  n753 = Index Array(array=w2068, index=1) -> (element=w1990:i32)
                  n754 = Initialize Array(w2069, 60 ("dimension size"), w1990) -> (w2066:u8[][])
                  n755 = local read "Inverse PNG"() -> (w1964:bool)
                  n756 = local read "PNG only"() -> (w1988:bool)
                  n757 = Format Into String(format string=w2041, w2040, w2001, w2000, w1950, w1949, w1948, w1998) -> (resulting string=w2043:string)  [unwired: 2 in, 1 out]
                  n758 = Format Into String(format string=w2041, w2037, w2038, w2039, w1947, w1946, w1945, w1999) -> (resulting string=w2042:string)  [unwired: 2 in, 1 out]
                  n759 = Format Into String(format string=w2010, w2006, w2015, w2014, w2013, w1997) -> (resulting string=w2016:string)  [unwired: 2 in, 1 out]
                  n760 = Format Into String(format string=w2010, w2011, w2009, w2008, w2007, w1996) -> (resulting string=w2012:string)  [unwired: 2 in, 1 out]
                  n761 = call "16bit Image Normalization.vi"("Transpose"=FALSE, "Imput image bits"=w1986, "Input image"=w1956) -> ("Normalized image"=w1957:u8[][], "Direct scaled image"=w1955:u8[][])  [unwired: 4 in, 3 out]
                  n762 = case shown="True" w1964 {
                    tunnel: [u32[] [16777222, 65793, 131586, 197379, 263172, 328965, 394758, 460551, 526344, 592137, 657930, 723723, 789516, 855309, 921102, 986895, 1052688, 1118481, 1184274, 1250067, 1315860, 1381653, 1447446, 1513239, 1579032, 1644825, 1710618, 1776411, 1842204, 1907997, 1973790, 2039583, 2105376, 2171169, 2236962, 2302755, 2368548, 2434341, 2500134, 2565927, 2631720, 2697513, 2763306, 2829099, 2894892, 2960685, 3026478, 3092271, 3158064, 3223857, 3289650, 3355443, 3421236, 3487029, 3552822, 3618615, 3684408, 3750201, 3815994, 3881787, 3947580, 4013373, 4079166, 4144959, 4210752, 4276545, 4342338, 4408131, 4473924, 4539717, 4605510, 4671303, 4737096, 4802889, 4868682, 4934475, 5000268, 5066061, 5131854, 5197647, 5263440, 5329233, 5395026, 5460819, 5526612, 5592405, 5658198, 5723991, 5789784, 5855577, 5921370, 5987163, 6052956, 6118749, 6184542, 6250335, 6316128, 6381921, 6447714, 6513507, 6579300, 6645093, 6710886, 6776679, 6842472, 6908265, 6974058, 7039851, 7105644, 7171437, 7237230, 7303023, 7368816, 7434609, 7500402, 7566195, 7631988, 7697781, 7763574, 7829367, 7895160, 7960953, 8026746, 8092539, 8158332, 8224125, 8289918, 8355711, 8421504, 8487297, 8553090, 8618883, 8684676, 8750469, 8816262, 8882055, 8947848, 9013641, 9079434, 9145227, 9211020, 9276813, 9342606, 9408399, 9474192, 9539985, 9605778, 9671571, 9737364, 9803157, 9868950, 9934743, 10000536, 10066329, 10132122, 10197915, 10263708, 10329501, 10395294, 10461087, 10526880, 10592673, 10658466, 10724259, 10790052, 10855845, 10921638, 10987431, 11053224, 11119017, 11184810, 11250603, 11316396, 11382189, 11447982, 11513775, 11579568, 11645361, 11711154, 11776947, 11842740, 11908533, 11974326, 12040119, 12105912, 12171705, 12237498, 12303291, 12369084, 12434877, 12500670, 12566463, 12632256, 12698049, 12763842, 12829635, 12895428, 12961221, 13027014, 13092807, 13158600, 13224393, 13290186, 13355979, 13421772, 13487565, 13553358, 13619151, 13684944, 13750737, 13816530, 13882323, 13948116, 14013909, 14079702, 14145495, 14211288, 14277081, 14342874, 14408667, 14474460, 14540253, 14606046, 14671839, 14737632, 14803425, 14869218, 14935011, 15000804, 15066597, 15132390, 15198183, 15263976, 15329769, 15395562, 15461355, 15527148, 15592941, 15658734, 15724527, 15790320, 15856113, 15921906, 15987699, 16053492, 16119285, 16185078, 16250871, 16316664, 16382457, 16448250, 16514043, 16579836, 16645629, 16711422, 16448250] ("256 gray scale") u32[] [16448250, 16711422, 16645629, 16579836, 16514043, 16448250, 16382457, 16316664, 16250871, 16185078, 16119285, 16053492, 15987699, 15921906, 15856113, 15790320, 15724527, 15658734, 15592941, 15527148, 15461355, 15395562, 15329769, 15263976, 15198183, 15132390, 15066597, 15000804, 14935011, 14869218, 14803425, 14737632, 14671839, 14606046, 14540253, 14474460, 14408667, 14342874, 14277081, 14211288, 14145495, 14079702, 14013909, 13948116, 13882323, 13816530, 13750737, 13684944, 13619151, 13553358, 13487565, 13421772, 13355979, 13290186, 13224393, 13158600, 13092807, 13027014, 12961221, 12895428, 12829635, 12763842, 12698049, 12632256, 12566463, 12500670, 12434877, 12369084, 12303291, 12237498, 12171705, 12105912, 12040119, 11974326, 11908533, 11842740, 11776947, 11711154, 11645361, 11579568, 11513775, 11447982, 11382189, 11316396, 11250603, 11184810, 11119017, 11053224, 10987431, 10921638, 10855845, 10790052, 10724259, 10658466, 10592673, 10526880, 10461087, 10395294, 10329501, 10263708, 10197915, 10132122, 10066329, 10000536, 9934743, 9868950, 9803157, 9737364, 9671571, 9605778, 9539985, 9474192, 9408399, 9342606, 9276813, 9211020, 9145227, 9079434, 9013641, 8947848, 8882055, 8816262, 8750469, 8684676, 8618883, 8553090, 8487297, 8421504, 8355711, 8289918, 8224125, 8158332, 8092539, 8026746, 7960953, 7895160, 7829367, 7763574, 7697781, 7631988, 7566195, 7500402, 7434609, 7368816, 7303023, 7237230, 7171437, 7105644, 7039851, 6974058, 6908265, 6842472, 6776679, 6710886, 6645093, 6579300, 6513507, 6447714, 6381921, 6316128, 6250335, 6184542, 6118749, 6052956, 5987163, 5921370, 5855577, 5789784, 5723991, 5658198, 5592405, 5526612, 5460819, 5395026, 5329233, 5263440, 5197647, 5131854, 5066061, 5000268, 4934475, 4868682, 4802889, 4737096, 4671303, 4605510, 4539717, 4473924, 4408131, 4342338, 4276545, 4210752, 4144959, 4079166, 4013373, 3947580, 3881787, 3815994, 3750201, 3684408, 3618615, 3552822, 3487029, 3421236, 3355443, 3289650, 3223857, 3158064, 3092271, 3026478, 2960685, 2894892, 2829099, 2763306, 2697513, 2631720, 2565927, 2500134, 2434341, 2368548, 2302755, 2236962, 2171169, 2105376, 2039583, 1973790, 1907997, 1842204, 1776411, 1710618, 1644825, 1579032, 1513239, 1447446, 1381653, 1315860, 1250067, 1184274, 1118481, 1052688, 986895, 921102, 855309, 789516, 723723, 657930, 592137, 526344, 460551, 394758, 328965, 263172, 197379, 131586, 65793, 16777222] ("256 gray scale inverse")] -> w1961
                    tunnel: [_ "Inverse"] -> w1959
                    tunnel: [u32 16448250 ("text color(black)") u32 0 ("text color(black)")] -> w1962
                    frame False {
                    }
                    frame True {
                    }
                  }
                  n763 = Unbundle By Name(w2036) -> ("Magnification"=w2005:sgl, "Pixel size"=w2004:sgl, "Working distance"=w2003:sgl, "EHT"=w2002:sgl)
                  n764 = case shown="False" w1988 {
                    tunnel: w2066 -> [w2121 w2124]
                    tunnel: w2065 -> [w2120 w2123]
                    tunnel: [w2119 w2122] -> w2064
                    tunnel: w1957 -> [w2118 _]
                    frame False {
                      n765 = Build Array (concatenate)(w2121, w2120, w2118) -> (w2119:u8[][])
                    }
                    frame True {
                      n766 = Build Array (concatenate)(w2124, w2123) -> (w2122:u8[][])
                    }
                  }
                  n767 = local read "File name"() -> (w2076:path)
                  n768 = case shown="13" w2044 {
                    tunnel: w2043 -> [w2129 _ w2132 _ w2134 _ w2140 _ w2143 _ w2148 _ w2153 _ w2160]
                    tunnel: w2042 -> [_ w2130 w2131 _ _ w2137 w2139 _ _ w2145 w2147 _ _ w2156 w2159]
                    tunnel: w2016 -> [_ _ _ w2133 w2135 w2136 w2138 _ _ _ _ w2150 w2152 w2155 w2158]
                    tunnel: w2012 -> [_ _ _ _ _ _ _ w2141 w2142 w2144 w2146 w2149 w2151 w2154 w2157]
                    tunnel: [w2129 w2130 w2132 w2133 w2134 w2137 w2140 w2141 w2143 w2145 w2148 w2150 w2153 w2156 w2160] -> w2023
                    tunnel: [_ _ w2131 _ w2135 w2136 w2139 _ w2142 w2144 w2147 w2149 w2152 w2155 w2159] -> w2022
                    tunnel: [_ _ _ _ _ _ w2138 _ _ _ w2146 _ w2151 w2154 w2158] -> w2021
                    tunnel: [_ _ _ _ _ _ _ _ _ _ _ _ _ _ w2157] -> w2020
                    frame 1, Default {
                    }
                    frame 2 {
                    }
                    frame 3 {
                    }
                    frame 4 {
                    }
                    frame 5 {
                    }
                    frame 6 {
                    }
                    frame 7 {
                    }
                    frame 8 {
                    }
                    frame 9 {
                    }
                    frame 10 {
                    }
                    frame 11 {
                    }
                    frame 12 {
                    }
                    frame 13 {
                    }
                    frame 14 {
                    }
                    frame 15 {
                    }
                  }
                  n769 = local read "Sample ID"() -> (w1958:string)
                  n770 = call <vilib>:"Flatten Pixmap.vi"("colors"=u32[] [16777222, 65793, 131586, 197379, 263172, 328965, 394758, 460551, 526344, 592137, 657930, 723723, 789516, 855309, 921102, 986895, 1052688, 1118481, 1184274, 1250067, 1315860, 1381653, 1447446, 1513239, 1579032, 1644825, 1710618, 1776411, 1842204, 1907997, 1973790, 2039583, 2105376, 2171169, 2236962, 2302755, 2368548, 2434341, 2500134, 2565927, 2631720, 2697513, 2763306, 2829099, 2894892, 2960685, 3026478, 3092271, 3158064, 3223857, 3289650, 3355443, 3421236, 3487029, 3552822, 3618615, 3684408, 3750201, 3815994, 3881787, 3947580, 4013373, 4079166, 4144959, 4210752, 4276545, 4342338, 4408131, 4473924, 4539717, 4605510, 4671303, 4737096, 4802889, 4868682, 4934475, 5000268, 5066061, 5131854, 5197647, 5263440, 5329233, 5395026, 5460819, 5526612, 5592405, 5658198, 5723991, 5789784, 5855577, 5921370, 5987163, 6052956, 6118749, 6184542, 6250335, 6316128, 6381921, 6447714, 6513507, 6579300, 6645093, 6710886, 6776679, 6842472, 6908265, 6974058, 7039851, 7105644, 7171437, 7237230, 7303023, 7368816, 7434609, 7500402, 7566195, 7631988, 7697781, 7763574, 7829367, 7895160, 7960953, 8026746, 8092539, 8158332, 8224125, 8289918, 8355711, 8421504, 8487297, 8553090, 8618883, 8684676, 8750469, 8816262, 8882055, 8947848, 9013641, 9079434, 9145227, 9211020, 9276813, 9342606, 9408399, 9474192, 9539985, 9605778, 9671571, 9737364, 9803157, 9868950, 9934743, 10000536, 10066329, 10132122, 10197915, 10263708, 10329501, 10395294, 10461087, 10526880, 10592673, 10658466, 10724259, 10790052, 10855845, 10921638, 10987431, 11053224, 11119017, 11184810, 11250603, 11316396, 11382189, 11447982, 11513775, 11579568, 11645361, 11711154, 11776947, 11842740, 11908533, 11974326, 12040119, 12105912, 12171705, 12237498, 12303291, 12369084, 12434877, 12500670, 12566463, 12632256, 12698049, 12763842, 12829635, 12895428, 12961221, 13027014, 13092807, 13158600, 13224393, 13290186, 13355979, 13421772, 13487565, 13553358, 13619151, 13684944, 13750737, 13816530, 13882323, 13948116, 14013909, 14079702, 14145495, 14211288, 14277081, 14342874, 14408667, 14474460, 14540253, 14606046, 14671839, 14737632, 14803425, 14869218, 14935011, 15000804, 15066597, 15132390, 15198183, 15263976, 15329769, 15395562, 15461355, 15527148, 15592941, 15658734, 15724527, 15790320, 15856113, 15921906, 15987699, 16053492, 16119285, 16185078, 16250871, 16316664, 16382457, 16448250, 16514043, 16579836, 16645629, 16711422, 16448250] ("256 gray scale"), "8-bit pixmap"=w2064) -> ("image data"=w2061:T30)  [unwired: 4 in, 5 out]
                  n771 = Strip Path(path=w2076) -> (stripped path=w2075:path, name=w2049:string)
                  n772 = call <vilib>:"Draw Flattened Pixmap.vi"("image data"=w2061) -> ("new picture"=w2063:picture)  [unwired: 1 in, 7 out]
                  n773 = Format Into String(format string="%s\n%s,  %s\nScan Rate = %.3pHz", w2049, w1958, w1959, w1954) -> (resulting string=w2048:string)  [unwired: 2 in, 1 out]
                  n774 = Search and Replace String(input string=w2049, search string=".dat", replace string=".png" ("replace string (\"\")")) -> (result string=w2072:string)  [unwired: 1 in, 7 out]
                  n775 = call <vilib>:"Draw Text at Point.vi"("text color(black)"=w1962, "text"=w2048, "origin"=cluster{"x":i16, "y":i16} {"x"=10, "y"=0}, "picture"=w2063) -> ("new picture"=w2051:picture)  [unwired: 5 in, 2 out]
                  n776 = local read "X resolution"() -> (w2053:u32)
                  n777 = local read "Y resolution"() -> (w2054:u32)
                  n778 = Build Path(base path=w2075, name or relative path=w2072) -> (appended path=w2071:path)
                  n779 = call <vilib>:"Flatten Pixmap.vi"("colors"=w1961, "8-bit pixmap"=w1955) -> ("image data"=w1989:T30)  [unwired: 4 in, 5 out]
                  n780 = case shown="False" w1988 {
                    tunnel: w1989 -> [w2106 _]
                    frame False {
                      n781 = local read "Tile index"() -> (w2115:u8[])
                      n782 = Index Array(array=w2115) -> (element #1=w2116:u8, element #2=w2117:u8)  [unwired: 2 in]
                      n783 = Format Into String(w2116) -> (resulting string=w2114:string)  [unwired: 3 in, 1 out]
                      n784 = Format Into String(w2117) -> (resulting string=w2112:string)  [unwired: 3 in, 1 out]
                      n785 = Concatenate Strings("Primary_grid_" ("string"), w2114, "-" ("string"), w2112, ".png" ("string")) -> (w2111:string)
                      n786 = Build Path(base path=path "D:/3D FIB-SEM Files" ("path to PNG file"), name or relative path=w2111) -> (appended path=w2107:path)
                      n787 = call <vilib>:"Write PNG File.vi"("image data"=w2106, "path to PNG file"=w2107) -> ()  [unwired: 1 in, 9 out]
                    }
                    frame True {
                    }
                  }
                  n788 = Format Into String(format string="Mag = %5.1f X\nPixel Size = %5.1f nm\n%#g x %#g pixels", w2005, w2004, w2053, w2054) -> (resulting string=w2047:string)  [unwired: 2 in, 1 out]
                  n789 = call <vilib>:"Draw Text at Point.vi"("text color(black)"=w1962, "text"=w2047, "origin"=cluster{"x":i16, "y":i16} {"x"=230, "y"=0}, "picture"=w2051) -> ("new picture"=w2060:picture)  [unwired: 5 in, 2 out]
                  n790 = local read "DetA-Scaling"() -> (w1952:sgl)
                  n791 = local read "DetB-Scaling"() -> (w1951:sgl)
                  n792 = Format Into String(format string="WD = %#g mm\nEHT = %#g kV\nDetA/B e- Scaling = %#g / %#g", w2003, w2002, w1952, w1951) -> (resulting string=w2056:string)  [unwired: 2 in, 1 out]
                  n793 = call <vilib>:"Draw Text at Point.vi"("text color(black)"=w1962, "text"=w2056, "origin"=cluster{"x":i16, "y":i16} {"x"=350, "y"=0}, "picture"=w2060) -> ("new picture"=w2027:picture)  [unwired: 5 in, 2 out]
                  n794 = call <vilib>:"Draw Text at Point.vi"("text color(black)"=w1962, "text"=w2023, "origin"=cluster{"x":i16, "y":i16} {"x"=10, "y"=45}, "picture"=w2027) -> ("new picture"=w2026:picture)  [unwired: 5 in, 2 out]
                  n795 = call <vilib>:"Draw Text at Point.vi"("text color(black)"=w1962, "text"=w2022, "origin"=cluster{"x":i16, "y":i16} {"x"=522, "y"=45}, "picture"=w2026) -> ("new picture"=w2025:picture)  [unwired: 5 in, 2 out]
                  n796 = call <vilib>:"Draw Text at Point.vi"("text color(black)"=w1962, "text"=w2021, "origin"=cluster{"x":i16, "y":i16} {"x"=1034, "y"=45}, "picture"=w2025) -> ("new picture"=w2024:picture)  [unwired: 5 in, 2 out]
                  n797 = call <vilib>:"Draw Text at Point.vi"("text color(black)"=w1962, "text"=w2020, "origin"=cluster{"x":i16, "y":i16} {"x"=1546, "y"=45}, "picture"=w2024) -> ("new picture"=w2028:picture)  [unwired: 5 in, 2 out]
                  n798 = call <vilib>:"Picture to Pixmap.vi"("picture"=w2028) -> ("image data"=w1966:T30)  [unwired: 3 in, 7 out]
                  n799 = call <vilib>:"Unflatten Pixmap.vi"("image data"=w1966) -> ("24-bit pixmap"=w1965:u32[][])  [unwired: 4 in, 6 out]
                  n800 = call <vilib>:"Flatten Pixmap.vi"("colors"=w1961, "8-bit pixmap"=w1965) -> ("image data"=w1967:T30)  [unwired: 4 in, 5 out]
                  n801 = call <vilib>:"Write PNG File.vi"("image data"=w1967, "path to PNG file"=w2071) -> ()  [unwired: 1 in, 9 out]
                }
              }
            }
            frame #4 {
              n802 = local read "Upload"() -> (w2200:bool)
              n803 = case shown="True" w2200 {
                frame False {
                }
                frame True {
                  n804 = stacked-sequence {
                    frame #0 {
                      n805 = shared-variable ".\\Zeiss Library.lvlib\\Upload flags path"() -> (w2201:string)  [unwired: 1 in, 1 out]
                      n806 = String To Path(string=w2201) -> (path=w2202:path)
                      "Upload flags path" <- w2202
                      n807 = File/Directory Info(path=w2202) -> (path out=w2205:path, error out=w2203:errorcluster)  [unwired: 1 in, 5 out]
                      n808 = Unbundle By Name(w2203) -> ("status"=w2204:bool)
                      n809 = case shown="True" w2204 {
                        tunnel: w2205 -> [_ w2206]
                        frame False {
                        }
                        frame True {
                          n810 = Create Folder(path (use dialog)=w2206) -> ()  [unwired: 1 in, 4 out]
                        }
                      }
                    }
                    frame #1 {
                      w2214 = T17 3 items=["no dialog", "OK message", "continue or stop message", "OK message + warnings", "continue/stop + warnings"] ("type of dialog (OK msg:1)")
                      w2226 = "^" ("replace string (\"\")")
                      n811 = local read "Upload flags path"() -> (w2217:path)
                      n812 = local read "File name"() -> (w2223:path)
                      n813 = local read "Delete after upload"() -> (w2210:bool)
                      n814 = Path To String(path=w2223) -> (string=w2222:string)
                      n815 = Select(t="^delete" ("replace string (\"\")"), s=w2210, f="^keep" ("replace string (\"\")")) -> (s? t:f=w2207:string)
                      n816 = Search and Replace String(replace all?=TRUE ("replace all? (F)"), input string=w2222, search string="\\", replace string=w2226) -> (result string=w2227:string)  [unwired: 4 in, 3 out]
                      n817 = local read "Sample ID"() -> (w2220:string)
                      n818 = Search and Replace String(input string=w2227, search string=":", replace string=w2226) -> (result string=w2219:string)  [unwired: 5 in, 3 out]
                      n819 = Concatenate Strings(w2220, "^" ("string"), w2219, w2207) -> (w2221:string)
                      n820 = Build Path(base path=w2217, name or relative path=w2221) -> (appended path=w2216:path)
                      n821 = Open/Create/Replace File(file path (use dialog)=w2216, operation (0:open)=T16."replace or create") -> (refnum out=w2213:refnum<file>, error out=w2211:errorcluster)  [unwired: 1 in, 4 out]
                      n822 = Close File(refnum=w2213, error in=w2211) -> (error out=w2212:errorcluster)  [unwired: 1 out]
                      n823 = call <vilib>:"General Error Handler.vi"("type of dialog (OK msg:1)"=w2214, "error in (no error)"=w2212) -> ()  [unwired: 1 in, 13 out]
                    }
                  }
                }
              }
            }
          }
        }
      }
      n824 = flat-sequence {
        tunnel: w762 -> [_]
        frame #0 {
          w932 = T17 3 items=["no dialog", "OK message", "continue or stop message", "OK message + warnings", "continue/stop + warnings"] ("type of dialog (OK msg:1)")
          w928 = 0 items=["one channel for each line", "one channel for all lines"] ("line grouping")
          n825 = shared-variable "My Computer\\Zeiss Library.lvlib\\Machine Type"() -> (w925:u8)  [unwired: 1 in, 1 out]
          n826 = case shown="2" w925 {
            frame 0, Default {
              n827 = local read "Eanable COM"() -> (w937:bool)
              n828 = case shown="True" w937 {
                frame False {
                }
                frame True {
                  w949 = TRUE ("Initialization")
                  n829 = local read "COM port"() -> (w946:refnum<visa-resource-name>)
                  n830 = call "Remcon32 command.vi"("Initialization"=w949, "SEM command"="bblk 1" ("write buffer"), "COM port in"=w946) -> ("error out"=w948:errorcluster, "COM port out"=w947:refnum<visa-resource-name>)  [unwired: 2 in, 5 out]
                  n831 = call "Remcon32 command.vi"("error in"=w948, "SEM command"="edx 0" ("write buffer"), "COM port in"=w947) -> ("error out"=w941:errorcluster, "COM port out"=w939:refnum<visa-resource-name>)  [unwired: 2 in, 5 out]
                  n832 = call "Remcon32 command.vi"("error in"=w941, "SEM command"="bblk 1" ("write buffer"), "COM port in"=w939) -> ("error out"=w942:errorcluster, "COM port out"=w940:refnum<visa-resource-name>)  [unwired: 2 in, 5 out]
                  n833 = local read "Freeze"() -> (w944:bool)
                  n834 = case shown="True" w944 {
                    tunnel: w940 -> [w952 w956]
                    tunnel: w949 -> [w950 w955]
                    tunnel: w942 -> [w951 w954]
                    frame False {
                      n835 = call "Remcon32 command.vi"("Close session"=w950, "error in"=w951, "COM port in"=w952) -> ()  [unwired: 2 in, 7 out]
                    }
                    frame True {
                      n836 = call "Remcon32 command.vi"("Close session"=w955, "error in"=w954, "SEM command"="frez" ("write buffer"), "COM port in"=w956) -> ()  [unwired: 1 in, 7 out]
                    }
                  }
                }
              }
            }
            frame 2 {
              n837 = local read "Api"() -> (w966:refnum<k7>)
              n838 = local read "Freeze"() -> (w959:bool)
              n839 = invoke class="_EMApi" method="Set"(reference=w966, "lpszParam"="DP_BEAM_BLANKED", "vValue"=sgl 1.0) -> (reference out=w963:refnum<k7>, error out=w962:errorcluster)  [unwired: 2 in, 3 out]
              n840 = invoke class="_EMApi" method="Set"(reference=w963, error in=w962, "lpszParam"="DP_EXT_SCAN_CONTROL" ("lpszCommand"), "vValue"=sgl 0.0) -> (reference out=w958:refnum<k7>, error out=w957:errorcluster)  [unwired: 1 in, 3 out]
              n841 = case shown="True" w959 {
                tunnel: w958 -> [_ w968]
                tunnel: w957 -> [_ w967]
                frame False {
                }
                frame True {
                  n842 = invoke class="_EMApi" method="Execute"(reference=w968, error in=w967, "lpszCommand"="CMD_FREEZE_ALL") -> ()  [unwired: 1 in, 4 out]
                }
              }
            }
          }
          n843 = local read "Detector FIB-NI auto switch"() -> (w936:tag)
          n844 = call-poly <vilib>:"DAQmx Create Virtual Channel.vi"("lines"=w936, "line grouping"=w928) -> ("task out"=w926:refnum<k21>, "error out"=w927:errorcluster)  [unwired: 3 in, 9 out]
          n845 = call <vilib>:"DAQmx Start Task.vi"("task/channels in"=w926, "error in"=w927) -> ("task out"=w929:refnum<k21>, "error out"=w930:errorcluster)  [unwired: 12 out]
          n846 = call-poly <vilib>:"DAQmx Write.vi"("task/channels in"=w929, "data"=FALSE, "error in"=w930) -> ("task out"=w934:refnum<k21>, "error out"=w935:errorcluster)  [unwired: 1 in, 10 out]
          n847 = call <vilib>:"DAQmx Clear Task.vi"("task in"=w934, "error in"=w935) -> ("error out"=w933:errorcluster)  [unwired: 13 out]
          n848 = call <vilib>:"Simple Error Handler.vi"("type of dialog (OK msg:1)"=w932, "error in (no error)"=w933) -> ()  [unwired: 8 out]
        }
      }
      n849 = Get Queue Status(queue=w811, error in (no error)=w810) -> (queue out=w813:refnum<queue>, error out=w814:errorcluster, # elements in queue=w815:i32)  [unwired: 6 out]
      n850 = Merge Errors(w765, w762, w770) -> (w761:errorcluster)
      "error out" <- w761
      n851 = Equal To 0?(x=w815) -> (x = 0?=w816:bool)
      n852 = case shown="True" w776 {
        tunnel: w775 -> [_ w970]
        frame False {
        }
        frame True {
          n853 = Set Occurrence(w970) -> ()
        }
      }
      n854 = case shown="False" w829 {
        tunnel: w818 -> [w2230 _]
        tunnel: w817 -> [w2229 _]
        frame False {
          n855 = Release Queue(queue=w2230, error in (no error)=w2229) -> ()  [unwired: 4 out]
        }
        frame True {
        }
      }
      n856 = call <vilib>:"Clear Errors.vi"("error in (no error)"=w761) -> ()  [unwired: 5 in, 2 out]
      n857 = Compound Arithmetic op=OR(w816, w812) -> (w807:bool)
      n858 = case shown="True" w807 {
        tunnel: w813 -> [_ w988]
        tunnel: w814 -> [w985 w987]
        tunnel: [w985 w986] -> _
        frame False {
        }
        frame True {
          n859 = Release Queue(queue=w988, error in (no error)=w987) -> (error out=w986:errorcluster)  [unwired: 3 out]
        }
      }
      n860 = case shown="False" w807 {
        tunnel: w809 -> [w984 _]
        tunnel: w808 -> [w983 _]
        frame False {
          n861 = Release Queue(queue=w984, error in (no error)=w983) -> ()  [unwired: 4 out]
        }
        frame True {
        }
      }
    }
    frame #3 {
      n862 = local read "Det A Img"() -> (w2271:i16[][])
      n863 = local read "Det B Img"() -> (w2265:i16[][])
      n864 = Array Size(array=w2271) -> (size(s)=w2269:i32[])
      n865 = Array Size(array=w2265) -> (size(s)=w2267:i32[])
      n866 = Multiply Array Elements(1:w2269) -> (0:w2270:i32)
      n867 = Multiply Array Elements(1:w2267) -> (0:w2266:i32)
      n868 = local read "Options"() -> (w2281:T9)
      n869 = Reshape Array(w2271, w2270) -> (w2272:i16[])
      n870 = Reshape Array(w2265, w2266) -> (w2264:i16[])
      n871 = Array Max & Min(array=w2272) -> (max value=w2268:i16)  [unwired: 3 out]
      n872 = Array Max & Min(array=w2264) -> (max value=w2263:i16)  [unwired: 3 out]
      n873 = Unbundle By Name(w2281) -> ("8-bit"=w2278:bool, "Detector A"=w2277:bool, "Detector B"=w2276:bool)
      n874 = Greater?(x=w2268, y=u8 255) -> (0:w2282:bool)
      n875 = Greater?(x=w2263, y=u8 255) -> (0:w2280:bool)
      n876 = Compound Arithmetic op=AND(w2278, w2277, w2282) -> (w2275:bool)
      n877 = Compound Arithmetic op=AND(w2278, w2276, w2280) -> (w2274:bool)
      n878 = Build Array(w2275, w2274) -> (→"8-bit over scale":bool[])
    }
    frame #4 {
      n879 = local read "Tile index"() -> (w2284:u8[])
      n880 = local write "stop"(TRUE ("stop")) -> ()
      n881 = local write "Force tclk init"(FALSE ("Force tclk init")) -> ()
      n882 = shared-variable ".\\Zeiss Library.lvlib\\Completed tile index"(w2284) -> ()  [unwired: 1 in, 1 out]
    }
  }
